vi "reg_visu OPC1.vi"(7 "object_name":string="GM1", 9 "Останов\nпрограммы":bool) -> ()   [LabVIEW 2019]
uses:
  projects/Additivs/Regulators/PROG/GM1_201007/enums/AI.ctl
  Heating/ctl/general_init_client.ctl
  OPC/OPC UA Client.ctl
  <vilib>/OPCUA/controls/OPC UA Client Refnum.ctl
  <vilib>/OPCUA/controls/NodeId.ctl
  <vilib>/OPCUA/controls/NodeIds.ctl
  <vilib>/OPCUA/controls/Subscription ID.ctl
  <vilib>/OPCUA/controls/Write Variant Request.ctl
  <vilib>/OPCUA/controls/Write Status.ctl
  <vilib>/OPCUA/controls/Subscription Data Change.ctl
  <vilib>/OPCUA/controls/Data Type.ctl
  <vilib>/OPCUA/controls/OPC UA StatusCode.ctl
  Database/ctl/Coninfo.ctl
  Inputs/Ctl/AI short.ctl
  Inputs/Ctl/Parameter State.ctl
  Inputs/Ctl/DI short.ctl
  Alarms/Ctl/ALRs_State.ctl
  projects/Additivs/Regulators/PROG/GM1_201007/enums/KFM.ctl
  projects/Additivs/Regulators/PROG/GM1_201007/enums/PAR.ctl
  projects/Additivs/Regulators/PROG/GM1_201007/enums/DI.ctl
  projects/Additivs/Regulators/PROG/GM1_201007/enums/DI_FAST.ctl
  projects/Additivs/Regulators/PROG/GM1_201007/enums/AO.ctl
  projects/Additivs/Regulators/PROG/GM1_201007/enums/DO.ctl
  projects/Additivs/Regulators/PROG/GM1_201007/enums/ALR.ctl
  projects/Additivs/Regulators/PROG/GM1_201007/enums/System.ctl
  ctl/Y_short.ctl
  Inputs/Ctl/Parameter State short.ctl
  ctl/Ys_short.ctl
  <vilib>/picture/picture.llb/imagedata.ctl
  Reg visu/Reg visu.lvclass
  Reg visu/Reg visu.lvclass/Reg visu.ctl
  Inputs/Ctl/ParamColumns.ctl
  531d0f69-163a-4f16-9a14-c53a50917fc8.vi
  cf2ac22c-c8a5-4ec0-ba3c-9dae82546773.vi
  <vilib>/NI/AMC/Create Single Message.vi
  <vilib>/NI/AMC/Update Message Routing Info.vi
  <vilib>/NI/AMC/Read Termination Message.vi
  <vilib>/JDP Science/JSONtext/Find Multiple Items.vi
  <vilib>/JDP Science/JSONtext/String Subset.vi
  <vilib>/JDP Science/JSONtext/support/Strip Quotes and Unescape.vi
  <vilib>/JDP Science/JSONtext/support/Unescape JSON string.vi
  <vilib>/Utility/config.llb/Read Key (String).vi
  <vilib>/OPCUA/client/Multiple Read String Array.vi
  <vilib>/OPCUA/client/Multiple Read ByteString Array.vi
  Reg visu/Run.vi
  Heating/Global stop.vi
  <vilib>/NI/AMC/Send Message.vi
  <vilib>/NI/AMC/Globals.vi
  <vilib>/OPCUA/client/Multiple Read String.vi
  <vilib>/JDP Science/JSONtext/JSON text to Variant.vi
  <vilib>/OPCUA/client/Multiple Write Variant.vi
  <vilib>/JDP Science/JSONtext/Parsing/Parse Full Path or Item Name.vi
  <vilib>/JDP Science/JSONtext/Offset/Find Item Locations by Path.vi
  <vilib>/JDP Science/JSONtext/Get Array Elements.vi
  <vilib>/JDP Science/JSONtext/LVClass Serializer/JSONtext LVClass Serializer.lvclass
  Heating/ctl/Z_State.ctl
  Heating/Heating.lvlib
  Heating/ctl/Y_state.ctl
  Heating/ctl/Y_source.ctl
  Heating/ctl/ZM_State.ctl
  <vilib>/NI/AMC/AMC.lvlib
  <vilib>/OPCUA/NI OPC UA Client.lvlib
  Database/PostgreSQL.lvlib
  <vilib>/Utility/config.llb/NI_LVConfig.lvlib
  projects/Additivs/Regulators/PROG/GM1_201007/enums/Param_h0gm1.lvlib
  Inputs/Inputs.lvlib
  control.lvlib
  OPC/OPC addons.lvlib
  Alarms/Alarms.lvlib
  Heating/ctl/ZY_control.ctl
  Alarms/Ctl/ALR_Status_short.ctl
  Heating/ctl/Y_short.ctl
  Heating/ctl/Z.ctl
  Heating/ctl/ZY_state_short.ctl
  projects/Additivs/Regulators/PROG/GM1_201007/enums/scada_prog_state.ctl
  Heating/ctl/YQ2/YQ2.xctl
  Heating/ctl/Z_OnSwitch/Z_OnSwitch.xctl
  Heating/ctl/ZY_state_OPC.ctl
  7b03969a-a950-4454-9689-61267dd49491.vi
  fdeea6ee-2705-42e7-9783-53477a0f0781.vi
  00ce5b65-c19c-4f2f-b5a6-2d8b920d64b8.vi
  d49def32-a249-4c88-86f5-dd42ff10ee1e.vi
  847353ff-c4dc-4a0d-82d8-8a8c8b1dd027.vi
  96cb8638-67ee-45ab-9e65-4cb433c703bb.vi
  5d0f38f1-9d99-409f-81fc-f0eb7cf3d60e.vi
  fe7cfdb3-b4e0-46ae-bded-47b821cc5e2e.vi
  96416696-a13a-4191-9eaf-5b72f20cf204.vi
  <vilib>/OPCUA/client/Multiple Read Int32 Array.vi
  <vilib>/OPCUA/client/Multiple Read Double Array.vi
  <vilib>/OPCUA/client/Multiple Read UInt32 Array.vi
  <vilib>/OPCUA/client/Multiple Read Bool Array.vi
  Userlib.lvlib
  Heating/ctl/Z_source.ctl
panel:
  in  "HT1 emergency stop":bool caption="Аварийный сброс"
  in  "Reset":bool
  in  "Start":bool
  out "PV 2":dbl(slide) scale=0.0..50.0 scale format="%#_4g"
  in  "tick":u32=100 caption="Время цикла основной программы" min=5 max=1000 step=1
  out "EB3BP1_XQ01":dbl caption="kPa" format="%#.1f"
  in  "AI_enum":T1
  out "CPU %":dbl(slide) scale=0.0..100.0
  in  "password system DB":string
  in  "message name":string="AI redefine"
  in  "process":bool
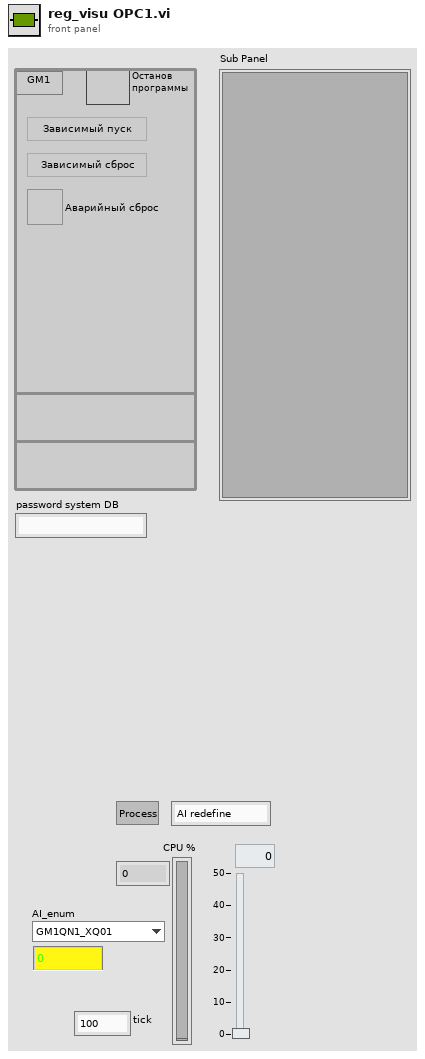
[diagram p1: front panel]
types:
  T1 = typedef "Param_h0gm1.lvlib/AI.ctl" = enum16{"GM1QN1_XQ01", "GM1QN2_XQ01", "GM1QN3_XQ01", "GM1QN4_XQ01", "GM1QN5_XQ01", "GM1QN6_XQ01", "GM1QN7_XQ01", "GM1QN8_XQ01", "GM1QN9_XQ01", "GM1QN10_XQ01", "GM1QN11_XQ01", "GM1QN12_XQ01", "GM1QN13_XQ01", "GM1QN14_XQ01", "GM1QN15_XQ01", "GM1QN16_XQ01", "GM1QN17_XQ01", "GM1QN18_XQ01", "GM1QN19_XQ01", "GM1QN20_XQ01", "GM1QN21_XQ01", "GM1QN22_XQ01", "GM1QN23_XQ01", "GM1QN1_XQ02", "GM1QN2_XQ02", "GM1QN3_XQ02", "GM1QN4_XQ02", "GM1QN5_XQ02", "GM1QN6_XQ02", "GM1QN7_XQ02", "GM1QN8_XQ02", "GM1QN9_XQ02", "GM1QN10_XQ02", "GM1QN11_XQ02", "GM1QN12_XQ02", "GM1QN13_XQ02", "GM1QN14_XQ02", "GM1QN15_XQ02", "GM1QN16_XQ02", "GM1QN17_XQ02", "GM1QN18_XQ02", "GM1QN19_XQ02", "GM1QN20_XQ02", "GM1QN21_XQ02", "GM1QN22_XQ02", "GM1QN23_XQ02"}
  T2 = typedef "Heating.lvlib/general_init_client.ctl" = enum16{"Init Data", "Init TMPs", "Read system DB param", "Read data DB param", "Read OPC param", "Read Enums", "Read Reg param", "Connect to OPC", "Read Param", "Read AI param", "AI references", "AI reorder", "AI reorder1", "AI Descriptions", "AI Descriptions1", "Read DI param", "Read AO param", "Read DO param", "Read ALR param", "Read control param", "Read state param", "Init save progs", "Init ALR Listbox symbols", "Init Y defs", "Init Shared Variables", "Exit"}
  T3 = typedef "AMC.lvlib/Message Queue.ctl" = refnum<queue>
  T4 = typedef "Inputs.lvlib/AI short.ctl" = cluster{"AI":dbl[], "AIState":T5[], "AIALRState":errorcluster[]}
  T5 = typedef "Inputs.lvlib/Parameter State.ctl" = cluster{"code":i32, "visible":bool, "color":u32, "source":string}
  T6 = typedef "NodeIds.ctl" = T7[]
  T7 = typedef "NodeId.ctl" = string
  T8 = typedef "Inputs.lvlib/DI short.ctl" = cluster{"DI":bool[], "DI_State":T5[], "DI_ALRState":errorcluster[]}
  T9 = typedef "Alarms.lvlib/ALRs_State.ctl" = cluster{"ALR not block":bool[], "ALR":bool[], "ALR blocked":bool[], "ALR ON":bool[], "code":i32[], "level":i32[][], "t ms":u32[], "ack state":enum32{"not", "tripped", "reset", "ack"}[], "color":u32[]}
  T10 = typedef "control.lvlib/Y_short.ctl" = cluster{"Y_Source":u8, "Y_SetState":u8, "SP_Set":dbl, "SP":dbl, "PV":dbl, "PV_State":T11, "Y_preSet":dbl, "Y_Set":dbl, "Y":dbl, "Y_State":T11, "YB":bool}
  T11 = typedef "Inputs.lvlib/Parameter State short.ctl" = cluster{"code":i32, "visible":bool, "color":u32}
  T12 = cluster{"connect":bool, "gas":string, "Y_State":T10}
  T13 = cluster{"name":string, "OPC port":string, "security policy":cluster{"message mode":enum16{"None", "Sign", "Sign and Encrypt"}, "security":enum16{"Basic256", "Basic128Rsa15"}}}
  T14 = cluster{"KFM":string[], "PAR":string[], "AI":string[], "DI":string[], "DI_fast":string[], "AO":string[], "DO":string[], "ALR":string[], "System":string[]}
  T15 = typedef "PostgreSQL.lvlib/Coninfo.ctl" = cluster{"host":string, "port":string, "client_encoding":string, "dbname":string, "user":string, "password":string}
  T16 = typedef "OPC addons.lvlib/OPC UA Client.ctl" = cluster{"Client refnum":T17, "Folders":T7[], "node IDs":T6, "subscription IDs":T18[], "requests":T19[], "data change event":refnum<user-event>, "Event Reg":refnum<event-registration>}
  T17 = typedef "OPC UA Client Refnum.ctl" = refnum<k21>
  T18 = typedef "Subscription ID.ctl" = u32
  T19 = typedef "Write Variant Request.ctl" = cluster{"node ID":T7, "value":variant, "timestamp (current time)":timestamp, "node status":T20}
  T20 = typedef "Write Status.ctl" = u32
  T21 = cluster{"object_name":string, "Server":cluster{"name":string, "OPC port":string, "security policy":cluster{"message mode":enum16{"None", "Sign", "Sign and Encrypt"}, "security":enum16{"Basic256", "Basic128Rsa15"}}}, "Enums":cluster{"KFM":string[], "PAR":string[], "AI":string[], "DI":string[], "DI_fast":string[], "AO":string[], "DO":string[], "ALR":string[], "System":string[]}, "OPC UA":T16, "system DB":T15, "AI_SHVR":refnum<k21>, "AI_Names_SHVR":refnum<k21>, "DI_SHVR":refnum<k21>, "DI_Names_SHVR":refnum<k21>, "ALR_state_SHRV":refnum<k21>, "ALR_Descriptions_SHRV":refnum<k21>, "CPU_utilization":refnum<k21>, "AI_refs":refnum<vi>[], "AI_Descriptions":string[], "DI_Descriptions":string[], "ALR_Descriptions":string[]}
  T22 = cluster{"AI_reorder_table":i32[], "AI":dbl[], "AIState":T5[], "AIALRState":errorcluster[], "DI_reorder_table":i32[], "DI":bool[], "DI_State":T5[], "ALR_State":T9, "ALR_Names":string[], "RegsParam":dbl[][], "Regs_Descriptions":string[][], "system msg":string}
  T23 = typedef "NI_LVConfig.lvlib/Config Data RefNum.ctl" = refnum<k1>
  T24 = typedef "Param_h0gm1.lvlib/System.ctl" = enum16{"GM3HT1", "GM3HT2", "EB2TB1", "EB2TB2", "EB2TB3", "EB3TB1", "EB3TB2", "EB3TB3"}
  T25 = typedef "Param_h0gm1.lvlib/ALR.ctl" = enum16{"GM1JBA1JA1_CONN", "GM1JBA1JA2_CONN", "GM1JBA2JA1_CONN", "GM1JBA2JA2_CONN", "GM1JBA3JA1_CONN", "GM1QN1XQ01_SERR", "GM1QN2XQ01_SERR", "GM1QN3XQ01_SERR", "GM1QN4XQ01_SERR", "GM1QN5XQ01_SERR", "GM1QN6XQ01_SERR", "GM1QN7XQ01_SERR", "GM1QN8XQ01_SERR", "GM1QN9XQ01_SERR", "GM1QN10XQ01_SERR", "GM1QN11XQ01_SERR", "GM1QN12XQ01_SERR", "GM1QN13XQ01_SERR", "GM1QN14XQ01_SERR", "GM1QN15XQ01_SERR", "GM1QN16XQ01_SERR", "GM1QN17XQ01_SERR", "GM1QN18XQ01_SERR", "GM1QN19XQ01_SERR", "GM1QN20XQ01_SERR", "GM1QN21XQ01_SERR", "GM1QN22XQ01_SERR", "GM1QN23XQ01_SERR"}
  T26 = typedef "Param_h0gm1.lvlib/DO.ctl" = enum16{"GM1FZ1_YB47"}
  T27 = typedef "Param_h0gm1.lvlib/AO.ctl" = enum16{"GM1QN1_YQ01", "GM1QN2_YQ01", "GM1QN3_YQ01", "GM1QN4_YQ01", "GM1QN5_YQ01", "GM1QN6_YQ01", "GM1QN7_YQ01", "GM1QN8_YQ01", "GM1QN9_YQ01", "GM1QN10_YQ01", "GM1QN11_YQ01", "GM1QN12_YQ01", "GM1QN13_YQ01", "GM1QN14_YQ01", "GM1QN15_YQ01", "GM1QN16_YQ01", "GM1QN17_YQ01", "GM1QN18_YQ01", "GM1QN19_YQ01", "GM1QN20_YQ01", "GM1QN21_YQ01", "GM1QN22_YQ01", "GM1QN23_YQ01"}
  T28 = typedef "Param_h0gm1.lvlib/DI_FAST.ctl" = enum16{"W1.KF_XB01", "W1.KF_XB02", "W1.KF_XB03", "W1.KF_XB04", "W1.KF_XB05", "W1.KF_XB06", "W1.KF_XB07", "W1.KF_XB08", "W1.KF_XB09", "W1.KF_XB10", "W1.KF_XB11", "W1.KF_XB12", "W1.KF_XB13", "W1.KF_XB14", "W1.KF_XB15", "W1.KF_XB16"}
  T29 = typedef "Param_h0gm1.lvlib/DI.ctl" = enum16{"GM1FZ1_XB19"}
  T30 = typedef "Param_h0gm1.lvlib/PAR.ctl" = enum16{"GM1QN1_alr_value", "GM1QN1_auto_value", "GM1QN1_output_set_time", "GM1QN1_group", "GM1QN1_process_gas", "GM1QN2_alr_value", "GM1QN2_auto_value", "GM1QN2_output_set_time", "GM1QN2_group", "GM1QN2_process_gas", "GM1QN3_alr_value", "GM1QN3_auto_value", "GM1QN3_output_set_time", "GM1QN3_group", "GM1QN3_process_gas", "GM1QN4_alr_value", "GM1QN4_auto_value", "GM1QN4_output_set_time", "GM1QN4_group", "GM1QN4_process_gas", "GM1QN5_alr_value", "GM1QN5_auto_value", "GM1QN5_output_set_time", "GM1QN5_group", "GM1QN5_process_gas", "GM1QN6_alr_value", "GM1QN6_auto_value", "GM1QN6_output_set_time", "GM1QN6_group", "GM1QN6_process_gas", "GM1QN7_alr_value", "GM1QN7_auto_value", "GM1QN7_output_set_time", "GM1QN7_group", "GM1QN7_process_gas", "GM1QN8_alr_value", "GM1QN8_auto_value", "GM1QN8_output_set_time", "GM1QN8_group", "GM1QN8_process_gas", "GM1QN9_alr_value", "GM1QN9_auto_value", "GM1QN9_output_set_time", "GM1QN9_group", "GM1QN9_process_gas", "GM1QN10_alr_value", "GM1QN10_auto_value", "GM1QN10_output_set_time", "GM1QN10_group", "GM1QN10_process_gas", "GM1QN11_alr_value", "GM1QN11_auto_value", "GM1QN11_output_set_time", "GM1QN11_group", "GM1QN11_process_gas", "GM1QN12_alr_value", "GM1QN12_auto_value", "GM1QN12_output_set_time", "GM1QN12_group", "GM1QN12_process_gas", "GM1QN13_alr_value", "GM1QN13_auto_value", "GM1QN13_output_set_time", "GM1QN13_group", "GM1QN13_process_gas", "GM1QN14_alr_value", "GM1QN14_auto_value", "GM1QN14_output_set_time", "GM1QN14_group", "GM1QN14_process_gas", "GM1QN15_alr_value", "GM1QN15_auto_value", "GM1QN15_output_set_time", "GM1QN15_group", "GM1QN15_process_gas", "GM1QN16_alr_value", "GM1QN16_auto_value", "GM1QN16_output_set_time", "GM1QN16_group", "GM1QN16_process_gas", "GM1QN17_alr_value", "GM1QN17_auto_value", "GM1QN17_output_set_time", "GM1QN17_group", "GM1QN17_process_gas", "GM1QN18_alr_value", "GM1QN18_auto_value", "GM1QN18_output_set_time", "GM1QN18_group", "GM1QN18_process_gas", "GM1QN19_alr_value", "GM1QN19_auto_value", "GM1QN19_output_set_time", "GM1QN19_group", "GM1QN19_process_gas", "GM1QN20_alr_value", "GM1QN20_auto_value", "GM1QN20_output_set_time", "GM1QN20_group", "GM1QN20_process_gas", "GM1QN21_alr_value", "GM1QN21_auto_value", "GM1QN21_output_set_time", "GM1QN21_group", "GM1QN21_process_gas", "GM1QN22_alr_value", "GM1QN22_auto_value", "GM1QN22_output_set_time", "GM1QN22_group", "GM1QN22_process_gas", "GM1QN23_alr_value", "GM1QN23_auto_value", "GM1QN23_output_set_time", "GM1QN23_group", "GM1QN23_process_gas"}
  T31 = typedef "Param_h0gm1.lvlib/KFM.ctl" = enum16{"GM1KF1_A1", "GM1JBA1_JA1", "GM1JBA1_JA2", "GM1JBA2_JA1", "GM1JBA2_JA2", "GM1JBA3_JA1"}
  T32 = cluster{"message mode":enum16{"None", "Sign", "Sign and Encrypt"}, "security":enum16{"Basic256", "Basic128Rsa15"}}
  T33 = typedef "OPC addons.lvlib/OPC tag.ctl" = cluster{"name":string, "data type":T34, "access level":T35, "description":string, "period":T36}
  T34 = typedef "Data Type.ctl" = u16
  T35 = typedef "OPC addons.lvlib/Access level.ctl" = enum16{"none", "read-only", "write-only", "read/write"}
  T36 = typedef "OPC addons.lvlib/Period.ctl" = enum16{"on_load", "100 ms", "500 ms", "1 s"}
  T37 = cluster{"sampling interval":dbl, "queue size":u32, "discard oldest":bool, "data change filter":cluster{"trigger":enum32{"Status", "StatusValue", "StatusValueTimestamp"}, "deadband type":enum32{"None", "Absolute", "Percent"}, "deadband value":dbl}}[]
  T38 = cluster{"Read Access":enum8{"Allowed", "Required", "None"}, "Write Access":enum8{"Allowed", "Required", "None"}}
  T39 = typedef "OPC UA StatusCode.ctl" = u32
  T40 = cluster{"node ID":T7, "values ":string[], "timestamp":timestamp, "status":T39}[]
  T41 = cluster{"node ID":T7, "values ":string[], "timestamp":timestamp, "status":T39}
  T42 = cluster{"node ID":T7, "values ":u8[][], "timestamp":timestamp, "status":T39}[]
  T43 = cluster{"node ID":T7, "values ":u8[][], "timestamp":timestamp, "status":T39}
  T44 = typedef "Heating.lvlib/ZY_control.ctl" = cluster{"Z_HSw":u8, "Z_HSetState":T45, "Y_HSw":u8, "Y_HSetState":T46, "SP":dbl, "Y_H":dbl, "Reset_ALR":bool}
  T45 = typedef "Heating.lvlib/Z_State.ctl" = enum8{"initialization", "alarm", "disabled", "not ready", "stop ready", "reserv", "switched off", "reserv2", "switched on", "check", "on min", "decrease out", "on", "increase out", "on max"}
  T46 = typedef "Heating.lvlib/Y_state.ctl" = enum8{"initialize", "alarm", "min", "stop", "hand", "auto", "max"}
  T47 = typedef "Heating.lvlib/ZY_state_short.ctl" = cluster{"Z":T48, "Y":T51, "ALR_Status":T53[]}
  T48 = typedef "Heating.lvlib/Z.ctl" = cluster{"Z_Source":T49, "Z_SetState":T45, "Z_State":T45, "Z_State_T":u32, "ZM_State":T50, "ZM_State_T":u32, "ALR  L1":bool, "ALR  L2":bool, "HH_run":u64}
  T49 = typedef "Heating.lvlib/Z_source.ctl" = enum8{"initialize", "local disabled", "local hand", "hand", "auto", "dist"}
  T50 = typedef "Heating.lvlib/ZM_State.ctl" = enum8{"initialization", "stop", "start_cmd", "contactor_on_cmd", "heating", "on", "stop_cmd", "power_down", "contactor_off_cmd", "cooling", "restart_delay"}
  T51 = typedef "Heating.lvlib/Y_short.ctl" = cluster{"Y_Source":T52, "Y_SetState":T46, "SP_Set":dbl, "SP":dbl, "PV":dbl, "Y_Set":dbl, "Y":dbl, "Y_State":T11, "YB":bool}
  T52 = typedef "Heating.lvlib/Y_source.ctl" = enum8{"initialize", "local disabled", "local hand", "hand", "auto", "dist"}
  T53 = typedef "Alarms.lvlib/ALR_Status_short.ctl" = cluster{"status":bool, "code":i32, "level":i32}
  T54 = cluster{"connect":bool, "gas":string, "Y_State":T10}[]
  T55 = typedef "imagedata.ctl" = cluster{"image type":i32, "image depth":i32, "image":u8[], "mask":u8[], "colors":u32[], "Rectangle":cluster{"left":i16, "top":i16, "right":i16, "bottom":i16}}
  T56 = typedef "AMC.lvlib/Message.ctl" = cluster{"name":string, "value":string, "attributes":T57, "receiver host":string, "receiver process":string, "source host":string, "source process":string, "priority message":bool, "acknowledge message":bool}
  T57 = typedef "Tools_KeyedArray.lvlib/KeyedArray.ctl" = cluster{"keys":string[], "values":string[]}
  T58 = cluster{"node ID":T7, "value ":string, "timestamp":timestamp, "status":T39}[]
  T59 = typedef "Inputs.lvlib/ParamColumns.ctl" = enum16{"value", "value_range_min", "value_range_max", "d", "fname", "value_units", "fcode", "fcodef", "fcode_full"}
  T60 = typedef "Param_h0gm1.lvlib/scada_prog_state.ctl" = enum16{"ReadAIParam", "ReadAIParam1", "ReadDIParam", "AI", "AI1", "AIValues", "AIValues1", "DI", "DiValues", "Alarms", "Messages", "TB1", "TB2", "TB3", "Control EB3", "Outputs", "Exit"}
  T61 = cluster{"connect":bool, "Z_Source":T52, "Z_State_heating":T45}
  T62 = typedef "Heating.lvlib/ZY_state_OPC.ctl" = cluster{"Z":cluster{"Z_Source":u8, "Z_SetState":u8, "Z_State":u8, "Z_State_T":u32, "ZM_State":u8, "ZM_State_T":u32, "ALR  L1":bool, "ALR  L2":bool, "HH_run":i32}, "Y":cluster{"Y_Source":u8, "Y_SetState":u8, "SP_Set":dbl, "SP":dbl, "PV":dbl, "Y_Set":dbl, "Y":dbl, "Y_State":cluster{"code":i32, "visible":bool, "color":u32}, "YB":bool}, "ALR_Status":cluster{"status":bool, "code":i32, "level":i32}[]}
  T63 = typedef "Heating.lvlib/ZY_state_short.ctl" = cluster{"Z":T64, "Y":T51, "ALR_Status":T53[]}
  T64 = typedef "Heating.lvlib/Z.ctl" = cluster{"Z_Source":T52, "Z_SetState":T45, "Z_State":T45, "Z_State_T":u32, "ZM_State":T50, "ZM_State_T":u32, "ALR  L1":bool, "ALR  L2":bool, "HH_run":i32}
  T65 = cluster{"node ID":T7, "values ":dbl[], "timestamp":timestamp, "status":T39}[]
  T66 = cluster{"node ID":T7, "values ":i32[], "timestamp":timestamp, "status":T39}[]
  T67 = cluster{"node ID":T7, "values ":dbl[], "timestamp":timestamp, "status":T39}
  T68 = cluster{"node ID":T7, "values ":i32[], "timestamp":timestamp, "status":T39}
  T69 = cluster{"node ID":T7, "values ":bool[], "timestamp":timestamp, "status":T39}[]
  T70 = cluster{"node ID":T7, "values ":bool[], "timestamp":timestamp, "status":T39}
  T71 = cluster{"node ID":T7, "values ":u32[], "timestamp":timestamp, "status":T39}[]
  T72 = cluster{"node ID":T7, "values ":u32[], "timestamp":timestamp, "status":T39}
  T73 = cluster{"node ID":T7, "value ":string, "timestamp":timestamp, "status":T39}
  T74 = typedef "Heating.lvlib/ZY_state_short.ctl" = cluster{"Z":T64, "Y":T75, "ALR_Status":T53[]}
  T75 = typedef "Heating.lvlib/Y_short.ctl" = cluster{"Y_Source":T52, "Y_SetState":T46, "SP_Set":dbl, "SP":dbl, "PV":dbl, "Y":dbl, "Y_State":T11, "YB":bool}
  T76 = enum32{"invalid app kind", "Development System", "Run Time System", "Student Edition", "Embedded LabVIEW", "Evaluation", "Custom"}
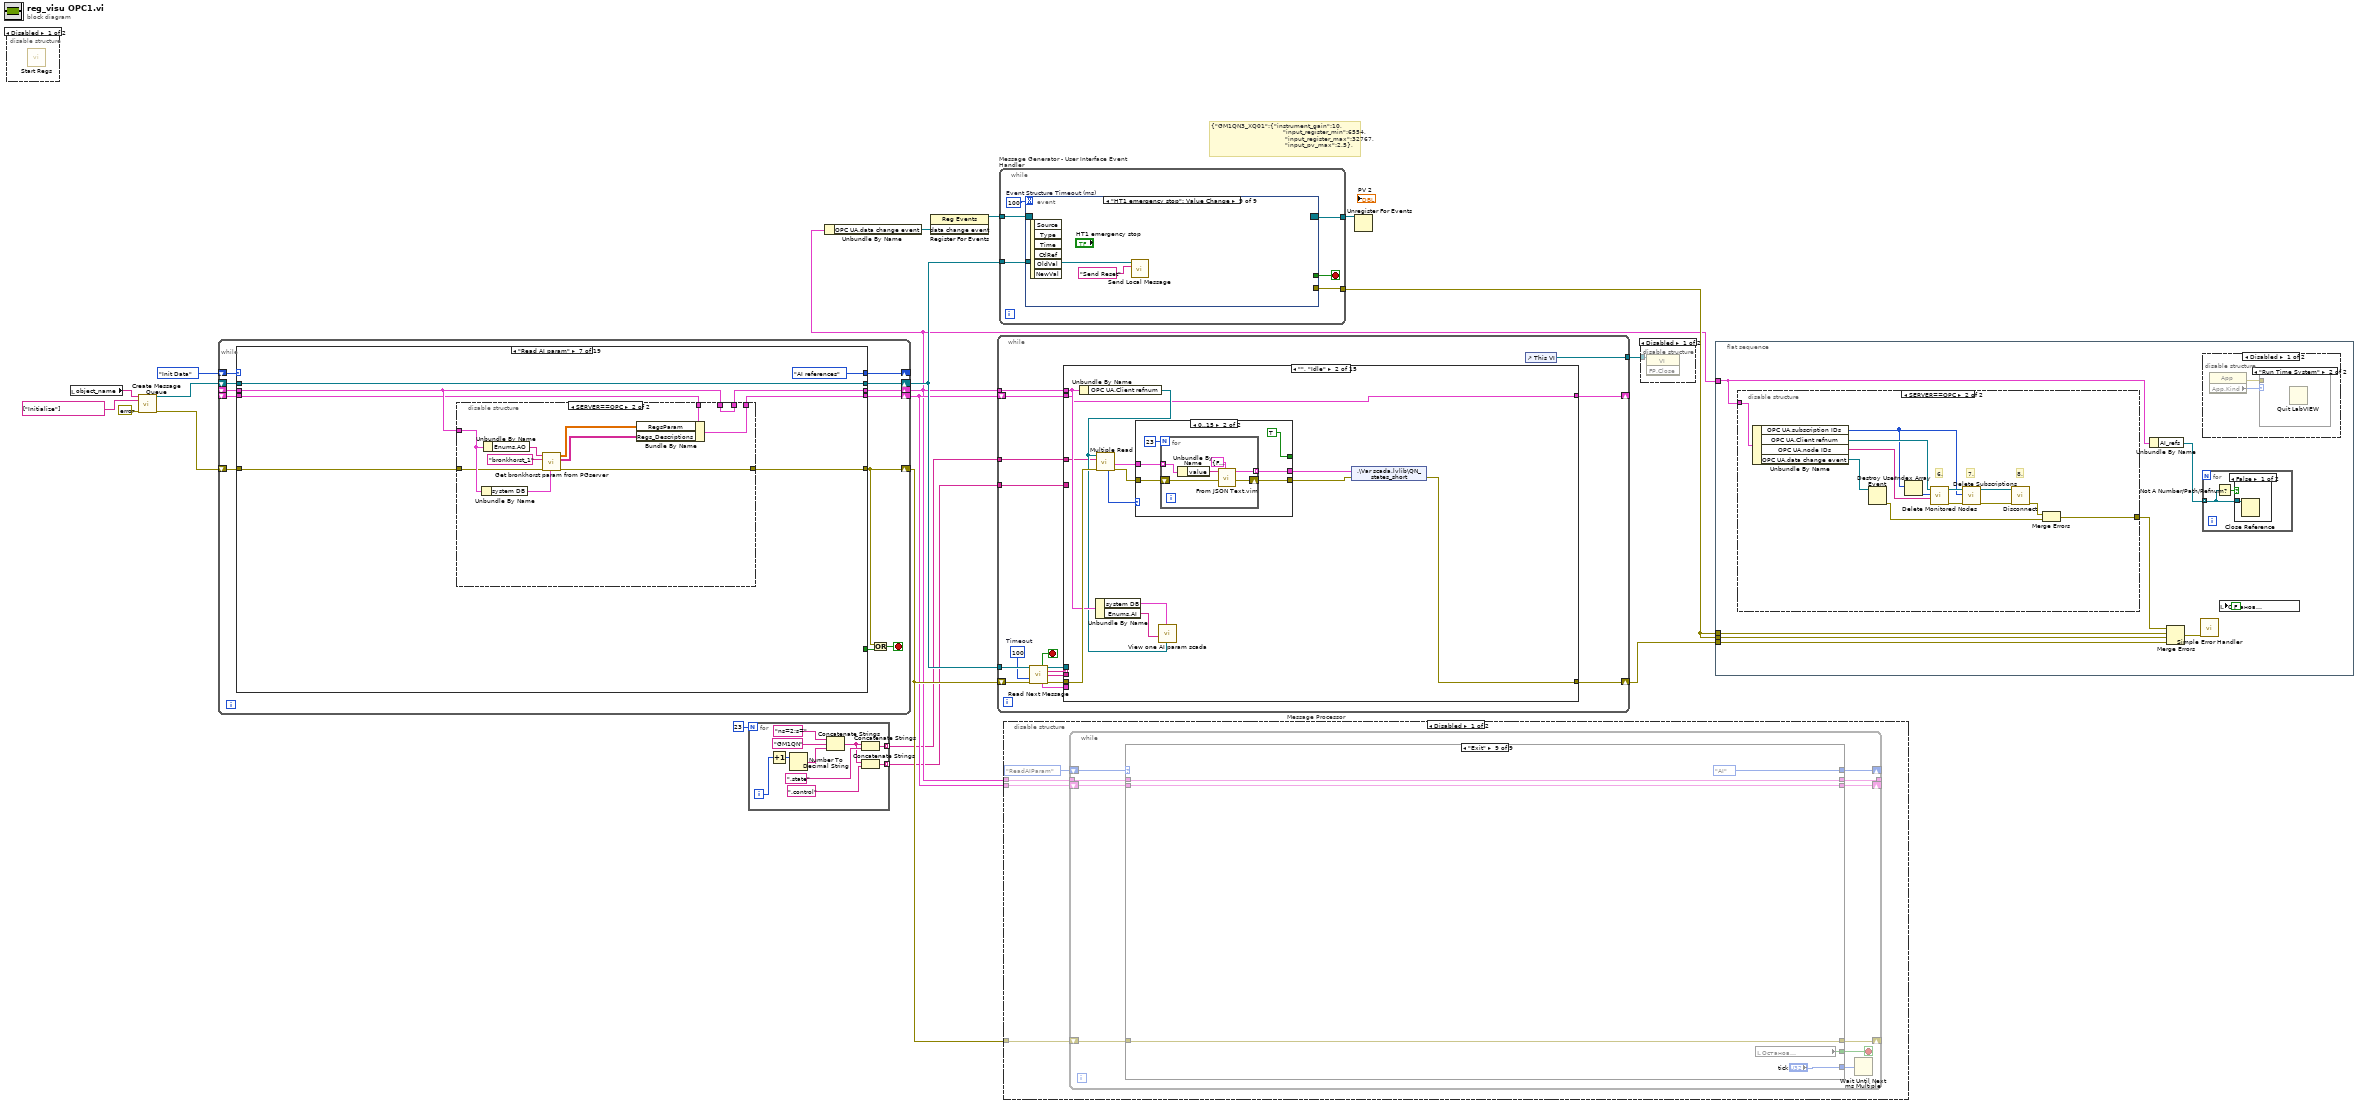
[diagram p0: block diagram]
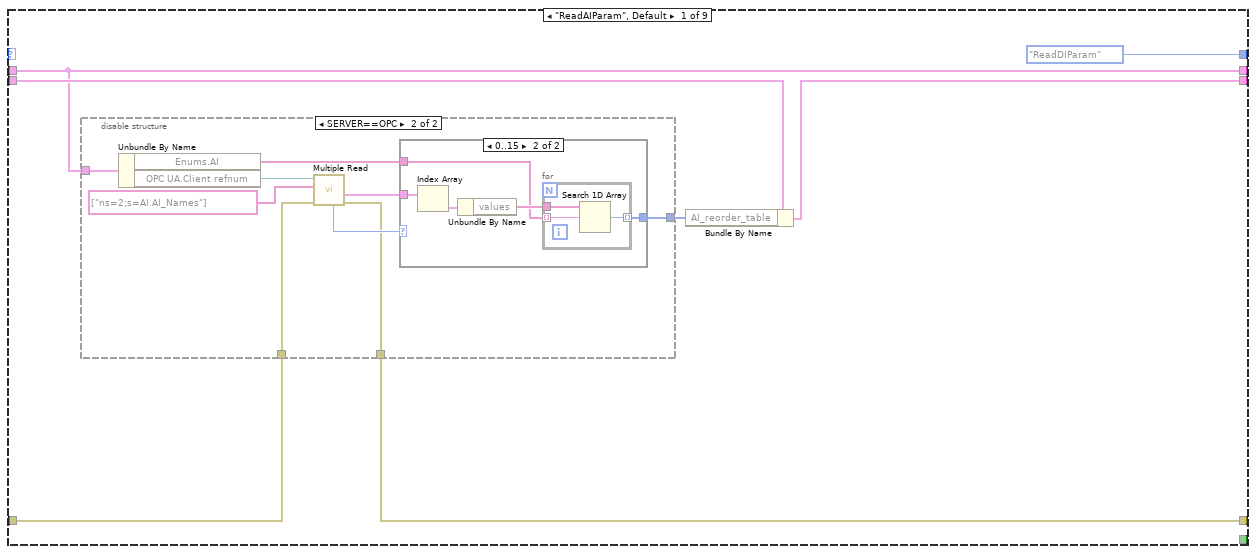
[diagram p3: hidden frame]
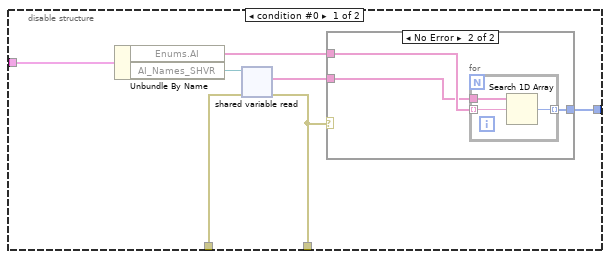
[diagram p4: hidden frame]
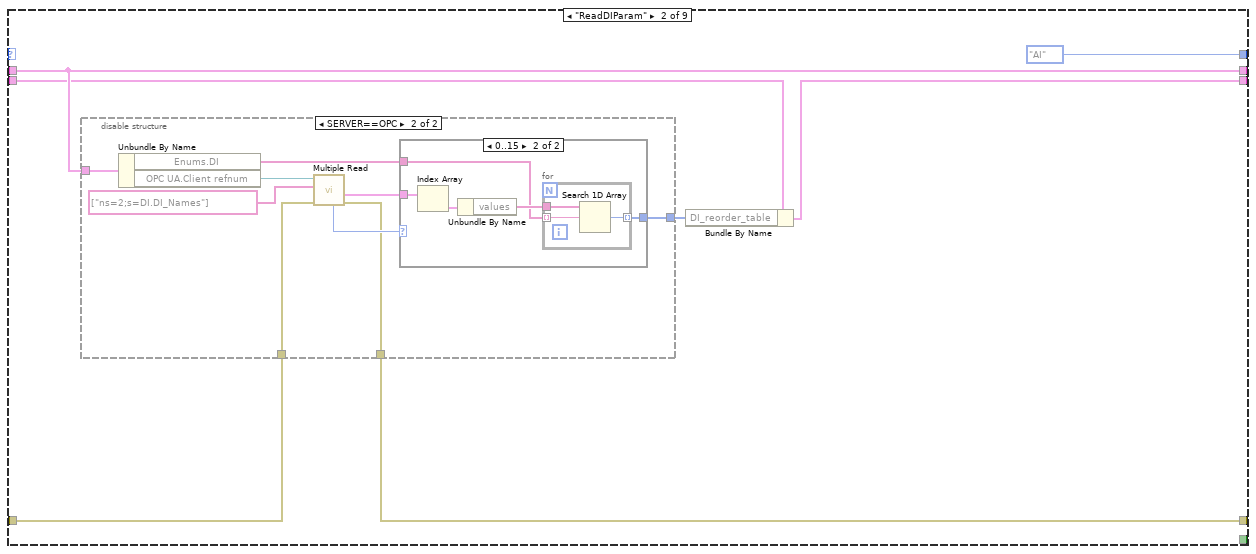
[diagram p7: hidden frame]
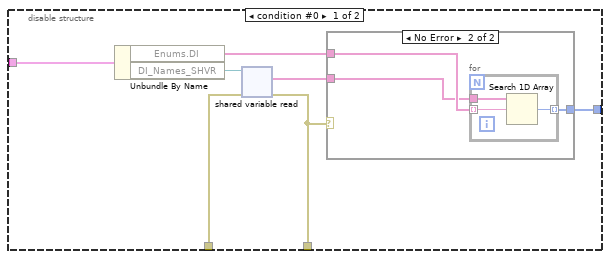
[diagram p8: hidden frame]
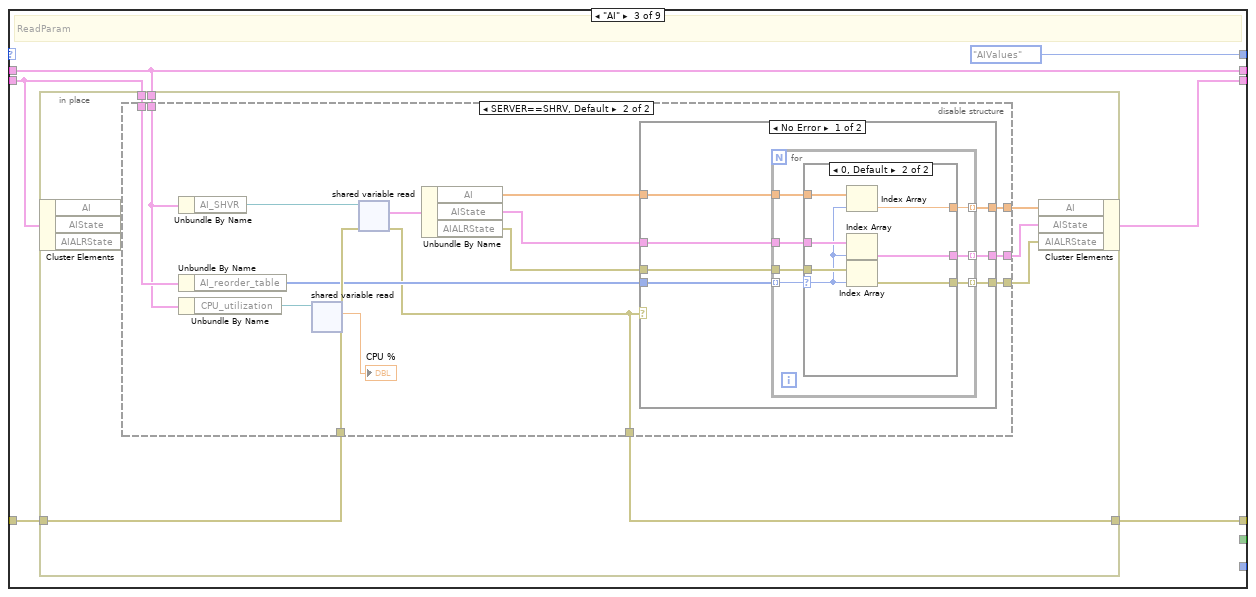
[diagram p11: hidden frame]
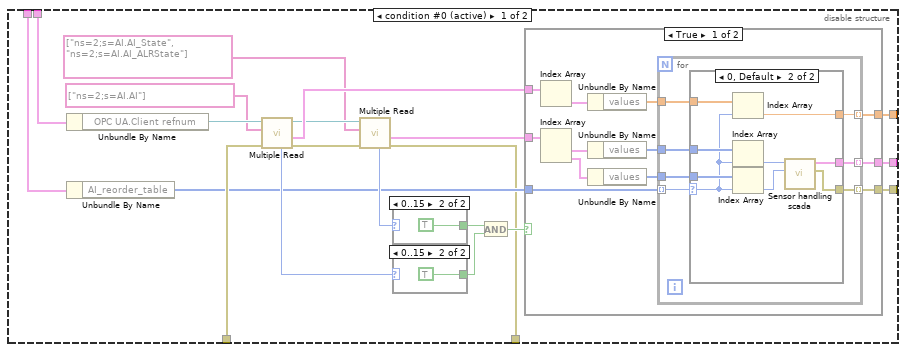
[diagram p12: hidden frame]
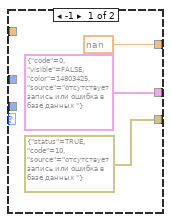
[diagram p15: hidden frame]
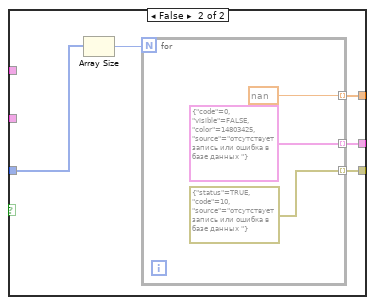
[diagram p16: hidden frame]
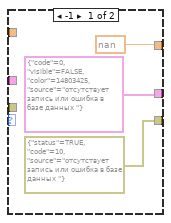
[diagram p17: hidden frame]
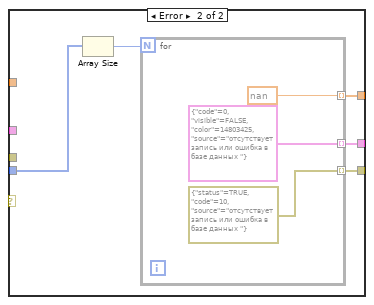
[diagram p18: hidden frame]
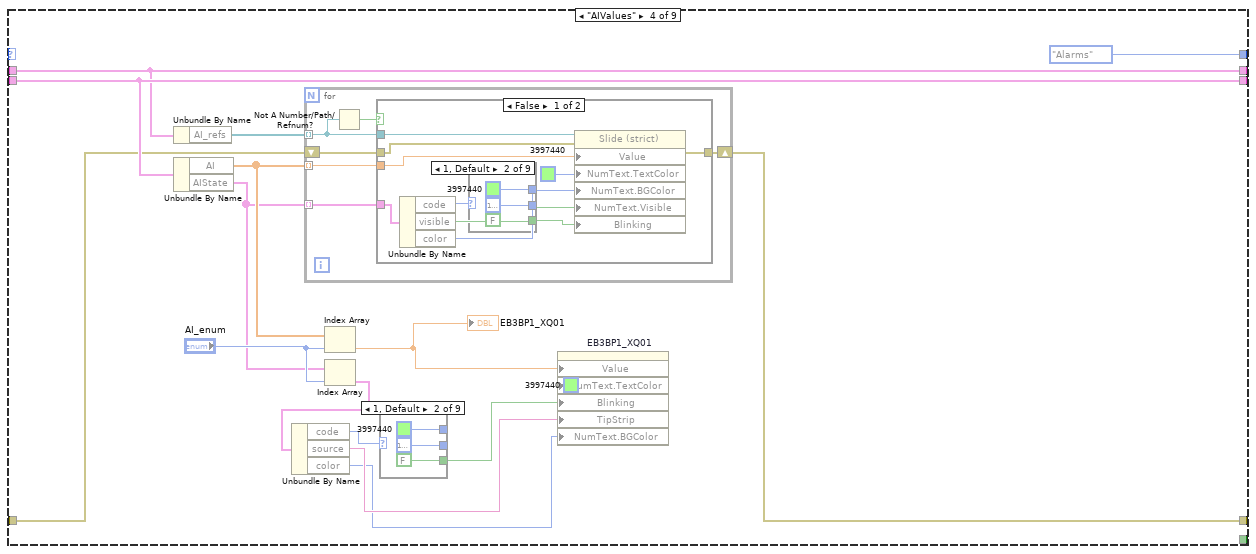
[diagram p19: hidden frame]
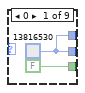
[diagram p20: hidden frame]
diagram:
  # "{\"GM1QN3_XQ01\":{\"instrument_gain\":10,\n                                    \"input_register_min\":6554,\n                                     \"input_register_max\":32767,\n                                     \"input_pv_max\":2.5},"
  n1 = disable-structure shown="Disabled" {
    frame Disabled {
      n2 = call "Start Regs.vi"() -> ()  [unwired: 11 in, 1 out]
    }
    frame Enabled {
    }
  }
  n3 = local read "object_name"() -> (w17:string)
  n4 = call <vilib>:"Create Message Queue.vi"("message queue name"=w17, "initial message names"=string[] ["Initialize"], "error in"=errorcluster {"status"=FALSE, "code"=0, "source"=""}) -> ("message queue out"=w10:T3, "error out"=w12:errorcluster)  [unwired: 11 in]
  n5 = while {
    shift-right: [w20] -> w6
    shift-left: w12 -> [w28]
    shift-right: [w31] -> w4
    shift-left: _ -> [w29]
    shift-right: [w27] -> _
    shift-left: general_init_client."Init Data" -> [w30]
    shift-right: [w24] -> w5
    shift-left: _ -> [w23]
    shift-right: [w21] -> w9
    shift-left: w10 -> [w22]
    stop <- w25 stop-if-true
    n6 = case shown="\"Read AI param\"" w30 {
      tunnel: [w50 w68 w70 w113 w176 w202 w239 w279 w291 w336 w356 w392 w435 w463 w493 w499 w516 w577 w580] -> w20
      selector: w30 -> [_ _ _ _ _ _ _ _ _ _ _ _ _ _ _ _ _ _ w583]
      tunnel: [w51 w66 w105 w114 w196 w203 w240 w276 w290 w330 w358 w393 w437 w465 w495 w512 w528 w578 w581] -> w31
      tunnel: w29 -> [_ w66 w104 w112 w198 w201 w238 w275 w290 w329 w355 w386 w434 w462 w495 w512 w528 w578 w581]
      tunnel: w28 -> [w50 w68 w106 w115 w186 w205 w241 w279 w292 w337 w359 w387 w438 w466 w492 w499 w518 w577 w580]
      tunnel: [general_init_client."Init TMPs" general_init_client."Read system DB param" general_init_client."Read data DB param" general_init_client."Read Enums" general_init_client."Read OPC param" general_init_client."Read Param" general_init_client."AI references" general_init_client."AI reorder" general_init_client."AI Descriptions" general_init_client."Read DI param" general_init_client."Read ALR param" general_init_client."Read control param" general_init_client."Read state param" general_init_client."Init Shared Variables" general_init_client."Init ALR Listbox symbols" general_init_client."Init Y defs" general_init_client."Exit" general_init_client."Init Data" w582] -> w27
      tunnel: [_ _ _ _ _ _ _ _ _ _ _ _ _ _ _ _ _ TRUE _] -> w26
      tunnel: [w48 w61 w108 w117 w200 w206 w237 w280 w289 w333 w357 w385 w436 w464 w498 w515 w527 w575 w585] -> w24
      tunnel: w23 -> [w48 _ w108 w117 w200 w206 w236 w280 w288 w333 w357 w384 w436 w464 w498 w515 w527 w575 w585]
      tunnel: w22 -> [w49 w67 w107 w116 w175 w204 w243 w282 w295 w342 w361 w395 w440 w468 w497 w514 w521 w574 w584]
      tunnel: [w49 w67 w107 w116 w175 w204 w243 w282 w295 w342 w361 w395 w440 w468 w497 w514 w521 w574 w584] -> w21
      frame "Init Data" {
        w33 = string[] []  # DI_Descriptions
        w34 = string[] []  # AI_Descriptions
        w32 = string[] []  # ALR_Descriptions
        w35 = refnum<vi>[] []  # AI_refs
        w36 = refnum<k21> refnum  # CPU_utilization
        w38 = refnum<k21> refnum  # ALR_Descriptions_SHRV
        w39 = refnum<k21> refnum  # ALR_state_SHRV
        w40 = refnum<k21> refnum  # DI_Names_SHVR
        w41 = refnum<k21> refnum  # DI_SHVR
        w42 = T13 {"name"="H1GM2", "OPC port"="49580", "security policy"={"message mode"=enum."None", "security"=enum."Basic256"}}  # Server
        w43 = refnum<k21> refnum  # AI_Names_SHVR
        w44 = refnum<k21> refnum  # AI_SHVR
        w46 = T14 {"KFM"=[], "PAR"=[], "AI"=[], "DI"=[], "DI_fast"=[], "AO"=[], "DO"=[], "ALR"=[], "System"=[]}  # Enums
        w47 = T15 {"host"="localhosh", "port"="5432", "client_encoding"="LATIN1", "dbname"="system", "user"="postgres", "password"=""}  # system DB
        w45 = T16 {"Client refnum"="", "Folders"=[], "node IDs"=[], "subscription IDs"=[], "requests"=[], "data change event"=refnum, "Event Reg"=refnum}  # OPC UA
        n7 = Bundle("object_name"="object_name", "Server"=w42, "Enums"=w46, "OPC UA"=w45, "system DB"=w47, "AI_SHVR"=w44, "AI_Names_SHVR"=w43, "DI_SHVR"=w41, "DI_Names_SHVR"=w40, "ALR_state_SHRV"=w39, "ALR_Descriptions_SHRV"=w38, "CPU_utilization"=w36, "AI_refs"=w35, "AI_Descriptions"=w34, "DI_Descriptions"=w33, "ALR_Descriptions"=w32) -> (w51:T21)  [unwired: 1 in]
      }
      frame "Init TMPs" {
        w53 = string[][] []  # Regs_Descriptions
        w55 = dbl[][] []  # RegsParam
        w56 = string[] []  # ALR_Names
        w57 = T9 {"ALR not block"=[], "ALR"=[], "ALR blocked"=[], "ALR ON"=[], "code"=[], "level"=[], "t ms"=[], "ack state"=[], "color"=[]}  # ALR_State
        w54 = ""  # system msg
        w58 = i32[] []  # DI_reorder_table
        w60 = i32[] []  # AI_reorder_table
        (unwired) dbl[] []  # AO
        (unwired) dbl[][] []  # AOP
        (unwired) bool[] []  # DO
        (unwired) i32[][] []  # DOP
        (unwired) i32[] []  # PAR_I
        (unwired) dbl[] []  # PAR
        (unwired) bool[] []  # connect
        w65 = T5[] []  # AIState
        w64 = errorcluster[] []  # AIALRState
        w63 = bool[] []  # DI
        (unwired) dbl[][] []  # DIP
        w62 = T5[] []  # DI_State
        (unwired) dbl[][] []  # AIP
        w59 = dbl[] []  # AI
        n8 = Bundle("AI_reorder_table"=w60, "AI"=w59, "AIState"=w65, "AIALRState"=w64, "DI_reorder_table"=w58, "DI"=w63, "DI_State"=w62, "ALR_State"=w57, "ALR_Names"=w56, "RegsParam"=w55, "Regs_Descriptions"=w53, "system msg"=w54) -> (w61:T22)  [unwired: 1 in]
      }
      frame "Read system DB param" {
        w81 = "System_DB" ("key")
        n9 = disable-structure shown="Default" {
          disable-tunnel: [w110 w111] -> w71
          frame condition #0 (active) {
            n10 = call <vilib>:"Application Directory.vi"() -> ("Application Directory"=w110:path)
          }
          frame condition #1 {
            n11 = call <vilib>:"Dflt Data Dir.vi"() -> ("App:Default Data Directory"=w111:path)
          }
        }
        n12 = Unbundle By Name(w104) -> ("system DB"=w95:T15)
        n13 = Unbundle By Name(w95) -> ("host"=w94:string, "port"=w93:string, "client_encoding"=w90:string, "dbname"=w85:string, "user"=w80:string)
        n14 = Build Path(base path=w71, name or relative path=path "DBp.ini" ("configuration file path")) -> (appended path=w103:path)
        n15 = call <vilib>:"Open Config Data.vi"("error in (no error)"=w106, "configuration file path"=w103) -> ("error out"=w101:errorcluster, "refnum"=w100:T23)  [unwired: 7 in, 1 out]
        n16 = call-poly <vilib>:"Read Key.vi"("section"=w81, "error in (no error)"=w101, "default value"=w94, "key"="host", "refnum"=w100) -> ("error out"=w96:errorcluster, "value"=w73:string, "refnum out"=w97:T23)  [unwired: 3 in, 1 out]
        n17 = call-poly <vilib>:"Read Key.vi"("section"=w81, "error in (no error)"=w96, "default value"=w93, "key"="port", "refnum"=w97) -> ("error out"=w89:errorcluster, "value"=w74:string, "refnum out"=w91:T23)  [unwired: 3 in, 1 out]
        n18 = call-poly <vilib>:"Read Key.vi"("section"=w81, "error in (no error)"=w89, "default value"=w90, "key"="clint_encoding", "refnum"=w91) -> ("error out"=w86:errorcluster, "value"=w75:string, "refnum out"=w87:T23)  [unwired: 3 in, 1 out]
        n19 = call-poly <vilib>:"Read Key.vi"("section"=w81, "error in (no error)"=w86, "default value"=w85, "key"="dbname", "refnum"=w87) -> ("error out"=w82:errorcluster, "value"=w76:string, "refnum out"=w83:T23)  [unwired: 3 in, 1 out]
        n20 = call-poly <vilib>:"Read Key.vi"("section"=w81, "error in (no error)"=w82, "default value"=w80, "key"="user", "refnum"=w83) -> ("error out"=w78:errorcluster, "value"=w77:string, "refnum out"=w79:T23)  [unwired: 3 in, 1 out]
        n21 = call <vilib>:"Close Config Data.vi"("error in (no error)"=w78, "refnum"=w79) -> ("error out"=w70:errorcluster)  [unwired: 8 in, 1 out]
        n22 = Bundle By Name(cluster=w104, "system DB.user"=w77, "system DB.dbname"=w76, "system DB.client_encoding"=w75, "system DB.port"=w74, "system DB.host"=w73, "system DB.password"="password system DB") -> (w105:T21)
      }
      frame "Read data DB param" {
        n23 = disable-structure shown="SERVER==OPC" {
          disable-tunnel: w115 -> [w158 w164]
          disable-tunnel: w112 -> [w156 w163]
          disable-tunnel: [w154 w163] -> w114
          disable-tunnel: [w123 w164] -> w113
          disable-tunnel: w112 -> [w150 _]
          frame condition #0 (active) {
            w135 = "Server" ("key")
            n24 = disable-structure shown="Default" {
              disable-tunnel: [w161 w162] -> w153
              frame condition #0 (active) {
                n25 = call <vilib>:"Application Directory.vi"() -> ("Application Directory"=w161:path)
              }
              frame condition #1 {
                n26 = call <vilib>:"Dflt Data Dir.vi"() -> ("App:Default Data Directory"=w162:path)
              }
            }
            n27 = Unbundle By Name(w150) -> ("Server.name"=w152:string, "Server.OPC port"=w149:string, "Server.security policy.message mode"=w138:enum16{"None", "Sign", "Sign and Encrypt"}, "Server.security policy.security"=w133:enum16{"Basic256", "Basic128Rsa15"})
            n28 = Build Path(base path=w153, name or relative path=path "DBp.ini" ("configuration file path")) -> (appended path=w160:path)
            n29 = call <vilib>:"Open Config Data.vi"("error in (no error)"=w158, "configuration file path"=w160) -> ("error out"=w137:errorcluster, "refnum"=w157:T23)  [unwired: 7 in, 1 out]
            n30 = call <userlib>:"Get Strings from Enum__ogtk.vi"("error in (no error)"=w137, "Enum"=w138) -> ("error out"=w127:errorcluster, "String Value"=w136:string)  [unwired: 6 in, 2 out]
            n31 = call <userlib>:"Get Strings from Enum__ogtk.vi"("error in (no error)"=w137, "Enum"=w133) -> ("error out"=w128:errorcluster, "String Value"=w134:string)  [unwired: 6 in, 2 out]
            n32 = call-poly <vilib>:"Read Key.vi"("section"=w135, "error in (no error)"=w137, "default value"=w152, "key"="name", "refnum"=w157) -> ("error out"=w146:errorcluster, "value"=w151:string, "refnum out"=w147:T23)  [unwired: 3 in, 1 out]
            n33 = call-poly <vilib>:"Read Key.vi"("section"=w135, "error in (no error)"=w146, "default value"=w149, "key"="OPC port", "refnum"=w147) -> ("error out"=w145:errorcluster, "value"=w144:string, "refnum out"=w143:T23)  [unwired: 3 in, 1 out]
            n34 = call-poly <vilib>:"Read Key.vi"("section"=w135, "error in (no error)"=w145, "default value"=w136, "key"="message mode", "refnum"=w143) -> ("error out"=w140:errorcluster, "value"=w130:string, "refnum out"=w142:T23)  [unwired: 3 in, 1 out]
            n35 = call-poly <vilib>:"Read Key.vi"("section"=w135, "error in (no error)"=w140, "default value"=w134, "key"="security ", "refnum"=w142) -> ("error out"=w139:errorcluster, "value"=w129:string, "refnum out"=w141:T23)  [unwired: 3 in, 1 out]
            n36 = call <vilib>:"Close Config Data.vi"("error in (no error)"=w139, "refnum"=w141) -> ("error out"=w124:errorcluster)  [unwired: 8 in, 1 out]
            n37 = Scan From String(input string=w129, error in=w128, default 1=enum16{"Basic256", "Basic128Rsa15"}."Basic256" ("Server.security policy.security")) -> (error out=w122:errorcluster, output 1=w126:enum16{"Basic256", "Basic128Rsa15"})  [unwired: 2 in, 2 out]
            n38 = Scan From String(input string=w130, error in=w127, default 1=enum16{"None", "Sign", "Sign and Encrypt"}."None" ("Server.security policy.message mode")) -> (error out=w121:errorcluster, output 1=w125:enum16{"None", "Sign", "Sign and Encrypt"})  [unwired: 2 in, 2 out]
            n39 = Bundle By Name(cluster=w156, "Server.security policy.security"=w126, "Server.security policy.message mode"=w125, "Server.OPC port"=w144, "Server.name"=w151) -> (w154:T21)
            n40 = Merge Errors(w124, w122, w121) -> (w123:errorcluster)
          }
          frame condition #1 {
          }
        }
      }
      frame "Read Enums" {
        w166 = System."GM3HT1"  # System_enum
        w167 = ALR."GM1JBA1JA1_CONN"  # ALR_enum
        w168 = DO."GM1FZ1_YB47"  # DO_enum
        w169 = AO."GM1QN1_YQ01"  # AO_enum
        w170 = DI_FAST."W1.KF_XB01"  # DI_enum fast
        w171 = DI."GM1FZ1_XB19"  # DI_enum
        w172 = AI."GM1QN1_XQ01"  # AI_enum
        w173 = PAR."GM1QN1_output_set_time"  # PAR_enum
        w174 = KFM."GM1JBA1_JA1"  # KFM_enum
        w195 = T14 {"KFM"=[], "PAR"=[], "AI"=[], "DI"=[], "DI_fast"=[], "AO"=[], "DO"=[], "ALR"=[], "System"=[]}  # Enums
        n41 = call <userlib>:"Get Strings from Enum__ogtk.vi"("error in (no error)"=w186, "Enum"=w174) -> ("error out"=w185:errorcluster, "Enum Strings"=w194:string[])  [unwired: 6 in, 2 out]
        n42 = call <userlib>:"Get Strings from Enum__ogtk.vi"("error in (no error)"=w186, "Enum"=w173) -> ("error out"=w184:errorcluster, "Enum Strings"=w193:string[])  [unwired: 6 in, 2 out]
        n43 = call <userlib>:"Get Strings from Enum__ogtk.vi"("error in (no error)"=w186, "Enum"=w172) -> ("error out"=w183:errorcluster, "Enum Strings"=w192:string[])  [unwired: 6 in, 2 out]
        n44 = call <userlib>:"Get Strings from Enum__ogtk.vi"("error in (no error)"=w186, "Enum"=w171) -> ("error out"=w182:errorcluster, "Enum Strings"=w191:string[])  [unwired: 6 in, 2 out]
        n45 = call <userlib>:"Get Strings from Enum__ogtk.vi"("error in (no error)"=w186, "Enum"=w170) -> ("error out"=w181:errorcluster, "Enum Strings"=w190:string[])  [unwired: 6 in, 2 out]
        n46 = call <userlib>:"Get Strings from Enum__ogtk.vi"("error in (no error)"=w186, "Enum"=w169) -> ("error out"=w180:errorcluster, "Enum Strings"=w189:string[])  [unwired: 6 in, 2 out]
        n47 = call <userlib>:"Get Strings from Enum__ogtk.vi"("error in (no error)"=w186, "Enum"=w168) -> ("error out"=w179:errorcluster, "Enum Strings"=w188:string[])  [unwired: 6 in, 2 out]
        n48 = call <userlib>:"Get Strings from Enum__ogtk.vi"("error in (no error)"=w186, "Enum"=w167) -> ("error out"=w178:errorcluster, "Enum Strings"=w187:string[])  [unwired: 6 in, 2 out]
        n49 = call <userlib>:"Get Strings from Enum__ogtk.vi"("error in (no error)"=w186, "Enum"=w166) -> ("error out"=w177:errorcluster)  [unwired: 6 in, 3 out]
        n50 = Bundle By Name(cluster=w195, "KFM"=w194, "PAR"=w193, "AI"=w192, "DI"=w191, "DI_fast"=w190, "AO"=w189, "DO"=w188, "ALR"=w187, "System"=string[] []) -> (w197:T14)
        n51 = Merge Errors(w185, w184, w183, w182, w181, w180, w179, w178, w177) -> (w176:errorcluster)
        n52 = Bundle By Name(cluster=w198, "Enums"=w197) -> (w196:T21)
      }
      frame "Read OPC param" {
        n53 = disable-structure shown="SERVER==OPC" {
          disable-tunnel: w205 -> [w228 w234]
          disable-tunnel: [w227 w235] -> w203
          disable-tunnel: [w209 w234] -> w202
          disable-tunnel: w201 -> [w221 w235]
          disable-tunnel: w201 -> [w213 _]
          frame condition #0 (active) {
            w229 = TRUE  # trust any server
            # "1."
            n54 = Unbundle By Name(w213) -> ("Server.name"=w223:string, "Server.OPC port"=w219:string, "Server.security policy"=w208:T32)
            n55 = Concatenate Strings("opc.tcp://" ("server endpoint URL 2"), w223, ":" ("server endpoint URL 2"), w219) -> (w218:string)
            n56 = call <vilib>:"Connect.vi"("trust any server (F)"=w229, "error in (no error)"=w228, "security policy"=w208, "server endpoint URL"=w218) -> ("error out"=w231:errorcluster, "OPC UA client refnum out"=w232:T17)  [unwired: 5 in, 1 out]
            n57 = call <vilib>:"Create Subscription.vi"("error in (no error)"=w231, "publishing interval (1000 ms)"=100.0 ("update rate (1000 ms)"), "OPC UA client refnum in"=w232) -> ("error out"=w210:errorcluster, "OPC UA data change event"=w212:refnum<user-event>, "subscription ID out"=w225:T18, "OPC UA client refnum out"=w233:T17)  [unwired: 4 in, 1 out]
            n58 = register-events(w212) -> (reference out=w211:refnum<event-registration>)  [unwired: 2 in, 1 out]
            n59 = call "OPC_server_param.vi"() -> ("Parameters"=w217:T33[])  [unwired: 11 in]
            n60 = call "Select OPC node IDs.vi"("OPC Params"=w217) -> ("parameters"=w214:T37, "requests"=w215:T19[], "node IDs"=w216:string[])  [unwired: 8 in]
            n61 = call <vilib>:"Add Monitored Data Nodes.vi"("monitoring parameters"=w214, "error in (no error)"=w210, "node IDs"=w216, "subscription ID in"=w225, "OPC UA client refnum in"=w233) -> ("error out"=w209:errorcluster, "OPC UA client refnum out"=w224:T17)  [unwired: 3 in, 2 out]
            n62 = Build Array(w225) -> (w226:T18[])
            n63 = Bundle By Name(cluster=w221, "OPC UA.data change event"=w212, "OPC UA.Event Reg"=w211, "OPC UA.node IDs"=w216, "OPC UA.subscription IDs"=w226, "OPC UA.requests"=w215, "OPC UA.Client refnum"=w224) -> (w227:T21)
          }
          frame condition #1 {
          }
        }
      }
      frame "Read AI param" {
        n64 = disable-structure shown="SERVER==OPC" {
          disable-tunnel: w241 -> [w258 w267]
          disable-tunnel: [w256 w272] -> w240
          disable-tunnel: w238 -> [w251 w272]
          disable-tunnel: [w246 w268] -> w239
          disable-tunnel: w238 -> [w249 w271]
          disable-tunnel: w236 -> [w244 w265]
          disable-tunnel: [w244 w263] -> w237
          frame condition #0 {
            w245 = T38 {"Read Access"=enum."Allowed", "Write Access"=enum."None"} ("access")
            w248 = "ni.var.psp://" ("server endpoint URL 2")
            n65 = Unbundle By Name(w249) -> ("Server.name"=w247:string)
            n66 = Concatenate Strings(w248, w247, "/InputsVar/AI" ("server endpoint URL 2")) -> (w259:string)
            n67 = shared-variable-open ("AI_ref")(w259, w258, T4 {"AI"=[], "AIState"=[], "AIALRState"=[]} ("AI"), w245) -> (w257:refnum<k21>, w255:errorcluster)
            n68 = Concatenate Strings(w248, w247, "/InputsVar/AI_fcode_full" ("server endpoint URL 2")) -> (w254:string)
            n69 = shared-variable-open ("AI_ref")(w254, w255, string[] [] ("AI"), w245) -> (w250:refnum<k21>, w246:errorcluster)
            n70 = Bundle By Name(cluster=w251, "AI_SHVR"=w257, "AI_Names_SHVR"=w250) -> (w256:T21)
          }
          frame condition #1 (active) {
            n71 = Unbundle By Name(w271) -> ("system DB"=w266:T15)
            n72 = Unbundle By Name(w271) -> ("Enums.AO"=w270:string[])
            n73 = call "Get bronkhorst param from PGserver.vi"("conninfo"=w266, "error in (no error)"=w267, "AIParamTable"="bronkhorst_1", "AIParameters"=w270) -> ("error out"=w268:errorcluster, "Names table"=w262:string[][], "Parameters table"=w264:dbl[][])  [unwired: 5 in]
            n74 = Bundle By Name(cluster=w265, "RegsParam"=w264, "Regs_Descriptions"=w262) -> (w263:T22)
          }
        }
      }
      frame "AI references" {
        w274 = AI."GM1QN1_XQ01"  # AI_enum
        n75 = Unbundle By Name(w275) -> ("Enums.AI"=w277:string[])
        n76 = Array Size(array=w277) -> (size(s)=w278:i32)
        n77 = for {
          N: w278 -> [_]
          tunnel: w274 -> [w286]
          tunnel: [w283] -> w273 mode=indexing
          i -> [w284]
          n78 = Coerce To Type(0:w284, 1:w286) -> (2:w285:T1)
          n79 = case shown="\"GM1QN1_XQ01\"" w285 {
            tunnel: [_ w287] -> w283
            frame Default {
            }
            frame "GM1QN1_XQ01" {
              n80 = control-ref of="PV 2"() -> (w287:refnum<vi>)
            }
          }
        }
        n81 = Bundle By Name(cluster=w275, "AI_refs"=w273) -> (w276:T21)
      }
      frame "AI reorder" {
        n82 = disable-structure shown="SERVER==OPC" {
          disable-tunnel: [w300 w311] -> w293
          disable-tunnel: w290 -> [w302 w317]
          disable-tunnel: w292 -> [w297 w310]
          disable-tunnel: [w296 w309] -> w291
          frame condition #0 {
            n83 = Unbundle By Name(w302) -> ("Enums.AI"=w299:string[], "AI_Names_SHVR"=w301:refnum<k21>)
            n84 = shared-variable-read(w301, w297) -> (w296:errorcluster, w298:string[])  [unwired: 2 out]
            n85 = case shown="No Error" w296 {
              tunnel: w298 -> [_ w303]
              tunnel: w299 -> [_ w305]
              tunnel: [_ w304] -> w300
              frame Error {
              }
              frame No Error {
                n86 = for {
                  tunnel: w305 -> [w308] mode=indexing
                  tunnel: w303 -> [w307]
                  tunnel: [w306] -> w304 mode=indexing
                  n87 = Search 1D Array(1D array=w307, element=w308) -> (index of element=w306:i32)  [unwired: 1 in]
                }
              }
            }
          }
          frame condition #1 (active) {
            n88 = Unbundle By Name(w317) -> ("Enums.AI"=w312:string[], "OPC UA.Client refnum"=w314:T17)
            n89 = call-poly <vilib>:"Multiple Read.vi"("error in (no error)"=w310, "node IDs"=T6 ["ns=2;s=AI.AI_Names"] ("OPC UA.node IDs"), "OPC UA client refnum in"=w314) -> ("error out"=w309:errorcluster, "results"=w316:T40, "service status"=w315:T39)  [unwired: 5 in, 1 out]
            n90 = case shown="0..15" w315 {
              tunnel: w316 -> [_ w321]
              tunnel: w312 -> [_ w319]
              tunnel: [_ w318] -> w311
              frame 16.., Default {
              }
              frame 0..15 {
                n91 = Index Array(array=w321) -> (element=w322:T41)  [unwired: 1 in]
                n92 = Unbundle By Name(w322) -> ("values"=w320:string[])
                n93 = for {
                  tunnel: w319 -> [w325] mode=indexing
                  tunnel: w320 -> [w324]
                  tunnel: [w323] -> w318 mode=indexing
                  n94 = Search 1D Array(1D array=w324, element=w325) -> (index of element=w323:i32)  [unwired: 1 in]
                }
              }
            }
          }
        }
        n95 = Bundle By Name(cluster=w288, "AI_reorder_table"=w293) -> (w289:T22)
      }
      frame "AI Descriptions" {
        n96 = Unbundle By Name(w329) -> ("OPC UA.Client refnum"=w339:T17)
        n97 = Unbundle By Name(w329) -> ("AI_refs"=w328:refnum<vi>[])
        n98 = Unbundle By Name(w333) -> ("AI_reorder_table"=w332:i32[])
        n99 = call-poly <vilib>:"Multiple Read.vi"("error in (no error)"=w337, "node IDs"=T6 ["ns=2;s=AI.AI_Descriptions"] ("OPC UA.node IDs"), "OPC UA client refnum in"=w339) -> ("error out"=w336:errorcluster, "results"=w335:T42)  [unwired: 5 in, 2 out]
        n100 = Index Array(array=w335) -> (element=w334:T43)  [unwired: 1 in]
        n101 = Unbundle By Name(w334) -> ("values"=w338:u8[][])
        n102 = for {
          tunnel: w338 -> [w354] mode=indexing
          tunnel: [w352] -> w326 mode=indexing
          tunnel: u8[] [0] ("unsigned byte array") -> [w350]
          n103 = Byte Array To String(unsigned byte array=w354) -> (string=w353:string)
          n104 = Byte Array To String(unsigned byte array=w350) -> (string=w351:string)
          n105 = Match Pattern(string=w353, regular expression=w351) -> (before substring=w352:string)  [unwired: 1 in, 3 out]
        }
        n106 = for {
          tunnel: w332 -> [w347] mode=indexing
          tunnel: w326 -> [w346]
          tunnel: [w345] -> w331 mode=indexing
          tunnel: w328 -> [w343] mode=indexing
          n107 = Not A Number/Path/Refnum?(number/path/refnum=w343) -> (NaN/Path/Refnum?=w344:bool)
          n108 = Index Array(array=w346, index=w347) -> (element=w345:string)
          n109 = case shown="False" w344 {
            tunnel: w345 -> [w349 _]
            tunnel: w343 -> [w348 _]
            frame False {
              n110 = property on="Property Node" class="Slide (strict)"(reference=w348, "TipStrip"=w349) -> ()  [unwired: 1 in, 2 out]
            }
            frame True {
            }
          }
        }
        n111 = Bundle By Name(cluster=w329, "AI_Descriptions"=w331) -> (w330:T21)
      }
      frame "Read DI param" {
        n112 = disable-structure shown="SERVER==SHRV, Default" {
          disable-tunnel: w359 -> [w363 w378]
          disable-tunnel: [w362 w376] -> w358
          disable-tunnel: w355 -> [w362 w369]
          disable-tunnel: [w363 w367] -> w356
          disable-tunnel: w355 -> [_ w365]
          frame condition #0 (active) {
          }
          frame condition #1 {
            w364 = T38 {"Read Access"=enum."Allowed", "Write Access"=enum."None"} ("access")
            w373 = "ni.var.psp://" ("server endpoint URL 2")
            n113 = Unbundle By Name(w365) -> ("Server.name"=w372:string)
            n114 = Concatenate Strings(w373, w372, "/InputsVar/DI" ("server endpoint URL 2")) -> (w379:string)
            n115 = shared-variable-open ("AI_ref")(w379, w378, T8 {"DI"=[], "DI_State"=[], "DI_ALRState"=[]} ("DI"), w364) -> (w377:refnum<k21>, w375:errorcluster)
            n116 = Concatenate Strings(w373, w372, "/InputsVar/DI_fcode_full" ("server endpoint URL 2")) -> (w374:string)
            n117 = shared-variable-open ("AI_ref")(w374, w375, string[] [] ("AI"), w364) -> (w368:refnum<k21>, w367:errorcluster)
            n118 = Bundle By Name(cluster=w369, "DI_SHVR"=w377, "DI_Names_SHVR"=w368) -> (w376:T21)
          }
        }
      }
      frame "Read ALR param" {
        n119 = Unbundle By Name(w384) -> ("ALR_State"=w390:T9)
        n120 = Unbundle By Name(w386) -> ("Enums.ALR"=w391:string[])
        n121 = Array Size(array=w391) -> (size(s)=w382:i32)
        n122 = call "ALR scada init.vi"("error in (no error)"=w387, "N_param"=w382, "ALR_State in"=w390) -> ("error out"=w388:errorcluster, "ALR_State out"=w389:T9)  [unwired: 7 in]
        n123 = disable-structure shown="SERVER==SHRV, Default" {
          disable-tunnel: w388 -> [w416 w420]
          disable-tunnel: [w415 w428] -> w393
          disable-tunnel: w386 -> [w414 w427]
          disable-tunnel: [w413 w417] -> w392
          disable-tunnel: w386 -> [_ w419]
          frame condition #0 {
            w401 = T38 {"Read Access"=enum."Allowed", "Write Access"=enum."None"} ("access")
            w400 = "ni.var.psp://" ("server endpoint URL 2")
            n124 = Unbundle By Name(w414) -> ("Server.name"=w399:string)
            n125 = Concatenate Strings(w400, w399, "/ALRVar/ALR_State" ("server endpoint URL 2")) -> (w411:string)
            n126 = shared-variable-open ("AI_ref")(w411, w416, T9 {"ALR not block"=[], "ALR"=[], "ALR blocked"=[], "ALR ON"=[], "code"=[], "level"=[], "t ms"=[], "ack state"=[], "color"=[]} ("ALR_State"), w401) -> (w410:refnum<k21>, w409:errorcluster)
            n127 = Concatenate Strings(w400, w399, "/ALRVar/ALR_Descriptions" ("server endpoint URL 2")) -> (w408:string)
            n128 = shared-variable-open ("AI_ref")(w408, w409, string[] [] ("ALR_Names"), w401) -> (w396:refnum<k21>, w402:errorcluster)
            n129 = Concatenate Strings(w400, w399, "/Var/Total" ("server endpoint URL 2")) -> (w404:string)
            n130 = shared-variable-open ("AI_ref")(w404, w402, 0.0 ("CPU_utilization"), w401) -> (w397:refnum<k21>, w413:errorcluster)
            n131 = Bundle By Name(cluster=w414, "ALR_state_SHRV"=w410, "ALR_Descriptions_SHRV"=w396, "CPU_utilization"=w397) -> (w415:T21)
          }
          frame condition #1 (active) {
            n132 = Unbundle By Name(w419) -> ("OPC UA.Client refnum"=w423:T17)
            n133 = call-poly <vilib>:"Multiple Read.vi"("error in (no error)"=w420, "node IDs"=T6 ["ns=2;s=ALR.ALR_Descriptions"] ("OPC UA.node IDs"), "OPC UA client refnum in"=w423) -> ("error out"=w417:errorcluster, "results"=w425:T42)  [unwired: 5 in, 2 out]
            n134 = Index Array(array=w425) -> (element=w426:T43)  [unwired: 1 in]
            n135 = Unbundle By Name(w426) -> ("values"=w424:u8[][])
            n136 = for {
              tunnel: w424 -> [w433] mode=indexing
              tunnel: [w431] -> w418 mode=indexing
              tunnel: u8[] [0] ("unsigned byte array") -> [w429]
              n137 = Byte Array To String(unsigned byte array=w433) -> (string=w432:string)
              n138 = Byte Array To String(unsigned byte array=w429) -> (string=w430:string)
              n139 = Match Pattern(string=w432, regular expression=w430) -> (before substring=w431:string)  [unwired: 1 in, 3 out]
            }
            n140 = Bundle By Name(cluster=w427, "ALR_Descriptions"=w418) -> (w428:T21)
          }
        }
        n141 = Initialize Array("", w382) -> (w381:string[])
        n142 = Bundle By Name(cluster=w384, "ALR_State"=w389, "ALR_Names"=w381) -> (w385:T22)
      }
      frame "Read control param" {
        n143 = disable-structure shown="SERVER==SHRV, Default" {
          disable-tunnel: w438 -> [w442 w459]
          disable-tunnel: [w441 w458] -> w437
          disable-tunnel: w434 -> [w441 w455]
          disable-tunnel: [w442 _] -> w435
          disable-tunnel: w434 -> [_ w454]
          frame condition #0 (active) {
          }
          frame condition #1 {
            w443 = T44 {"Z_HSw"=0, "Z_HSetState"=enum."stop ready", "Y_HSw"=0, "Y_HSetState"=enum."hand", "SP"=0.0, "Y_H"=0.0, "Reset_ALR"=FALSE} ("ZY_control")
            w451 = T38 {"Read Access"=enum."Allowed", "Write Access"=enum."Allowed"} ("access")
            w450 = "ni.var.psp://" ("server endpoint URL 2")
            n144 = Unbundle By Name(w454) -> ("Server.name"=w449:string)
            n145 = Concatenate Strings(w450, w449, "/Var/EB2TB1_control" ("server endpoint URL 2")) -> (w460:string)
            n146 = shared-variable-open ("AI_ref")(w460, w459, w443, w451) -> (w446:refnum<k21>, w457:errorcluster)
            n147 = Concatenate Strings(w450, w449, "/Var/EB2TB2_control" ("server endpoint URL 2")) -> (w456:string)
            n148 = shared-variable-open ("AI_ref")(w456, w457, w443, w451) -> (w445:refnum<k21>, w452:errorcluster)
            n149 = Concatenate Strings(w450, w449, "/Var/EB2TB3_control" ("server endpoint URL 2")) -> (w453:string)
            n150 = shared-variable-open ("AI_ref")(w453, w452, w443, w451) -> (w444:refnum<k21>)  [unwired: 1 out]
            n151 = Bundle By Name(cluster=w455, "CPU_utilization"=w446, "AI_Descriptions"=w445, "ALR_Descriptions"=w444) -> (w458:T21)
          }
        }
      }
      frame "Read state param" {
        n152 = disable-structure shown="SERVER==SHRV, Default" {
          disable-tunnel: w466 -> [w470 w487]
          disable-tunnel: [w469 w486] -> w465
          disable-tunnel: w462 -> [w469 w483]
          disable-tunnel: [w470 _] -> w463
          disable-tunnel: w462 -> [_ w482]
          frame condition #0 (active) {
          }
          frame condition #1 {
            w471 = T47 {"Z"={"Z_Source"=enum."hand", "Z_SetState"=enum."stop ready", "Z_State"=enum."initialization", "Z_State_T"=0, "ZM_State"=enum."initialization", "ZM_State_T"=0, "ALR  L1"=FALSE, "ALR  L2"=FALSE, "HH_run"=0}, "Y"={"Y_Source"=enum."hand", "Y_SetState"=enum."hand", "SP_Set"=0.0, "SP"=0.0, "PV"=0.0, "Y_Set"=0.0, "Y"=0.0, "Y_State"={"code"=0, "visible"=FALSE, "color"=0}, "YB"=FALSE}, "ALR_Status"=[]} ("AI")
            w479 = T38 {"Read Access"=enum."Allowed", "Write Access"=enum."Allowed"} ("access")
            w478 = "ni.var.psp://" ("server endpoint URL 2")
            n153 = Unbundle By Name(w482) -> ("Server.name"=w477:string)
            n154 = Concatenate Strings(w478, w477, "/Var/EB2TB1_state" ("server endpoint URL 2")) -> (w488:string)
            n155 = shared-variable-open ("AI_ref")(w488, w487, w471, w479) -> (w474:refnum<k21>, w485:errorcluster)
            n156 = Concatenate Strings(w478, w477, "/Var/EB2TB2_state" ("server endpoint URL 2")) -> (w484:string)
            n157 = shared-variable-open ("AI_ref")(w484, w485, w471, w479) -> (w473:refnum<k21>, w480:errorcluster)
            n158 = Concatenate Strings(w478, w477, "/Var/EB2TB3_state" ("server endpoint URL 2")) -> (w481:string)
            n159 = shared-variable-open ("AI_ref")(w481, w480, w471, w479) -> (w472:refnum<k21>)  [unwired: 1 out]
            n160 = Bundle By Name(cluster=w483, "AI_refs"=w474, "DI_Descriptions"=w473, "EB2TB3_state"=w472) -> (w486:T21)
          }
        }
      }
      frame "Init Shared Variables" {
        n161 = Initialize Array(T12 {"connect"=FALSE, "gas"="H2", "Y_State"={"Y_Source"=3, "Y_SetState"=0, "SP_Set"=0.0, "SP"=0.0, "PV"=0.0, "PV_State"={"code"=0, "visible"=FALSE, "color"=0}, "Y_preSet"=0.0, "Y_Set"=0.0, "Y"=0.0, "Y_State"={"code"=0, "visible"=FALSE, "color"=0}, "YB"=FALSE}} ("Y_short_conn"), 24 ("dimension size")) -> (w490:T54)
        n162 = shared-variable ".\\Var scada.lvlib\\QN_states_short"(w490, error in=w492) -> (error out=w493:errorcluster)
      }
      frame "Init ALR Listbox symbols" {
        w508 = T55 {"image type"=0, "image depth"=24, "image"=[153, 204, 51, 153, 204, 51, 153, 204, 51, 153, 204, 51, 153, 204, 51, 153, 204, 51, 153, 204, 51, 153, 204, 51, 153, 204, 51, 153, 204, 51, 153, 204, 51, 153, 204, 51, 153, 204, 51, 153, 204, 51, 153, 204, 51, 153, 204, 51, 153, 204, 51, 153, 204, 51, 153, 204, 51, 153, 204, 51, 153, 204, 51, 153, 204, 51, 153, 204, 51, 153, 204, 51, 153, 204, 51, 153, 204, 51, 153, 204, 51, 153, 204, 51, 153, 204, 51, 153, 204, 51, 153, 204, 51, 153, 204, 51, 153, 204, 51, 153, 204, 51, 153, 204, 51, 153, 204, 51, 255, 255, 255, 255, 255, 255, 153, 204, 51, 153, 204, 51, 153, 204, 51, 153, 204, 51, 153, 204, 51, 153, 204, 51, 153, 204, 51, 153, 204, 51, 153, 204, 51, 153, 204, 51, 153, 204, 51, 153, 204, 51, 153, 204, 51, 153, 204, 51, 153, 204, 51, 255, 255, 255, 255, 255, 255, 255, 255, 255, 153, 204, 51, 153, 204, 51, 153, 204, 51, 153, 204, 51, 153, 204, 51, 153, 204, 51, 153, 204, 51, 153, 204, 51, 153, 204, 51, 153, 204, 51, 153, 204, 51, 153, 204, 51, 153, 204, 51, 153, 204, 51, 153, 204, 51, 255, 255, 255, 255, 255, 255, 255, 255, 255, 153, 204, 51, 153, 204, 51, 153, 204, 51, 153, 204, 51, 153, 204, 51, 153, 204, 51, 153, 204, 51, 153, 204, 51, 153, 204, 51, 153, 204, 51, 153, 204, 51, 153, 204, 51, 153, 204, 51, 153, 204, 51, 153, 204, 51, 255, 255, 255, 255, 255, 255, 255, 255, 255, 153, 204, 51, 153, 204, 51, 153, 204, 51, 153, 204, 51, 153, 204, 51, 153, 204, 51, 153, 204, 51, 153, 204, 51, 153, 204, 51, 153, 204, 51, 153, 204, 51, 153, 204, 51, 153, 204, 51, 153, 204, 51, 153, 204, 51, 255, 255, 255, 255, 255, 255, 255, 255, 255, 153, 204, 51, 153, 204, 51, 153, 204, 51, 255, 255, 255, 153, 204, 51, 153, 204, 51, 153, 204, 51, 153, 204, 51, 153, 204, 51, 153, 204, 51, 153, 204, 51, 153, 204, 51, 153, 204, 51, 153, 204, 51, 153, 204, 51, 255, 255, 255, 255, 255, 255, 255, 255, 255, 153, 204, 51, 255, 255, 255, 255, 255, 255, 153, 204, 51, 153, 204, 51, 153, 204, 51, 153, 204, 51, 153, 204, 51, 153, 204, 51, 153, 204, 51, 153, 204, 51, 153, 204, 51, 153, 204, 51, 153, 204, 51, 153, 204, 51, 255, 255, 255, 255, 255, 255, 255, 255, 255, 255, 255, 255, 255, 255, 255, 255, 255, 255, 153, 204, 51, 153, 204, 51, 153, 204, 51, 153, 204, 51, 153, 204, 51, 153, 204, 51, 153, 204, 51, 153, 204, 51, 153, 204, 51, 153, 204, 51, 153, 204, 51, 153, 204, 51, 255, 255, 255, 255, 255, 255, 255, 255, 255, 255, 255, 255, 255, 255, 255, 153, 204, 51, 153, 204, 51, 153, 204, 51, 153, 204, 51, 153, 204, 51, 153, 204, 51, 153, 204, 51, 153, 204, 51, 153, 204, 51, 153, 204, 51, 153, 204, 51, 255, 255, 255, 255, 255, 255, 255, 255, 255, 255, 255, 255, 255, 255, 255, 255, 255, 255, 153, 204, 51, 153, 204, 51, 153, 204, 51, 153, 204, 51, 153, 204, 51, 153, 204, 51, 153, 204, 51, 153, 204, 51, 153, 204, 51, 153, 204, 51, 255, 255, 255, 255, 255, 255, 255, 255, 255, 255, 255, 255, 255, 255, 255, 255, 255, 255, 255, 255, 255, 255, 255, 255, 153, 204, 51, 153, 204, 51, 153, 204, 51, 153, 204, 51, 153, 204, 51, 153, 204, 51, 153, 204, 51, 153, 204, 51, 153, 204, 51, 153, 204, 51, 153, 204, 51, 255, 255, 255, 255, 255, 255, 255, 255, 255, 255, 255, 255, 255, 255, 255, 255, 255, 255, 153, 204, 51, 153, 204, 51, 153, 204, 51, 153, 204, 51, 153, 204, 51, 153, 204, 51, 153, 204, 51, 153, 204, 51, 153, 204, 51, 153, 204, 51, 153, 204, 51, 153, 204, 51, 153, 204, 51, 153, 204, 51, 255, 255, 255, 255, 255, 255, 255, 255, 255, 153, 204, 51, 153, 204, 51, 153, 204, 51, 153, 204, 51, 153, 204, 51, 153, 204, 51, 153, 204, 51, 153, 204, 51, 153, 204, 51, 153, 204, 51, 153, 204, 51, 153, 204, 51, 153, 204, 51, 153, 204, 51, 153, 204, 51, 153, 204, 51, 153, 204, 51, 153, 204, 51, 153, 204, 51, 153, 204, 51, 153, 204, 51, 153, 204, 51, 153, 204, 51, 153, 204, 51, 153, 204, 51, 153, 204, 51, 153, 204, 51, 153, 204, 51, 153, 204, 51, 153, 204, 51, 153, 204, 51, 153, 204, 51, 153, 204, 51, 153, 204, 51, 153, 204, 51, 153, 204, 51, 153, 204, 51, 153, 204, 51, 153, 204, 51, 153, 204, 51, 153, 204, 51, 153, 204, 51, 153, 204, 51, 153, 204, 51, 153, 204, 51, 153, 204, 51, 153, 204, 51, 153, 204, 51, 153, 204, 51, 153, 204, 51, 153, 204, 51, 153, 204, 51, 153, 204, 51, 153, 204, 51], "mask"=[], "colors"=[], "Rectangle"={"left"=0, "top"=0, "right"=17, "bottom"=17}}  # green down arrow
        w500 = T55 {"image type"=0, "image depth"=24, "image"=array[867 elements], "mask"=[], "colors"=[], "Rectangle"={"left"=0, "top"=0, "right"=17, "bottom"=17}}  # gray
        w510 = T55 {"image type"=0, "image depth"=24, "image"=[77, 77, 77, 77, 77, 77, 77, 77, 77, 77, 77, 77, 77, 77, 77, 77, 77, 77, 77, 77, 77, 77, 77, 77, 77, 77, 77, 77, 77, 77, 77, 77, 77, 77, 77, 77, 77, 77, 77, 77, 77, 77, 77, 77, 77, 77, 77, 77, 77, 77, 77, 77, 77, 77, 77, 77, 77, 77, 77, 77, 77, 77, 77, 77, 77, 77, 77, 77, 77, 77, 77, 77, 77, 77, 77, 77, 77, 77, 77, 77, 77, 77, 77, 77, 77, 77, 77, 77, 77, 77, 77, 77, 77, 77, 77, 77, 77, 77, 77, 77, 77, 77, 77, 77, 77, 77, 77, 77, 77, 77, 77, 77, 77, 77, 77, 77, 77, 77, 77, 77, 77, 77, 77, 77, 77, 77, 77, 77, 77, 77, 77, 77, 77, 77, 77, 77, 77, 77, 77, 77, 77, 77, 77, 77, 77, 77, 77, 77, 77, 77, 77, 77, 77, 77, 77, 77, 77, 77, 77, 77, 77, 77, 77, 77, 77, 77, 77, 77, 77, 77, 77, 77, 77, 77, 77, 77, 77, 77, 77, 77, 77, 77, 77, 77, 77, 77, 77, 77, 77, 77, 77, 77, 77, 77, 77, 77, 77, 77, 77, 77, 77, 77, 77, 77, 77, 77, 77, 77, 77, 77, 77, 77, 77, 77, 77, 77, 77, 77, 77, 77, 77, 77, 77, 77, 77, 77, 77, 77, 77, 77, 77, 77, 77, 77, 77, 77, 77, 77, 77, 77, 77, 77, 77, 77, 77, 77, 77, 77, 77, 77, 77, 77, 77, 77, 77, 77, 77, 77, 77, 77, 77, 77, 77, 77, 77, 77, 77, 77, 77, 77, 77, 77, 77, 77, 77, 77, 77, 77, 77, 77, 77, 77, 77, 77, 77, 77, 77, 77, 77, 77, 77, 77, 77, 77, 77, 77, 77, 77, 77, 77, 77, 77, 77, 77, 77, 77, 77, 77, 77, 77, 77, 77, 77, 77, 77, 77, 77, 77, 77, 77, 77, 77, 77, 77, 77, 77, 77, 77, 77, 77, 77, 77, 77, 77, 77, 77, 77, 77, 77, 77, 77, 77, 77, 77, 77, 77, 77, 77, 77, 77, 77, 77, 77, 77, 77, 77, 77, 77, 77, 77, 77, 77, 77, 77, 77, 77, 77, 77, 77, 77, 77, 77, 77, 77, 77, 77, 77, 77, 77, 77, 77, 77, 77, 77, 77, 77, 77, 77, 77, 77, 77, 77, 77, 77, 77, 77, 77, 77, 77, 77, 77, 77, 77, 77, 77, 77, 77, 77, 77, 77, 77, 77, 77, 77, 77, 77, 77, 77, 77, 77, 77, 77, 77, 77, 77, 77, 77, 77, 77, 77, 77, 77, 77, 77, 77, 77, 77, 77, 77, 77, 77, 77, 77, 77, 77, 77, 77, 77, 77, 77, 77, 77, 77, 77, 77, 77, 77, 77, 77, 77, 77, 77, 77, 77, 77, 77, 77, 77, 77, 77, 77, 77, 77, 77, 77, 77, 77, 77, 77, 77, 77, 77, 77, 77, 77, 77, 77, 77, 77, 77, 77, 77, 77, 77, 77, 77, 77, 77, 77, 77, 77, 77, 77, 77, 77, 77, 77, 77, 77, 77, 77, 77, 77, 77, 77, 77, 77, 77, 77, 77, 77, 77, 77, 77, 77, 77, 77, 77, 77, 77, 77, 77, 77, 77, 77, 77, 77, 77, 77, 77, 77, 77, 77, 77, 77, 77, 77, 77, 77, 77, 77, 77, 77, 77, 77, 77, 77, 77, 77, 77, 77, 77, 77, 77, 77, 77, 77, 77, 77, 77, 77, 77, 77, 77, 77, 77, 77, 77, 77, 77, 77, 77, 77, 77, 77, 77, 77, 77, 77, 77, 77, 77, 77, 77, 77, 77, 77, 77, 77, 77, 77, 77, 77, 77, 77, 77, 77, 77, 77, 77, 77, 77, 77, 77, 77, 77, 77, 77, 77, 77, 77, 77, 77, 77, 77, 77, 77, 77, 77, 77, 77, 77, 77, 77, 77, 77, 77, 77, 77, 77, 77, 77, 77, 77, 77, 77, 77, 77, 77, 77, 77, 77, 77, 77, 77, 77, 77, 77, 77, 77, 77, 77, 77, 77, 77, 77, 77, 77, 77, 77, 77, 77, 77, 77, 77, 77, 77, 77, 77, 77, 77, 77, 77, 77, 77, 77, 77, 77, 77, 77, 77, 77, 77, 77, 77, 77, 77, 77, 77, 77, 77, 77, 77, 77, 77, 77, 77, 77, 77, 77, 77, 77, 77, 77, 77, 77, 77, 77, 77, 77, 77, 77, 77, 77, 77, 77, 77, 77, 77, 77, 77, 77, 77, 77, 77, 77, 77, 77, 77, 77, 77, 77, 77, 77, 77, 77, 77, 77, 77, 77, 77, 77, 77, 77, 77, 77, 77, 77, 77, 77, 77, 77, 77, 77, 77, 77, 77, 77, 77, 77, 77, 77, 77, 77, 77, 77, 77, 77, 77, 77, 77, 77, 77, 77, 77, 77, 77, 77, 77, 77, 77, 77, 77, 77, 77, 77, 77, 77, 77, 77, 77, 77, 77, 77, 77, 77, 77, 77, 77, 77, 77, 77, 77, 77, 77, 77, 77, 77, 77, 77, 77, 77, 77, 77, 77, 77, 77, 77, 77, 77, 77, 77, 77, 77, 77, 77, 77, 77, 77, 77, 77, 77, 77, 77, 77, 77, 77, 77, 77, 77, 77, 77, 77, 77, 77, 77, 77, 77, 77, 77, 77, 77, 77, 77, 77, 77, 77], "mask"=[], "colors"=[], "Rectangle"={"left"=0, "top"=0, "right"=17, "bottom"=17}}  # brown
        w509 = T55 {"image type"=0, "image depth"=24, "image"=[77, 77, 77, 77, 77, 77, 77, 77, 77, 77, 77, 77, 77, 77, 77, 77, 77, 77, 77, 77, 77, 77, 77, 77, 77, 77, 77, 77, 77, 77, 77, 77, 77, 77, 77, 77, 77, 77, 77, 77, 77, 77, 77, 77, 77, 77, 77, 77, 77, 77, 77, 77, 77, 77, 77, 77, 77, 77, 77, 77, 77, 77, 77, 77, 77, 77, 77, 77, 77, 77, 77, 77, 77, 77, 77, 77, 77, 77, 77, 77, 77, 77, 77, 77, 77, 77, 77, 77, 77, 77, 77, 77, 77, 77, 77, 77, 77, 77, 77, 77, 77, 77, 77, 77, 77, 77, 77, 77, 77, 77, 77, 77, 77, 77, 77, 77, 77, 77, 77, 77, 77, 77, 77, 77, 77, 77, 77, 77, 77, 77, 77, 77, 77, 77, 77, 77, 77, 77, 77, 77, 77, 77, 77, 77, 77, 77, 77, 77, 77, 77, 77, 77, 77, 77, 77, 77, 77, 77, 77, 77, 77, 77, 77, 77, 77, 77, 77, 77, 77, 77, 77, 77, 77, 77, 77, 77, 77, 77, 77, 77, 195, 195, 195, 195, 195, 195, 255, 255, 255, 255, 255, 255, 255, 255, 255, 77, 77, 77, 77, 77, 77, 77, 77, 77, 77, 77, 77, 77, 77, 77, 77, 77, 77, 77, 77, 77, 77, 77, 77, 77, 77, 77, 77, 77, 77, 255, 255, 255, 255, 255, 255, 255, 255, 255, 255, 255, 255, 255, 255, 255, 255, 255, 255, 255, 255, 255, 77, 77, 77, 77, 77, 77, 77, 77, 77, 77, 77, 77, 77, 77, 77, 77, 77, 77, 77, 77, 77, 77, 77, 77, 77, 77, 77, 77, 77, 77, 77, 77, 77, 255, 255, 255, 255, 255, 255, 255, 255, 255, 255, 255, 255, 255, 255, 255, 221, 221, 221, 77, 77, 77, 77, 77, 77, 77, 77, 77, 77, 77, 77, 77, 77, 77, 77, 77, 77, 77, 77, 77, 77, 77, 77, 77, 77, 77, 77, 77, 77, 77, 77, 77, 77, 77, 77, 255, 255, 255, 255, 255, 255, 255, 255, 255, 255, 255, 255, 195, 195, 195, 77, 77, 77, 77, 77, 77, 77, 77, 77, 77, 77, 77, 77, 77, 77, 77, 77, 77, 77, 77, 77, 77, 77, 77, 77, 77, 77, 77, 77, 77, 77, 77, 77, 255, 255, 255, 255, 255, 255, 255, 255, 255, 255, 255, 255, 255, 255, 255, 127, 127, 127, 77, 77, 77, 77, 77, 77, 77, 77, 77, 77, 77, 77, 77, 77, 77, 77, 77, 77, 77, 77, 77, 77, 77, 77, 77, 77, 77, 77, 77, 77, 255, 255, 255, 255, 255, 255, 255, 255, 255, 77, 77, 77, 255, 255, 255, 255, 255, 255, 77, 77, 77, 77, 77, 77, 77, 77, 77, 77, 77, 77, 77, 77, 77, 77, 77, 77, 77, 77, 77, 77, 77, 77, 77, 77, 77, 77, 77, 77, 255, 255, 255, 255, 255, 255, 255, 255, 255, 77, 77, 77, 77, 77, 77, 77, 77, 77, 255, 255, 255, 77, 77, 77, 77, 77, 77, 77, 77, 77, 77, 77, 77, 77, 77, 77, 77, 77, 77, 77, 77, 77, 77, 77, 77, 77, 77, 77, 255, 255, 255, 255, 255, 255, 255, 255, 255, 77, 77, 77, 77, 77, 77, 77, 77, 77, 77, 77, 77, 77, 77, 77, 77, 77, 77, 77, 77, 77, 77, 77, 77, 77, 77, 77, 77, 77, 77, 77, 77, 77, 77, 77, 77, 77, 77, 77, 255, 255, 255, 255, 255, 255, 255, 255, 255, 77, 77, 77, 77, 77, 77, 77, 77, 77, 77, 77, 77, 77, 77, 77, 77, 77, 77, 77, 77, 77, 77, 77, 77, 77, 77, 77, 77, 77, 77, 77, 77, 77, 77, 77, 77, 77, 77, 77, 255, 255, 255, 255, 255, 255, 255, 255, 255, 77, 77, 77, 77, 77, 77, 77, 77, 77, 77, 77, 77, 77, 77, 77, 77, 77, 77, 77, 77, 77, 77, 77, 77, 77, 77, 77, 77, 77, 77, 77, 77, 77, 77, 77, 77, 77, 77, 77, 255, 255, 255, 255, 255, 255, 255, 255, 255, 77, 77, 77, 77, 77, 77, 77, 77, 77, 77, 77, 77, 77, 77, 77, 77, 77, 77, 77, 77, 77, 77, 77, 77, 77, 77, 77, 77, 77, 77, 77, 77, 77, 77, 77, 77, 77, 77, 77, 77, 77, 77, 255, 255, 255, 255, 255, 255, 77, 77, 77, 77, 77, 77, 77, 77, 77, 77, 77, 77, 77, 77, 77, 77, 77, 77, 77, 77, 77, 77, 77, 77, 77, 77, 77, 77, 77, 77, 77, 77, 77, 77, 77, 77, 77, 77, 77, 77, 77, 77, 77, 77, 77, 77, 77, 77, 77, 77, 77, 77, 77, 77, 77, 77, 77, 77, 77, 77, 77, 77, 77, 77, 77, 77, 77, 77, 77, 77, 77, 77, 77, 77, 77, 77, 77, 77, 77, 77, 77, 77, 77, 77, 77, 77, 77, 77, 77, 77, 77, 77, 77, 77, 77, 77, 77, 77, 77, 77, 77, 77, 77, 77, 77, 77, 77, 77, 77, 77, 77, 77, 77, 77, 77, 77, 77, 77, 77, 77, 77, 77, 77, 77, 77, 77, 77, 77, 77, 77, 77, 77, 77, 77, 77, 77, 77, 77, 77, 77, 77], "mask"=[], "colors"=[], "Rectangle"={"left"=0, "top"=0, "right"=17, "bottom"=17}}  # brown up arrow
        w507 = T55 {"image type"=0, "image depth"=24, "image"=[77, 77, 77, 77, 77, 77, 77, 77, 77, 77, 77, 77, 77, 77, 77, 77, 77, 77, 77, 77, 77, 77, 77, 77, 77, 77, 77, 77, 77, 77, 77, 77, 77, 77, 77, 77, 77, 77, 77, 77, 77, 77, 77, 77, 77, 77, 77, 77, 77, 77, 77, 77, 77, 77, 77, 77, 77, 77, 77, 77, 77, 77, 77, 77, 77, 77, 77, 77, 77, 77, 77, 77, 77, 77, 77, 77, 77, 77, 77, 77, 77, 77, 77, 77, 77, 77, 77, 249, 248, 249, 249, 244, 249, 77, 77, 77, 77, 77, 77, 77, 77, 77, 77, 77, 77, 77, 77, 77, 77, 77, 77, 77, 77, 77, 77, 77, 77, 77, 77, 77, 77, 77, 77, 77, 77, 77, 77, 77, 77, 77, 77, 77, 77, 77, 77, 255, 255, 255, 251, 250, 250, 255, 251, 255, 77, 77, 77, 77, 77, 77, 77, 77, 77, 77, 77, 77, 77, 77, 77, 77, 77, 77, 77, 77, 77, 77, 77, 77, 77, 77, 77, 77, 77, 77, 77, 77, 77, 77, 77, 77, 77, 77, 77, 77, 77, 77, 245, 244, 244, 243, 240, 241, 77, 77, 77, 77, 77, 77, 77, 77, 77, 77, 77, 77, 77, 77, 77, 77, 77, 77, 77, 77, 77, 77, 77, 77, 77, 77, 77, 77, 77, 77, 77, 77, 77, 77, 77, 77, 77, 77, 77, 77, 77, 77, 255, 251, 255, 245, 244, 244, 243, 240, 241, 77, 77, 77, 77, 77, 77, 77, 77, 77, 77, 77, 77, 77, 77, 77, 77, 77, 77, 77, 77, 77, 77, 77, 77, 77, 77, 77, 77, 77, 77, 77, 77, 77, 77, 77, 77, 77, 77, 77, 77, 77, 77, 244, 243, 243, 247, 241, 247, 170, 170, 170, 77, 77, 77, 77, 77, 77, 77, 77, 77, 77, 77, 77, 77, 77, 77, 77, 77, 77, 77, 77, 77, 77, 77, 77, 77, 77, 77, 77, 77, 77, 77, 77, 77, 77, 77, 77, 77, 77, 77, 250, 247, 250, 240, 235, 239, 247, 241, 247, 77, 77, 77, 77, 77, 77, 77, 77, 77, 77, 77, 77, 77, 77, 77, 77, 77, 77, 77, 77, 77, 77, 77, 77, 77, 77, 77, 77, 77, 77, 77, 77, 77, 77, 77, 77, 77, 77, 77, 77, 77, 77, 251, 245, 252, 245, 238, 245, 170, 170, 170, 77, 77, 77, 77, 77, 77, 77, 77, 77, 77, 77, 77, 77, 77, 77, 77, 77, 77, 77, 77, 77, 77, 77, 77, 77, 77, 77, 77, 77, 77, 77, 77, 77, 77, 77, 77, 77, 77, 77, 246, 243, 245, 239, 237, 238, 221, 222, 220, 77, 77, 77, 77, 77, 77, 77, 77, 77, 77, 77, 77, 77, 77, 77, 77, 77, 77, 77, 77, 77, 77, 77, 77, 255, 255, 255, 255, 255, 255, 255, 255, 255, 77, 77, 77, 77, 77, 77, 77, 77, 77, 239, 236, 238, 232, 230, 230, 77, 77, 77, 77, 77, 77, 77, 77, 77, 77, 77, 77, 77, 77, 77, 77, 77, 77, 77, 77, 77, 77, 77, 77, 77, 77, 77, 170, 170, 170, 255, 255, 255, 255, 255, 255, 77, 77, 77, 77, 77, 77, 249, 241, 249, 233, 231, 231, 237, 231, 236, 77, 77, 77, 77, 77, 77, 77, 77, 77, 77, 77, 77, 77, 77, 77, 77, 77, 77, 77, 77, 77, 77, 77, 77, 77, 77, 77, 77, 77, 77, 255, 255, 255, 255, 255, 255, 237, 243, 234, 221, 231, 218, 237, 234, 236, 230, 228, 228, 170, 170, 170, 77, 77, 77, 77, 77, 77, 77, 77, 77, 77, 77, 77, 77, 77, 77, 77, 77, 77, 77, 77, 77, 77, 77, 77, 77, 77, 77, 77, 77, 77, 77, 77, 77, 170, 170, 170, 234, 232, 232, 230, 229, 229, 229, 226, 227, 217, 216, 215, 77, 77, 77, 77, 77, 77, 77, 77, 77, 77, 77, 77, 77, 77, 77, 77, 77, 77, 77, 77, 77, 77, 77, 77, 77, 77, 77, 77, 77, 77, 77, 77, 77, 77, 77, 77, 170, 170, 170, 234, 232, 232, 230, 229, 229, 229, 226, 227, 77, 77, 77, 77, 77, 77, 77, 77, 77, 77, 77, 77, 77, 77, 77, 77, 77, 77, 77, 77, 77, 77, 77, 77, 77, 77, 77, 77, 77, 77, 77, 77, 77, 77, 77, 77, 77, 77, 77, 77, 77, 77, 237, 232, 236, 234, 229, 233, 170, 170, 170, 77, 77, 77, 77, 77, 77, 77, 77, 77, 77, 77, 77, 77, 77, 77, 77, 77, 77, 77, 77, 77, 77, 77, 77, 77, 77, 77, 77, 77, 77, 77, 77, 77, 77, 77, 77, 77, 77, 77, 77, 77, 77, 77, 77, 77, 77, 77, 77, 77, 77, 77, 77, 77, 77, 77, 77, 77, 77, 77, 77, 77, 77, 77, 77, 77, 77, 77, 77, 77, 77, 77, 77, 77, 77, 77, 77, 77, 77, 77, 77, 77, 77, 77, 77, 77, 77, 77, 77, 77, 77, 77, 77, 77, 77, 77, 77, 77, 77, 77, 77, 77, 77, 77, 77, 77, 77, 77, 77, 77, 77, 77, 77, 77, 77, 77, 77, 77, 77, 77, 77, 77, 77, 77, 77, 77, 77, 77, 77, 77], "mask"=[], "colors"=[], "Rectangle"={"left"=0, "top"=0, "right"=17, "bottom"=17}}  # brown ok
        w501 = T55 {"image type"=0, "image depth"=24, "image"=[77, 77, 77, 77, 77, 77, 77, 77, 77, 77, 77, 77, 77, 77, 77, 77, 77, 77, 77, 77, 77, 77, 77, 77, 77, 77, 77, 77, 77, 77, 77, 77, 77, 77, 77, 77, 77, 77, 77, 77, 77, 77, 77, 77, 77, 77, 77, 77, 77, 77, 77, 77, 77, 77, 77, 77, 77, 77, 77, 77, 77, 77, 77, 77, 77, 77, 77, 77, 77, 77, 77, 77, 77, 77, 77, 77, 77, 77, 77, 77, 77, 77, 77, 77, 77, 77, 77, 77, 77, 77, 77, 77, 77, 77, 77, 77, 77, 77, 77, 77, 77, 77, 77, 77, 77, 77, 77, 77, 77, 77, 77, 77, 77, 77, 77, 77, 77, 77, 77, 77, 77, 77, 77, 77, 77, 77, 77, 77, 77, 77, 77, 77, 77, 77, 77, 77, 77, 77, 77, 77, 77, 153, 204, 51, 153, 204, 51, 77, 77, 77, 77, 77, 77, 77, 77, 77, 77, 77, 77, 77, 77, 77, 77, 77, 77, 77, 77, 77, 77, 77, 77, 77, 77, 77, 77, 77, 77, 77, 77, 77, 77, 77, 77, 77, 77, 77, 77, 77, 77, 153, 204, 51, 153, 204, 51, 153, 204, 51, 77, 77, 77, 77, 77, 77, 77, 77, 77, 77, 77, 77, 77, 77, 77, 77, 77, 77, 77, 77, 77, 77, 77, 77, 77, 77, 77, 77, 77, 77, 77, 77, 77, 77, 77, 77, 77, 77, 77, 77, 77, 77, 153, 204, 51, 153, 204, 51, 99, 156, 0, 77, 77, 77, 77, 77, 77, 77, 77, 77, 77, 77, 77, 77, 77, 77, 77, 77, 77, 77, 77, 77, 77, 77, 77, 77, 77, 77, 77, 77, 77, 77, 77, 77, 77, 77, 77, 77, 77, 77, 153, 204, 51, 153, 204, 51, 153, 204, 51, 77, 77, 77, 77, 77, 77, 77, 77, 77, 77, 77, 77, 77, 77, 77, 77, 77, 77, 77, 77, 77, 77, 77, 77, 77, 77, 77, 77, 77, 77, 77, 77, 77, 77, 77, 77, 77, 77, 77, 77, 77, 77, 153, 204, 51, 153, 204, 51, 99, 156, 0, 77, 77, 77, 77, 77, 77, 77, 77, 77, 77, 77, 77, 77, 77, 77, 77, 77, 77, 77, 77, 77, 77, 77, 77, 77, 77, 77, 77, 77, 77, 77, 77, 77, 77, 77, 77, 77, 77, 77, 153, 204, 51, 153, 204, 51, 153, 204, 51, 77, 77, 77, 77, 77, 77, 77, 77, 77, 77, 77, 77, 77, 77, 77, 77, 77, 77, 77, 77, 77, 77, 77, 77, 77, 77, 77, 77, 77, 77, 77, 77, 77, 77, 77, 77, 77, 77, 77, 77, 77, 77, 153, 204, 51, 153, 204, 51, 99, 156, 0, 77, 77, 77, 77, 77, 77, 77, 77, 77, 77, 77, 77, 77, 77, 77, 77, 77, 77, 77, 77, 77, 77, 77, 77, 77, 77, 77, 77, 77, 77, 77, 77, 77, 77, 77, 77, 77, 77, 77, 153, 204, 51, 153, 204, 51, 153, 204, 51, 77, 77, 77, 77, 77, 77, 77, 77, 77, 77, 77, 77, 77, 77, 77, 77, 77, 77, 77, 77, 77, 77, 77, 77, 153, 204, 51, 153, 204, 51, 153, 204, 51, 77, 77, 77, 77, 77, 77, 77, 77, 77, 153, 204, 51, 153, 204, 51, 99, 156, 0, 77, 77, 77, 77, 77, 77, 77, 77, 77, 77, 77, 77, 77, 77, 77, 77, 77, 77, 77, 77, 77, 77, 77, 77, 99, 156, 0, 153, 204, 51, 153, 204, 51, 77, 77, 77, 77, 77, 77, 153, 204, 51, 153, 204, 51, 153, 204, 51, 77, 77, 77, 77, 77, 77, 77, 77, 77, 77, 77, 77, 77, 77, 77, 77, 77, 77, 77, 77, 77, 77, 77, 77, 77, 77, 77, 77, 77, 77, 153, 204, 51, 153, 204, 51, 153, 204, 51, 153, 204, 51, 153, 204, 51, 153, 204, 51, 99, 156, 0, 77, 77, 77, 77, 77, 77, 77, 77, 77, 77, 77, 77, 77, 77, 77, 77, 77, 77, 77, 77, 77, 77, 77, 77, 77, 77, 77, 77, 77, 77, 77, 77, 77, 99, 156, 0, 153, 204, 51, 153, 204, 51, 153, 204, 51, 99, 156, 0, 77, 77, 77, 77, 77, 77, 77, 77, 77, 77, 77, 77, 77, 77, 77, 77, 77, 77, 77, 77, 77, 77, 77, 77, 77, 77, 77, 77, 77, 77, 77, 77, 77, 77, 77, 77, 99, 156, 0, 153, 204, 51, 153, 204, 51, 153, 204, 51, 77, 77, 77, 77, 77, 77, 77, 77, 77, 77, 77, 77, 77, 77, 77, 77, 77, 77, 77, 77, 77, 77, 77, 77, 77, 77, 77, 77, 77, 77, 77, 77, 77, 77, 77, 77, 77, 77, 77, 77, 77, 77, 153, 204, 51, 153, 204, 51, 99, 156, 0, 77, 77, 77, 77, 77, 77, 77, 77, 77, 77, 77, 77, 77, 77, 77, 77, 77, 77, 77, 77, 77, 77, 77, 77, 77, 77, 77, 77, 77, 77, 77, 77, 77, 77, 77, 77, 77, 77, 77, 77, 77, 77, 77, 77, 77, 77, 77, 77, 77, 77, 77, 77, 77, 77, 77, 77, 77, 77, 77, 77, 77, 77, 77, 77, 77, 77, 77, 77, 77, 77, 77, 77, 77, 77, 77], "mask"=[], "colors"=[], "Rectangle"={"left"=0, "top"=0, "right"=17, "bottom"=17}}  # brown ok green down
        w502 = T55 {"image type"=0, "image depth"=24, "image"=[77, 77, 77, 77, 77, 77, 77, 77, 77, 77, 77, 77, 77, 77, 77, 77, 77, 77, 77, 77, 77, 77, 77, 77, 77, 77, 77, 77, 77, 77, 77, 77, 77, 77, 77, 77, 77, 77, 77, 77, 77, 77, 77, 77, 77, 77, 77, 77, 77, 77, 77, 77, 77, 77, 77, 77, 77, 77, 77, 77, 77, 77, 77, 77, 77, 77, 77, 77, 77, 77, 77, 77, 77, 77, 77, 77, 77, 77, 77, 77, 77, 77, 77, 77, 77, 77, 77, 77, 77, 77, 77, 77, 77, 77, 77, 77, 77, 77, 77, 77, 77, 77, 77, 77, 77, 77, 77, 77, 77, 77, 77, 77, 77, 77, 77, 77, 77, 77, 77, 77, 77, 77, 77, 77, 77, 77, 77, 77, 77, 77, 77, 77, 77, 77, 77, 77, 77, 77, 77, 77, 77, 249, 248, 249, 249, 244, 249, 77, 77, 77, 77, 77, 77, 77, 77, 77, 77, 77, 77, 77, 77, 77, 77, 77, 77, 77, 77, 77, 77, 77, 77, 77, 77, 77, 77, 77, 77, 77, 77, 77, 77, 77, 77, 77, 77, 77, 77, 77, 77, 255, 255, 255, 251, 250, 250, 255, 251, 255, 77, 77, 77, 77, 77, 77, 77, 77, 77, 77, 77, 77, 77, 77, 77, 77, 77, 77, 77, 77, 77, 77, 77, 77, 77, 77, 77, 77, 77, 77, 77, 77, 77, 77, 77, 77, 77, 77, 77, 77, 77, 77, 245, 244, 244, 243, 240, 241, 77, 77, 77, 77, 77, 77, 77, 77, 77, 77, 77, 77, 77, 77, 77, 77, 77, 77, 77, 77, 77, 77, 77, 77, 77, 77, 77, 77, 77, 77, 77, 77, 77, 77, 77, 77, 77, 77, 77, 77, 77, 77, 255, 251, 255, 245, 244, 244, 243, 240, 241, 77, 77, 77, 77, 77, 77, 77, 77, 77, 77, 77, 77, 77, 77, 77, 77, 77, 77, 77, 77, 77, 77, 77, 77, 77, 77, 77, 77, 77, 77, 77, 77, 77, 77, 77, 77, 77, 77, 77, 77, 77, 77, 244, 243, 243, 247, 241, 247, 170, 170, 170, 77, 77, 77, 77, 77, 77, 77, 77, 77, 77, 77, 77, 77, 77, 77, 77, 77, 77, 77, 77, 77, 77, 77, 77, 77, 77, 77, 77, 77, 77, 77, 77, 77, 77, 77, 77, 77, 77, 77, 250, 247, 250, 240, 235, 239, 247, 241, 247, 77, 77, 77, 77, 77, 77, 77, 77, 77, 77, 77, 77, 77, 77, 77, 77, 77, 77, 77, 77, 77, 77, 77, 77, 77, 77, 77, 77, 77, 77, 77, 77, 77, 77, 77, 77, 77, 77, 77, 77, 77, 77, 251, 245, 252, 245, 238, 245, 170, 170, 170, 77, 77, 77, 77, 77, 77, 77, 77, 77, 77, 77, 77, 77, 77, 77, 77, 77, 77, 77, 77, 77, 77, 77, 77, 77, 77, 77, 77, 77, 77, 77, 77, 77, 77, 77, 77, 77, 77, 77, 246, 243, 245, 239, 237, 238, 221, 222, 220, 77, 77, 77, 77, 77, 77, 77, 77, 77, 77, 77, 77, 77, 77, 77, 77, 77, 77, 77, 77, 77, 77, 77, 77, 255, 255, 255, 255, 255, 255, 255, 255, 255, 77, 77, 77, 77, 77, 77, 77, 77, 77, 239, 236, 238, 232, 230, 230, 77, 77, 77, 77, 77, 77, 77, 77, 77, 77, 77, 77, 77, 77, 77, 77, 77, 77, 77, 77, 77, 77, 77, 77, 77, 77, 77, 170, 170, 170, 255, 255, 255, 255, 255, 255, 77, 77, 77, 77, 77, 77, 249, 241, 249, 233, 231, 231, 237, 231, 236, 77, 77, 77, 77, 77, 77, 77, 77, 77, 77, 77, 77, 77, 77, 77, 77, 77, 77, 77, 77, 77, 77, 77, 77, 77, 77, 77, 77, 77, 77, 255, 255, 255, 255, 255, 255, 237, 243, 234, 221, 231, 218, 237, 234, 236, 230, 228, 228, 170, 170, 170, 77, 77, 77, 77, 77, 77, 77, 77, 77, 77, 77, 77, 77, 77, 77, 77, 77, 77, 77, 77, 77, 77, 77, 77, 77, 77, 77, 77, 77, 77, 77, 77, 77, 170, 170, 170, 234, 232, 232, 230, 229, 229, 229, 226, 227, 217, 216, 215, 77, 77, 77, 77, 77, 77, 77, 77, 77, 77, 77, 77, 77, 77, 77, 77, 77, 77, 77, 77, 77, 77, 77, 77, 77, 77, 77, 77, 77, 77, 77, 77, 77, 77, 77, 77, 170, 170, 170, 234, 232, 232, 230, 229, 229, 229, 226, 227, 77, 77, 77, 77, 77, 77, 77, 77, 77, 77, 77, 77, 77, 77, 77, 77, 77, 77, 77, 77, 77, 77, 77, 77, 77, 77, 77, 77, 77, 77, 77, 77, 77, 77, 77, 77, 77, 77, 77, 77, 77, 77, 237, 232, 236, 234, 229, 233, 170, 170, 170, 77, 77, 77, 77, 77, 77, 77, 77, 77, 77, 77, 77, 77, 77, 77, 77, 77, 77, 77, 77, 77, 77, 77, 77, 77, 77, 77, 77, 77, 77, 77, 77, 77, 77, 77, 77, 77, 77, 77, 77, 77, 77, 77, 77, 77, 77, 77, 77, 77, 77, 77, 77, 77, 77, 77, 77, 77, 77, 77, 77, 77, 77, 77, 77, 77, 77, 77, 77, 77, 77, 77, 77, 77, 77, 77], "mask"=[], "colors"=[], "Rectangle"={"left"=0, "top"=0, "right"=17, "bottom"=17}}  # brown ok down
        w506 = T55 {"image type"=0, "image depth"=24, "image"=[18, 179, 255, 18, 179, 255, 18, 179, 255, 18, 179, 255, 18, 179, 255, 18, 179, 255, 18, 179, 255, 18, 179, 255, 18, 179, 255, 18, 179, 255, 18, 179, 255, 18, 179, 255, 18, 179, 255, 18, 179, 255, 18, 179, 255, 18, 179, 255, 18, 179, 255, 18, 179, 255, 18, 179, 255, 18, 179, 255, 18, 179, 255, 18, 179, 255, 18, 179, 255, 18, 179, 255, 18, 179, 255, 18, 179, 255, 18, 179, 255, 18, 179, 255, 18, 179, 255, 18, 179, 255, 18, 179, 255, 18, 179, 255, 18, 179, 255, 18, 179, 255, 18, 179, 255, 18, 179, 255, 18, 179, 255, 18, 179, 255, 18, 179, 255, 18, 179, 255, 18, 179, 255, 18, 179, 255, 18, 179, 255, 18, 179, 255, 18, 179, 255, 18, 179, 255, 18, 179, 255, 18, 179, 255, 18, 179, 255, 18, 179, 255, 18, 179, 255, 18, 179, 255, 18, 179, 255, 18, 179, 255, 18, 179, 255, 18, 179, 255, 18, 179, 255, 18, 179, 255, 18, 179, 255, 18, 179, 255, 18, 179, 255, 18, 179, 255, 18, 179, 255, 18, 179, 255, 18, 179, 255, 18, 179, 255, 18, 179, 255, 18, 179, 255, 18, 179, 255, 18, 179, 255, 18, 179, 255, 18, 179, 255, 18, 179, 255, 18, 179, 255, 18, 179, 255, 18, 179, 255, 18, 179, 255, 18, 179, 255, 18, 179, 255, 18, 179, 255, 18, 179, 255, 18, 179, 255, 18, 179, 255, 18, 179, 255, 18, 179, 255, 18, 179, 255, 18, 179, 255, 18, 179, 255, 18, 179, 255, 18, 179, 255, 18, 179, 255, 18, 179, 255, 18, 179, 255, 18, 179, 255, 18, 179, 255, 18, 179, 255, 18, 179, 255, 18, 179, 255, 18, 179, 255, 18, 179, 255, 18, 179, 255, 18, 179, 255, 18, 179, 255, 18, 179, 255, 18, 179, 255, 18, 179, 255, 18, 179, 255, 18, 179, 255, 18, 179, 255, 18, 179, 255, 18, 179, 255, 18, 179, 255, 18, 179, 255, 18, 179, 255, 18, 179, 255, 18, 179, 255, 18, 179, 255, 18, 179, 255, 18, 179, 255, 18, 179, 255, 18, 179, 255, 18, 179, 255, 18, 179, 255, 18, 179, 255, 18, 179, 255, 18, 179, 255, 18, 179, 255, 18, 179, 255, 18, 179, 255, 18, 179, 255, 18, 179, 255, 18, 179, 255, 18, 179, 255, 18, 179, 255, 18, 179, 255, 18, 179, 255, 18, 179, 255, 18, 179, 255, 18, 179, 255, 18, 179, 255, 18, 179, 255, 18, 179, 255, 18, 179, 255, 18, 179, 255, 18, 179, 255, 18, 179, 255, 18, 179, 255, 18, 179, 255, 18, 179, 255, 18, 179, 255, 18, 179, 255, 18, 179, 255, 18, 179, 255, 18, 179, 255, 18, 179, 255, 18, 179, 255, 18, 179, 255, 18, 179, 255, 18, 179, 255, 18, 179, 255, 18, 179, 255, 18, 179, 255, 18, 179, 255, 18, 179, 255, 18, 179, 255, 18, 179, 255, 18, 179, 255, 18, 179, 255, 18, 179, 255, 18, 179, 255, 18, 179, 255, 18, 179, 255, 18, 179, 255, 18, 179, 255, 18, 179, 255, 18, 179, 255, 18, 179, 255, 18, 179, 255, 18, 179, 255, 18, 179, 255, 18, 179, 255, 18, 179, 255, 18, 179, 255, 18, 179, 255, 18, 179, 255, 18, 179, 255, 18, 179, 255, 18, 179, 255, 18, 179, 255, 18, 179, 255, 18, 179, 255, 18, 179, 255, 18, 179, 255, 18, 179, 255, 18, 179, 255, 18, 179, 255, 18, 179, 255, 18, 179, 255, 18, 179, 255, 18, 179, 255, 18, 179, 255, 18, 179, 255, 18, 179, 255, 18, 179, 255, 18, 179, 255, 18, 179, 255, 18, 179, 255, 18, 179, 255, 18, 179, 255, 18, 179, 255, 18, 179, 255, 18, 179, 255, 18, 179, 255, 18, 179, 255, 18, 179, 255, 18, 179, 255, 18, 179, 255, 18, 179, 255, 18, 179, 255, 18, 179, 255, 18, 179, 255, 18, 179, 255, 18, 179, 255, 18, 179, 255, 18, 179, 255, 18, 179, 255, 18, 179, 255, 18, 179, 255, 18, 179, 255, 18, 179, 255, 18, 179, 255, 18, 179, 255, 18, 179, 255, 18, 179, 255, 18, 179, 255, 18, 179, 255, 18, 179, 255, 18, 179, 255, 18, 179, 255, 18, 179, 255, 18, 179, 255, 18, 179, 255, 18, 179, 255, 18, 179, 255, 18, 179, 255, 18, 179, 255, 18, 179, 255, 18, 179, 255, 18, 179, 255, 18, 179, 255, 18, 179, 255, 18, 179, 255, 18, 179, 255, 18, 179, 255, 18, 179, 255, 18, 179, 255, 18, 179, 255, 18, 179, 255, 18, 179, 255, 18, 179, 255, 18, 179, 255, 18, 179, 255, 18, 179, 255, 18, 179, 255, 18, 179, 255, 18, 179, 255, 18, 179, 255, 18, 179, 255, 18, 179, 255, 18, 179, 255, 18, 179, 255, 18, 179, 255, 18, 179, 255, 18, 179, 255, 18, 179, 255, 18, 179, 255, 18, 179, 255, 18, 179, 255, 18, 179, 255, 18, 179, 255, 18, 179, 255, 18, 179, 255, 18, 179, 255, 18, 179, 255, 18, 179, 255, 18, 179, 255, 18, 179, 255, 18, 179, 255, 18, 179, 255], "mask"=[], "colors"=[], "Rectangle"={"left"=0, "top"=0, "right"=17, "bottom"=17}}  # blue
        w511 = T55 {"image type"=0, "image depth"=0, "image"=[], "mask"=[], "colors"=[], "Rectangle"={"left"=0, "top"=0, "right"=0, "bottom"=0}}  # element
        w505 = T55 {"image type"=0, "image depth"=24, "image"=[18, 179, 255, 18, 179, 255, 18, 179, 255, 18, 179, 255, 18, 179, 255, 18, 179, 255, 18, 179, 255, 18, 179, 255, 18, 179, 255, 18, 179, 255, 18, 179, 255, 18, 179, 255, 18, 179, 255, 18, 179, 255, 18, 179, 255, 18, 179, 255, 18, 179, 255, 18, 179, 255, 18, 179, 255, 18, 179, 255, 18, 179, 255, 18, 179, 255, 18, 179, 255, 18, 179, 255, 18, 179, 255, 18, 179, 255, 18, 179, 255, 18, 179, 255, 18, 179, 255, 18, 179, 255, 18, 179, 255, 18, 179, 255, 18, 179, 255, 18, 179, 255, 18, 179, 255, 18, 179, 255, 18, 179, 255, 18, 179, 255, 18, 179, 255, 18, 179, 255, 18, 179, 255, 18, 179, 255, 18, 179, 255, 18, 179, 255, 18, 179, 255, 18, 179, 255, 18, 179, 255, 18, 179, 255, 18, 179, 255, 18, 179, 255, 18, 179, 255, 18, 179, 255, 18, 179, 255, 18, 179, 255, 18, 179, 255, 18, 179, 255, 18, 179, 255, 18, 179, 255, 18, 179, 255, 18, 179, 255, 53, 189, 255, 98, 204, 255, 255, 255, 255, 255, 255, 255, 255, 255, 255, 18, 179, 255, 18, 179, 255, 18, 179, 255, 18, 179, 255, 18, 179, 255, 18, 179, 255, 18, 179, 255, 18, 179, 255, 18, 179, 255, 18, 179, 255, 255, 255, 255, 255, 255, 255, 255, 255, 255, 255, 255, 255, 255, 255, 255, 255, 255, 255, 255, 255, 255, 18, 179, 255, 18, 179, 255, 18, 179, 255, 18, 179, 255, 18, 179, 255, 18, 179, 255, 18, 179, 255, 18, 179, 255, 18, 179, 255, 18, 179, 255, 18, 179, 255, 255, 255, 255, 255, 255, 255, 255, 255, 255, 255, 255, 255, 255, 255, 255, 255, 255, 255, 18, 179, 255, 18, 179, 255, 18, 179, 255, 18, 179, 255, 18, 179, 255, 18, 179, 255, 18, 179, 255, 18, 179, 255, 18, 179, 255, 18, 179, 255, 18, 179, 255, 18, 179, 255, 255, 255, 255, 255, 255, 255, 255, 255, 255, 255, 255, 255, 98, 204, 255, 18, 179, 255, 18, 179, 255, 18, 179, 255, 18, 179, 255, 18, 179, 255, 18, 179, 255, 18, 179, 255, 18, 179, 255, 18, 179, 255, 18, 179, 255, 18, 179, 255, 255, 255, 255, 255, 255, 255, 255, 255, 255, 255, 255, 255, 255, 255, 255, 53, 189, 255, 18, 179, 255, 18, 179, 255, 18, 179, 255, 18, 179, 255, 18, 179, 255, 18, 179, 255, 18, 179, 255, 18, 179, 255, 18, 179, 255, 18, 179, 255, 255, 255, 255, 255, 255, 255, 255, 255, 255, 18, 179, 255, 255, 255, 255, 255, 255, 255, 18, 179, 255, 18, 179, 255, 18, 179, 255, 18, 179, 255, 18, 179, 255, 18, 179, 255, 18, 179, 255, 18, 179, 255, 18, 179, 255, 18, 179, 255, 255, 255, 255, 255, 255, 255, 255, 255, 255, 18, 179, 255, 18, 179, 255, 18, 179, 255, 255, 255, 255, 18, 179, 255, 18, 179, 255, 18, 179, 255, 18, 179, 255, 18, 179, 255, 18, 179, 255, 18, 179, 255, 18, 179, 255, 18, 179, 255, 255, 255, 255, 255, 255, 255, 255, 255, 255, 18, 179, 255, 18, 179, 255, 18, 179, 255, 18, 179, 255, 18, 179, 255, 18, 179, 255, 18, 179, 255, 18, 179, 255, 18, 179, 255, 18, 179, 255, 18, 179, 255, 18, 179, 255, 18, 179, 255, 255, 255, 255, 255, 255, 255, 255, 255, 255, 18, 179, 255, 18, 179, 255, 18, 179, 255, 18, 179, 255, 18, 179, 255, 18, 179, 255, 18, 179, 255, 18, 179, 255, 18, 179, 255, 18, 179, 255, 18, 179, 255, 18, 179, 255, 18, 179, 255, 255, 255, 255, 255, 255, 255, 255, 255, 255, 18, 179, 255, 18, 179, 255, 18, 179, 255, 18, 179, 255, 18, 179, 255, 18, 179, 255, 18, 179, 255, 18, 179, 255, 18, 179, 255, 18, 179, 255, 18, 179, 255, 18, 179, 255, 18, 179, 255, 255, 255, 255, 255, 255, 255, 255, 255, 255, 18, 179, 255, 18, 179, 255, 18, 179, 255, 18, 179, 255, 18, 179, 255, 18, 179, 255, 18, 179, 255, 18, 179, 255, 18, 179, 255, 18, 179, 255, 18, 179, 255, 18, 179, 255, 18, 179, 255, 18, 179, 255, 255, 255, 255, 255, 255, 255, 18, 179, 255, 18, 179, 255, 18, 179, 255, 18, 179, 255, 18, 179, 255, 18, 179, 255, 18, 179, 255, 18, 179, 255, 18, 179, 255, 18, 179, 255, 18, 179, 255, 18, 179, 255, 18, 179, 255, 18, 179, 255, 18, 179, 255, 18, 179, 255, 18, 179, 255, 18, 179, 255, 18, 179, 255, 18, 179, 255, 18, 179, 255, 18, 179, 255, 18, 179, 255, 18, 179, 255, 18, 179, 255, 18, 179, 255, 18, 179, 255, 18, 179, 255, 18, 179, 255, 18, 179, 255, 18, 179, 255, 18, 179, 255, 18, 179, 255, 18, 179, 255, 18, 179, 255, 18, 179, 255, 18, 179, 255, 18, 179, 255, 18, 179, 255, 18, 179, 255, 18, 179, 255, 18, 179, 255, 18, 179, 255, 18, 179, 255, 18, 179, 255, 18, 179, 255, 18, 179, 255], "mask"=[], "colors"=[], "Rectangle"={"left"=0, "top"=0, "right"=17, "bottom"=17}}  # blue up arrow
        w503 = T55 {"image type"=0, "image depth"=24, "image"=[18, 179, 255, 18, 179, 255, 18, 179, 255, 18, 179, 255, 18, 179, 255, 18, 179, 255, 18, 179, 255, 18, 179, 255, 18, 179, 255, 18, 179, 255, 18, 179, 255, 18, 179, 255, 18, 179, 255, 18, 179, 255, 18, 179, 255, 18, 179, 255, 18, 179, 255, 18, 179, 255, 18, 179, 255, 18, 179, 255, 18, 179, 255, 18, 179, 255, 18, 179, 255, 18, 179, 255, 18, 179, 255, 18, 179, 255, 18, 179, 255, 18, 179, 255, 18, 179, 255, 18, 179, 255, 18, 179, 255, 18, 179, 255, 18, 179, 255, 18, 179, 255, 18, 179, 255, 18, 179, 255, 18, 179, 255, 18, 179, 255, 18, 179, 255, 18, 179, 255, 18, 179, 255, 18, 179, 255, 18, 179, 255, 18, 179, 255, 18, 179, 255, 18, 179, 255, 18, 179, 255, 249, 248, 249, 249, 244, 249, 18, 179, 255, 18, 179, 255, 18, 179, 255, 18, 179, 255, 18, 179, 255, 18, 179, 255, 18, 179, 255, 18, 179, 255, 18, 179, 255, 18, 179, 255, 18, 179, 255, 18, 179, 255, 18, 179, 255, 18, 179, 255, 255, 255, 255, 251, 250, 250, 255, 251, 255, 18, 179, 255, 18, 179, 255, 18, 179, 255, 18, 179, 255, 18, 179, 255, 18, 179, 255, 18, 179, 255, 18, 179, 255, 18, 179, 255, 18, 179, 255, 18, 179, 255, 18, 179, 255, 18, 179, 255, 18, 179, 255, 245, 244, 244, 243, 240, 241, 18, 179, 255, 18, 179, 255, 18, 179, 255, 18, 179, 255, 18, 179, 255, 18, 179, 255, 18, 179, 255, 18, 179, 255, 18, 179, 255, 18, 179, 255, 18, 179, 255, 18, 179, 255, 18, 179, 255, 18, 179, 255, 255, 251, 255, 245, 244, 244, 243, 240, 241, 18, 179, 255, 18, 179, 255, 18, 179, 255, 18, 179, 255, 18, 179, 255, 18, 179, 255, 18, 179, 255, 18, 179, 255, 18, 179, 255, 18, 179, 255, 18, 179, 255, 18, 179, 255, 18, 179, 255, 18, 179, 255, 244, 243, 243, 247, 241, 247, 98, 204, 255, 18, 179, 255, 18, 179, 255, 18, 179, 255, 18, 179, 255, 18, 179, 255, 18, 179, 255, 18, 179, 255, 18, 179, 255, 18, 179, 255, 18, 179, 255, 18, 179, 255, 18, 179, 255, 18, 179, 255, 250, 247, 250, 240, 235, 239, 247, 241, 247, 18, 179, 255, 18, 179, 255, 18, 179, 255, 18, 179, 255, 18, 179, 255, 18, 179, 255, 18, 179, 255, 18, 179, 255, 18, 179, 255, 18, 179, 255, 18, 179, 255, 18, 179, 255, 18, 179, 255, 18, 179, 255, 251, 245, 252, 245, 238, 245, 98, 204, 255, 18, 179, 255, 18, 179, 255, 18, 179, 255, 18, 179, 255, 18, 179, 255, 18, 179, 255, 18, 179, 255, 18, 179, 255, 18, 179, 255, 18, 179, 255, 18, 179, 255, 18, 179, 255, 18, 179, 255, 246, 243, 245, 239, 237, 238, 221, 222, 220, 18, 179, 255, 18, 179, 255, 18, 179, 255, 18, 179, 255, 18, 179, 255, 18, 179, 255, 18, 179, 255, 18, 179, 255, 255, 255, 255, 255, 255, 255, 255, 255, 255, 18, 179, 255, 18, 179, 255, 18, 179, 255, 239, 236, 238, 232, 230, 230, 18, 179, 255, 18, 179, 255, 18, 179, 255, 18, 179, 255, 18, 179, 255, 18, 179, 255, 18, 179, 255, 18, 179, 255, 18, 179, 255, 98, 204, 255, 255, 255, 255, 255, 255, 255, 18, 179, 255, 18, 179, 255, 249, 241, 249, 233, 231, 231, 237, 231, 236, 18, 179, 255, 18, 179, 255, 18, 179, 255, 18, 179, 255, 18, 179, 255, 18, 179, 255, 18, 179, 255, 18, 179, 255, 18, 179, 255, 18, 179, 255, 255, 255, 255, 255, 255, 255, 237, 243, 234, 221, 231, 218, 237, 234, 236, 230, 228, 228, 98, 204, 255, 18, 179, 255, 18, 179, 255, 18, 179, 255, 18, 179, 255, 18, 179, 255, 18, 179, 255, 18, 179, 255, 18, 179, 255, 18, 179, 255, 18, 179, 255, 18, 179, 255, 98, 204, 255, 234, 232, 232, 230, 229, 229, 229, 226, 227, 98, 204, 255, 18, 179, 255, 18, 179, 255, 18, 179, 255, 18, 179, 255, 18, 179, 255, 18, 179, 255, 18, 179, 255, 18, 179, 255, 18, 179, 255, 18, 179, 255, 18, 179, 255, 18, 179, 255, 98, 204, 255, 234, 232, 232, 230, 229, 229, 229, 226, 227, 18, 179, 255, 18, 179, 255, 18, 179, 255, 18, 179, 255, 18, 179, 255, 18, 179, 255, 18, 179, 255, 18, 179, 255, 18, 179, 255, 18, 179, 255, 18, 179, 255, 18, 179, 255, 18, 179, 255, 18, 179, 255, 237, 232, 236, 234, 229, 233, 98, 204, 255, 18, 179, 255, 18, 179, 255, 18, 179, 255, 18, 179, 255, 18, 179, 255, 18, 179, 255, 18, 179, 255, 18, 179, 255, 18, 179, 255, 18, 179, 255, 18, 179, 255, 18, 179, 255, 18, 179, 255, 18, 179, 255, 18, 179, 255, 18, 179, 255, 18, 179, 255, 18, 179, 255, 18, 179, 255, 18, 179, 255, 18, 179, 255, 18, 179, 255, 18, 179, 255, 18, 179, 255, 18, 179, 255], "mask"=[], "colors"=[], "Rectangle"={"left"=0, "top"=0, "right"=17, "bottom"=17}}  # blue ok down
        w504 = T55 {"image type"=0, "image depth"=24, "image"=[18, 179, 255, 18, 179, 255, 18, 179, 255, 18, 179, 255, 18, 179, 255, 18, 179, 255, 18, 179, 255, 18, 179, 255, 18, 179, 255, 18, 179, 255, 18, 179, 255, 18, 179, 255, 18, 179, 255, 18, 179, 255, 18, 179, 255, 18, 179, 255, 18, 179, 255, 18, 179, 255, 18, 179, 255, 18, 179, 255, 18, 179, 255, 18, 179, 255, 18, 179, 255, 18, 179, 255, 18, 179, 255, 18, 179, 255, 18, 179, 255, 18, 179, 255, 18, 179, 255, 18, 179, 255, 18, 179, 255, 18, 179, 255, 18, 179, 255, 18, 179, 255, 18, 179, 255, 18, 179, 255, 255, 255, 255, 255, 255, 255, 18, 179, 255, 18, 179, 255, 18, 179, 255, 18, 179, 255, 18, 179, 255, 18, 179, 255, 18, 179, 255, 18, 179, 255, 18, 179, 255, 18, 179, 255, 18, 179, 255, 18, 179, 255, 18, 179, 255, 18, 179, 255, 18, 179, 255, 255, 255, 255, 255, 255, 255, 255, 255, 255, 18, 179, 255, 18, 179, 255, 18, 179, 255, 18, 179, 255, 18, 179, 255, 18, 179, 255, 18, 179, 255, 18, 179, 255, 18, 179, 255, 18, 179, 255, 18, 179, 255, 18, 179, 255, 18, 179, 255, 18, 179, 255, 18, 179, 255, 255, 255, 255, 255, 255, 255, 255, 255, 255, 18, 179, 255, 18, 179, 255, 18, 179, 255, 18, 179, 255, 18, 179, 255, 18, 179, 255, 18, 179, 255, 18, 179, 255, 18, 179, 255, 18, 179, 255, 18, 179, 255, 18, 179, 255, 18, 179, 255, 18, 179, 255, 18, 179, 255, 255, 255, 255, 255, 255, 255, 255, 255, 255, 18, 179, 255, 18, 179, 255, 18, 179, 255, 18, 179, 255, 18, 179, 255, 18, 179, 255, 18, 179, 255, 18, 179, 255, 18, 179, 255, 18, 179, 255, 18, 179, 255, 18, 179, 255, 18, 179, 255, 18, 179, 255, 18, 179, 255, 255, 255, 255, 255, 255, 255, 255, 255, 255, 18, 179, 255, 18, 179, 255, 18, 179, 255, 255, 255, 255, 18, 179, 255, 18, 179, 255, 18, 179, 255, 18, 179, 255, 18, 179, 255, 18, 179, 255, 18, 179, 255, 18, 179, 255, 18, 179, 255, 18, 179, 255, 18, 179, 255, 255, 255, 255, 255, 255, 255, 255, 255, 255, 18, 179, 255, 255, 255, 255, 255, 255, 255, 18, 179, 255, 18, 179, 255, 18, 179, 255, 18, 179, 255, 18, 179, 255, 18, 179, 255, 18, 179, 255, 18, 179, 255, 18, 179, 255, 18, 179, 255, 18, 179, 255, 18, 179, 255, 255, 255, 255, 255, 255, 255, 255, 255, 255, 255, 255, 255, 255, 255, 255, 255, 255, 255, 18, 179, 255, 18, 179, 255, 18, 179, 255, 18, 179, 255, 18, 179, 255, 18, 179, 255, 18, 179, 255, 18, 179, 255, 18, 179, 255, 18, 179, 255, 18, 179, 255, 18, 179, 255, 255, 255, 255, 255, 255, 255, 255, 255, 255, 255, 255, 255, 255, 255, 255, 18, 179, 255, 18, 179, 255, 18, 179, 255, 18, 179, 255, 18, 179, 255, 18, 179, 255, 18, 179, 255, 18, 179, 255, 18, 179, 255, 18, 179, 255, 18, 179, 255, 255, 255, 255, 255, 255, 255, 255, 255, 255, 255, 255, 255, 255, 255, 255, 255, 255, 255, 18, 179, 255, 18, 179, 255, 18, 179, 255, 18, 179, 255, 18, 179, 255, 18, 179, 255, 18, 179, 255, 18, 179, 255, 18, 179, 255, 18, 179, 255, 255, 255, 255, 255, 255, 255, 255, 255, 255, 255, 255, 255, 255, 255, 255, 255, 255, 255, 255, 255, 255, 255, 255, 255, 18, 179, 255, 18, 179, 255, 18, 179, 255, 18, 179, 255, 18, 179, 255, 18, 179, 255, 18, 179, 255, 18, 179, 255, 18, 179, 255, 18, 179, 255, 18, 179, 255, 255, 255, 255, 255, 255, 255, 255, 255, 255, 255, 255, 255, 255, 255, 255, 255, 255, 255, 18, 179, 255, 18, 179, 255, 18, 179, 255, 18, 179, 255, 18, 179, 255, 18, 179, 255, 18, 179, 255, 18, 179, 255, 18, 179, 255, 18, 179, 255, 18, 179, 255, 18, 179, 255, 18, 179, 255, 18, 179, 255, 255, 255, 255, 255, 255, 255, 255, 255, 255, 18, 179, 255, 18, 179, 255, 18, 179, 255, 18, 179, 255, 18, 179, 255, 18, 179, 255, 18, 179, 255, 18, 179, 255, 18, 179, 255, 18, 179, 255, 18, 179, 255, 18, 179, 255, 18, 179, 255, 18, 179, 255, 18, 179, 255, 18, 179, 255, 18, 179, 255, 18, 179, 255, 18, 179, 255, 18, 179, 255, 18, 179, 255, 18, 179, 255, 18, 179, 255, 18, 179, 255, 18, 179, 255, 18, 179, 255, 18, 179, 255, 18, 179, 255, 18, 179, 255, 18, 179, 255, 18, 179, 255, 18, 179, 255, 18, 179, 255, 18, 179, 255, 18, 179, 255, 18, 179, 255, 18, 179, 255, 18, 179, 255, 18, 179, 255, 18, 179, 255, 18, 179, 255, 18, 179, 255, 18, 179, 255, 18, 179, 255, 18, 179, 255, 18, 179, 255, 18, 179, 255, 18, 179, 255, 18, 179, 255, 18, 179, 255, 18, 179, 255, 18, 179, 255, 18, 179, 255, 18, 179, 255], "mask"=[], "colors"=[], "Rectangle"={"left"=0, "top"=0, "right"=17, "bottom"=17}}  # blue down arrow
        n163 = Build Array(w511, w510, w509, w508, w507, w506, w505, w504, w503, w502, w501, w500) -> ()  [unwired: 1 out]
      }
      frame "Init Y defs" {
        n164 = Unbundle By Name(w527) -> ("RegsParam"=w520:dbl[][], "Regs_Descriptions"=w519:string[][])
        n165 = vi-ref "Reg visu.lvclass:Run.vi"() -> (w524:refnum<vi>)
        n166 = property class="VI"(reference=w524) -> (reference out=w525:refnum<vi>, "Name"=w526:string)  [unwired: 1 in, 1 out]
        n167 = Close Reference(reference=w525) -> ()  [unwired: 1 in, 1 out]
        n168 = for {
          N: 1 -> [_]
          tunnel: refnum<class "Reg visu.lvclass"> refnum ("Reg visu.lvclass") -> [w537]
          tunnel: w521 -> [w566]
          tunnel: w518 -> [w555]
          tunnel: w526 -> [w564]
          tunnel: w520 -> [w557] mode=indexing
          tunnel: w519 -> [w546] mode=indexing
          tunnel: [w530] -> w517 mode=indexing
          i -> [w567]
          w533 = 128  # Enable simultaneous calls on reentrant VIs
          n169 = Index Array(array=w557) -> (element #1=w556:dbl, element #2=w554:dbl, element #3=w552:dbl, element #4=w550:dbl, element #5=w548:dbl)  [unwired: 5 in]
          n170 = call "Write Scale max.vi"("error in (no error)"=w555, "Scale max"=w556, "Reg visu in"=w537) -> ("error out"=w553:errorcluster, "Reg visu out"=w561:refnum<class "Reg visu.lvclass">)  [unwired: 7 in]
          n171 = call "Write auto.vi"("error in (no error)"=w553, "auto"=w554, "Reg visu in"=w561) -> ("error out"=w551:errorcluster, "Reg visu out"=w560:refnum<class "Reg visu.lvclass">)  [unwired: 7 in]
          n172 = call "Write alarm value.vi"("error in (no error)"=w551, "alarm value"=w552, "Reg visu in"=w560) -> ("error out"=w549:errorcluster, "Reg visu out"=w559:refnum<class "Reg visu.lvclass">)  [unwired: 7 in]
          n173 = call "Write k.vi"("error in (no error)"=w549, "k"=w550, "Reg visu in"=w559) -> ("error out"=w547:errorcluster, "Reg visu out"=w558:refnum<class "Reg visu.lvclass">)  [unwired: 7 in]
          n174 = call "Write t.vi"("error in (no error)"=w547, "t"=w548, "Reg visu in"=w558) -> ("error out"=w542:errorcluster, "Reg visu out"=w543:refnum<class "Reg visu.lvclass">)  [unwired: 7 in]
          n175 = Increment(x=w567) -> (x+1=w569:i32)
          n176 = Index Array(array=w546) -> (element #1=w545:string, element #3=w544:string)  [unwired: 3 in, 1 out]
          n177 = Number To Decimal String(number=w569) -> (decimal integer string=w568:string)  [unwired: 1 in]
          n178 = call "Write group.vi"("error in (no error)"=w542, "group"=w545, "Reg visu in"=w543) -> ("error out"=w541:errorcluster, "Reg visu out"=w540:refnum<class "Reg visu.lvclass">)  [unwired: 7 in]
          n179 = Concatenate Strings("GM1QN" ("string"), w568) -> (w563:string)
          n180 = call "Write gas.vi"("error in (no error)"=w541, "gas"=w544, "Reg visu in"=w540) -> ("error out"=w538:errorcluster, "Reg visu out"=w539:refnum<class "Reg visu.lvclass">)  [unwired: 7 in]
          n181 = call "Write object_name.vi"("error in (no error)"=w538, "object_name"=w563, "Reg visu in"=w539) -> ("error out"=w571:errorcluster, "Reg visu out"=w572:refnum<class "Reg visu.lvclass">)  [unwired: 7 in]
          n182 = call "Write N.vi"("error in (no error)"=w571, "N"=w567, "Reg visu in"=w572) -> ("error out"=w562:errorcluster, "Reg visu out"=w573:refnum<class "Reg visu.lvclass">)  [unwired: 7 in]
          n183 = Open VI Reference(type specifier VI Refnum (for type only)=refnum<vi> refnum, vi path=w564, options=w533, error in (no error)=w562) -> (vi reference=w535:refnum<vi>, error out=w536:errorcluster)  [unwired: 2 in]
          n184 = call-by-ref "Start Asynchronous Call"(reference=w535, error in=w536, "message queue in"=w566, "Reg visu in"=w573) -> (reference out=w534:refnum<vi>, error out=w532:errorcluster)  [unwired: 9 in, 1 out]
          n185 = invoke on="Sub Panel" class="SubPnl" method="Insert VI"(error in=w532, "VI Ref"=w534) -> (error out=w531:errorcluster)  [unwired: 2 in, 3 out]
          n186 = Close Reference(reference=w534, error in (no error)=w531) -> (error out=w530:errorcluster)
        }
        n187 = Merge Errors(w517) -> (w516:errorcluster)
      }
      frame "Exit".. {
      }
      frame Default {
        n188 = Increment(x=w583) -> (x+1=w582:T2)
      }
    }
    n189 = Or(x=w20, y=w26) -> (x .or. y?=w25:bool)
  }
  n190 = for {
    N: 23 -> [_]
    tunnel: [w589] -> w3 mode=indexing
    tunnel: [w586] -> w1 mode=indexing
    i -> [w592]
    n191 = Increment(x=w592) -> (x+1=w594:i32)
    n192 = Number To Decimal String(number=w594) -> (decimal integer string=w593:string)  [unwired: 1 in]
    n193 = Concatenate Strings("ns=2;s=", "GM1QN" ("string"), w593) -> (w588:string)
    n194 = Concatenate Strings(w588, ".control") -> (w586:string)
    n195 = Concatenate Strings(w588, ".state") -> (w589:string)
  }
  n196 = Unbundle By Name(w4) -> ("OPC UA.data change event"=w14:refnum<user-event>)
  n197 = register-events(w14) -> (reference out=w15:refnum<event-registration>)  [unwired: 2 in, 1 out]
  n198 = while "Message Processor" {
    shift-left: w6 -> [w607]
    shift-right: [w611] -> w8
    tunnel: w9 -> [w608]
    tunnel: w4 -> [w602]
    tunnel: [w601] -> w16
    tunnel: w3 -> [w599]
    tunnel: w1 -> [w598]
    shift-right: [w596] -> _
    shift-left: w5 -> [w597]
    stop <- w610 stop-if-true
    w603 = 100  # Timeout
    n199 = call <vilib>:"Read Next Message.vi"("message queue in"=w608, "timeout (1 ms)"=w603, "error in"=w607) -> ("exit process?"=w610:bool, "message queue out"=w609:T3, "message name"=w605:string, "message value"=w604:string, "message"=w600:T56, "error out"=w606:errorcluster)  [unwired: 5 in, 2 out]
    n200 = case shown="\"\", \"Idle\"" w605 {
      selector: w605 -> [_ _ w643 _ _ _ _ _ _ _ _ _ _ _ _]
      tunnel: w609 -> [_ _ _ w650 _ _ w657 _ _ w682 w703 _ w750 _ _]
      tunnel: w606 -> [w613 w626 w644 w648 w652 w654 w658 w660 w666 w681 w711 w724 w734 w774 w805]
      tunnel: [w613 w617 w644 w646 w652 w654 w656 w660 w666 w686 w704 w726 w751 w776 w813] -> w611
      tunnel: w604 -> [_ _ _ _ _ _ _ _ w665 _ _ _ _ w773 w792]
      tunnel: w602 -> [_ w622 _ _ _ _ _ _ _ w675 w712 w725 w736 w775 w812]
      tunnel: w600 -> [_ _ _ _ _ _ _ _ _ _ _ _ _ w772 _]
      tunnel: w599 -> [_ w615 _ _ _ _ _ _ _ _ _ _ _ _ _]
      tunnel: w598 -> [_ _ _ _ _ _ _ _ _ _ w709 w722 _ _ _]
      tunnel: w597 -> [w612 w614 w640 w645 w651 w653 w655 w659 w661 w685 w702 w719 w733 w761 w801]
      tunnel: [w612 w614 w640 w645 w651 w653 w655 w659 w661 w685 w702 w719 w733 w761 w801] -> w596
      frame "---------- Framework Operations ----------" {
        # "Dummy case to add a seperator in the Case Structure menu"
      }
      frame "", "Idle" {
        n201 = Unbundle By Name(w622) -> ("OPC UA.Client refnum"=w619:T17)
        n202 = Unbundle By Name(w622) -> ("system DB"=w621:T15, "Enums.AI"=w620:string[])
        n203 = call-poly <vilib>:"Multiple Read.vi"("error in (no error)"=w626, "node IDs"=w615, "OPC UA client refnum in"=w619) -> ("error out"=w624:errorcluster, "results"=w623:T58, "service status"=w625:T39)  [unwired: 5 in, 1 out]
        n204 = case shown="0..15" w625 {
          tunnel: w624 -> [w627 w633]
          tunnel: [w627 w632] -> w618
          tunnel: w623 -> [_ w631]
          tunnel: [_ w630] -> w616
          tunnel: [_ TRUE] -> _
          frame 16.., Default {
          }
          frame 0..15 {
            n205 = for {
              N: 23 -> [_]
              tunnel: w631 -> [w635] mode=indexing
              tunnel: [w636] -> w630 mode=indexing
              shift-right: [w637] -> w632
              shift-left: w633 -> [w638]
              n206 = Unbundle By Name(w635) -> ("value"=w639:string)
              n207 = call "From JSON Text.vim"("Data Type and Default Value"=T12 {"connect"=FALSE, "gas"="H2", "Y_State"={"Y_Source"=3, "Y_SetState"=0, "SP_Set"=0.0, "SP"=0.0, "PV"=0.0, "PV_State"={"code"=0, "visible"=FALSE, "color"=0}, "Y_preSet"=0.0, "Y_Set"=0.0, "Y"=0.0, "Y_State"={"code"=0, "visible"=FALSE, "color"=0}, "YB"=FALSE}} ("Y_short_conn"), "error in (no error)"=w638, "JSON"=w639) -> ("error out"=w637:errorcluster, "Data out"=w636:T12)  [unwired: 7 in]
            }
          }
        }
        n208 = call "View one AI param scada.vi"("OPC UA.Client refnum"=w619, "conninfo"=w621, "AIParameters"=w620) -> ()  [unwired: 8 in, 1 out]
        n209 = shared-variable ".\\Var scada.lvlib\\QN_states_short"(w616, error in=w618) -> (error out=w617:errorcluster)
      }
      frame "Missing Message Handler", Default {
        # "Call this case if a message is received that is not handled \nby any other case. Typically this is a programming error\nas a result of a typo or unhandled message/missing message handler."
        n210 = Format Into String(format string="DevError: Missing message handler for '%s\" message." ("message"), w643) -> (resulting string=w641:string)  [unwired: 2 in, 1 out]
        n211 = One Button Dialog(message=w641) -> ()  [unwired: 2 out]
      }
      frame "Error" {
        # "Proceed to Exit - Remove this if it is\nnot appropriate for the General Error case"
        # "General Error Case - this case is called if an error is passed using the error cluster below. Typically most new errors should be handed in each individual case and not passed in the rror cluster. If necessary a custom error handler case should be added and called from other cases."
        n212 = call <vilib>:"Simple Error Handler.vi"("error in (no error)"=w648) -> ()  [unwired: 1 in, 8 out]
        n213 = call <vilib>:"Clear Errors.vi"("error in (no error)"=w648) -> ("error out"=w647:errorcluster)  [unwired: 5 in, 1 out]
        n214 = call <vilib>:"Send Local Message.vi"("message queue in"=w650, "message name"="Exit", "error in"=w647) -> ("error out"=w646:errorcluster)  [unwired: 10 in, 2 out]
      }
      frame "---------- Generic Operations ----------" {
        # "Dummy case to add a seperator in the Case Structure menu"
      }
      frame "Initialize" {
        # "Initialize the state variables and user interface"
      }
      frame "Exit" {
        # "Destroy message queue >> this will halt the UI event handler loop"
        # "Stop the VI\n>> Perform any cleanup tasks in this message case.\n>> Clear display before closing."
        n215 = call <vilib>:"Destroy Message Queue.vi"("message queue in"=w657, "error in"=w658) -> ("error out"=w656:errorcluster)  [unwired: 11 in, 2 out]
      }
      frame "---------- Application Operations ----------" {
        # "Dummy case to add a seperator in the Case Structure menu"
      }
      frame "Process Data" {
        # "Add actions to perform in response to Process button being pressed"
        n216 = Fract/Exp String To Number(string=w665) -> (number=w664:dbl)  [unwired: 4 out]
        n217 = Format Into String(format string="Process Data: %f" ("message"), w664) -> (resulting string=w662:string)  [unwired: 2 in, 1 out]
        n218 = One Button Dialog(message=w662) -> ()  [unwired: 2 out]
      }
      frame "Send auto param" {
        n219 = Unbundle By Name(w685) -> ("RegsParam"=w684:dbl[][])
        n220 = for {
          N: 23 -> [_]
          tunnel: w684 -> [w694] mode=indexing
          shift-right: [w689] -> w670
          shift-left: "UPDATE TMP_PAR SET {" ("string") -> [w690]
          i -> [w691]
          n221 = Increment(x=w691) -> (x+1=w700:i32)
          n222 = Index Array(array=w694, index=1) -> (element=w693:dbl)
          n223 = Number To Decimal String(number=w700) -> (decimal integer string=w699:string)  [unwired: 1 in]
          n224 = Number To Fractional String(use system decimal point (T)=FALSE, number=w693) -> (F-format string=w692:string)  [unwired: 2 in]
          n225 = Concatenate Strings(w690, "\"GM1QN" ("string"), w699, "_auto_value\":{\"value\":" ("string"), w692, "}," ("string")) -> (w689:string)
        }
        n226 = Unbundle By Name(w675) -> ("OPC UA.Client refnum"=w674:T17)
        n227 = String Length(string=w670) -> (length=w673:i32)
        n228 = Decrement(x=w673) -> (x-1=w671:i32)
        n229 = Replace Substring(2:1 ("length (len. of substring)"), 3:w671, 4:"}" ("string"), 5:w670) -> (1:w667:string)  [unwired: 1 out]
        n230 = Get Date/Time In Seconds() -> (seconds since 1Jan1904=w678:timestamp)
        n231 = call "Write element_1.vi"("seconds since 1Jan1904"=w678, "Variant"=w667, "node ID"=T7 "ns=2;s=CONTROL.control") -> ("request out"=w677:T19)  [unwired: 8 in]
        n232 = Build Array(w677) -> (w679:T19[])
        n233 = call-poly <vilib>:"Multiple Write.vi"("error in (no error)"=w681, "requests"=w679, "OPC UA client refnum in"=w674) -> ("error out"=w680:errorcluster)  [unwired: 5 in, 3 out]
        n234 = call <vilib>:"Send Local Message.vi"("message queue in"=w682, "message name"="Send Start On", "error in"=w680) -> ("error out"=w686:errorcluster)  [unwired: 10 in, 2 out]
        n235 = Wait (ms)(milliseconds to wait=u32 200) -> ()  [unwired: 1 out]
      }
      frame "Send Start On" {
        n236 = Get Date/Time In Seconds() -> (seconds since 1Jan1904=w714:timestamp)
        n237 = Unbundle By Name(w712) -> ("OPC UA.Client refnum"=w713:T17)
        n238 = for {
          tunnel: w714 -> [w718]
          tunnel: [w717] -> w708 mode=indexing
          tunnel: "{\"Start\":true}" -> [w716]
          tunnel: w709 -> [w715] mode=indexing
          n239 = call "Write element_1.vi"("seconds since 1Jan1904"=w718, "Variant"=w716, "node ID"=w715) -> ("request out"=w717:T19)  [unwired: 8 in]
        }
        n240 = call-poly <vilib>:"Multiple Write.vi"("error in (no error)"=w711, "requests"=w708, "OPC UA client refnum in"=w713) -> ("error out"=w705:errorcluster)  [unwired: 5 in, 3 out]
        n241 = call <vilib>:"Send Local Message.vi"("message queue in"=w703, "message name"="Send Start Off", "error in"=w705) -> ("error out"=w704:errorcluster)  [unwired: 10 in, 2 out]
        n242 = Wait (ms)(milliseconds to wait=u32 200) -> ()  [unwired: 1 out]
      }
      frame "Send Start Off" {
        n243 = Get Date/Time In Seconds() -> (seconds since 1Jan1904=w728:timestamp)
        n244 = Unbundle By Name(w725) -> ("OPC UA.Client refnum"=w727:T17)
        n245 = for {
          tunnel: w728 -> [w732]
          tunnel: [w731] -> w721 mode=indexing
          tunnel: "{\"Start\":false}" -> [w730]
          tunnel: w722 -> [w729] mode=indexing
          n246 = call "Write element_1.vi"("seconds since 1Jan1904"=w732, "Variant"=w730, "node ID"=w729) -> ("request out"=w731:T19)  [unwired: 8 in]
        }
        n247 = call-poly <vilib>:"Multiple Write.vi"("error in (no error)"=w724, "requests"=w721, "OPC UA client refnum in"=w727) -> ("error out"=w726:errorcluster)  [unwired: 5 in, 3 out]
        n248 = Wait (ms)(milliseconds to wait=u32 100) -> ()  [unwired: 1 out]
      }
      frame "Send Reset" {
        n249 = for {
          N: 23 -> [_]
          shift-right: [w755] -> w740
          shift-left: "UPDATE TMP_PAR SET {" ("string") -> [w756]
          i -> [w754]
          n250 = Increment(x=w754) -> (x+1=w759:i32)
          n251 = Number To Decimal String(number=w759) -> (decimal integer string=w758:string)  [unwired: 1 in]
          n252 = Concatenate Strings(w756, "\"GM1QN" ("string"), w758, "_auto_value\":{\"value\":0}," ("string")) -> (w755:string)
        }
        n253 = Unbundle By Name(w736) -> ("OPC UA.Client refnum"=w744:T17)
        n254 = String Length(string=w740) -> (length=w743:i32)
        n255 = Decrement(x=w743) -> (x-1=w741:i32)
        n256 = Replace Substring(2:1 ("length (len. of substring)"), 3:w741, 4:"}" ("string"), 5:w740) -> (1:w737:string)  [unwired: 1 out]
        n257 = Get Date/Time In Seconds() -> (seconds since 1Jan1904=w747:timestamp)
        n258 = call "Write element_1.vi"("seconds since 1Jan1904"=w747, "Variant"=w737, "node ID"=T7 "ns=2;s=CONTROL.control") -> ("request out"=w746:T19)  [unwired: 8 in]
        n259 = Build Array(w746) -> (w748:T19[])
        n260 = call-poly <vilib>:"Multiple Write.vi"("error in (no error)"=w734, "requests"=w748, "OPC UA client refnum in"=w744) -> ("error out"=w735:errorcluster)  [unwired: 5 in, 3 out]
        n261 = call <vilib>:"Send Local Message.vi"("message queue in"=w750, "message name"="Send Start On", "error in"=w735) -> ("error out"=w751:errorcluster)  [unwired: 10 in, 2 out]
        n262 = Wait (ms)(milliseconds to wait=u32 200) -> ()  [unwired: 1 out]
      }
      frame "Send Y Control" {
        n263 = Unbundle By Name(w772) -> ("attributes.keys"=w770:string[], "attributes.values"=w769:string[])
        n264 = for {
          shift-right: [w784] -> w768
          shift-left: "{" -> [w789]
          tunnel: w770 -> [w787] mode=indexing
          tunnel: w769 -> [w786] mode=indexing
          n265 = Concatenate Strings(w789, "\"", w787, "\":", w786, ",") -> (w784:string)
        }
        n266 = String Length(string=w768) -> (length=w767:i32)
        n267 = Decrement(x=w767) -> (x-1=w766:i32)
        n268 = Replace Substring(2:1 ("length (len. of substring)"), 3:w766, 4:"}", 5:w768) -> (1:w763:string)  [unwired: 1 out]
        n269 = Unbundle By Name(w775) -> ("OPC UA.Client refnum"=w778:T17)
        n270 = Concatenate Strings("ns=2;s=", w773, ".control") -> (w777:string)
        n271 = Get Date/Time In Seconds() -> (seconds since 1Jan1904=w783:timestamp)
        n272 = call "Write element_1.vi"("seconds since 1Jan1904"=w783, "Variant"=w763, "node ID"=w777) -> ("request out"=w782:T19)  [unwired: 8 in]
        n273 = Build Array(w782) -> (w781:T19[])
        n274 = call-poly <vilib>:"Multiple Write.vi"("error in (no error)"=w774, "requests"=w781, "OPC UA client refnum in"=w778) -> ("error out"=w776:errorcluster)  [unwired: 5 in, 3 out]
        n275 = Wait (ms)(milliseconds to wait=u32 200) -> ()  [unwired: 1 out]
      }
      frame "Send Control" {
        w809 = 4  # fcode_full
        n276 = Unbundle By Name(w801) -> ("Regs_Descriptions"=w802:string[][])
        n277 = Scan From String(format string="%s%s SET %[^]", input string=w792) -> (error out=w793:errorcluster, output 1=w799:string, output 2=w798:string, output 3=w797:string)  [unwired: 5 in, 2 out]
        n278 = call "Is Value Changed.vim"("value"=w792) -> ("changed or first call?"=w795:bool)
        n279 = Not(x=w793) -> (.not. x?=w796:bool)
        n280 = And(x=w796, y=w795) -> (x .and. y?=w794:bool)
        n281 = case shown="False" w794 {
          tunnel: w799 -> [_ w825]
          tunnel: [w819 w822] -> _
          tunnel: w798 -> [_ w824]
          tunnel: w797 -> [_ w823]
          tunnel: w793 -> [w818 w821]
          tunnel: [_ w820] -> w791
          frame False {
            n282 = call <vilib>:"Clear Errors.vi"("error in (no error)"=w818) -> ("error out"=w819:errorcluster)  [unwired: 5 in, 1 out]
          }
          frame True {
            n283 = case shown="Default" w825 {
              tunnel: w824 -> [_ w830]
              tunnel: w823 -> [_ w829]
              tunnel: w821 -> [w826 w831]
              tunnel: [w826 w828] -> w822
              tunnel: [_ w827] -> w820
              frame Default {
              }
              frame "UPDATE" {
                n284 = case shown="Default" w830 {
                  tunnel: w829 -> [w832 w835 w837]
                  tunnel: [w833 w834 w836] -> w828
                  tunnel: w831 -> [w833 w834 w836]
                  tunnel: [w832 w835 w837] -> w827
                  frame Default {
                  }
                  frame "PAR" {
                  }
                  frame "TMP_PAR" {
                  }
                }
              }
            }
          }
        }
        n285 = Index Array(array=w802, index (col)=w809) -> (element=w808:string[])  [unwired: 1 in]
        n286 = call "JSON to array.vi"("error in (no error)"=w805, "JSON Data In"=w791) -> ("error out"=w806:errorcluster, "values"=w804:string[], "names"=w807:string[][])  [unwired: 7 in]
        n287 = for {
          tunnel: w808 -> [w851]
          tunnel: w804 -> [w846] mode=indexing
          shift-right: [w847] -> _
          shift-left: w806 -> [w843]
          shift-right: [w852] -> _
          shift-left: dbl[][] [] -> [w853]
          tunnel: w807 -> [w841] mode=indexing
          w850 = ParamColumns."value"  # ParamColumns
          n288 = Index Array(array=w841) -> (element #1=w840:string, element #2=w839:string)  [unwired: 2 in]
          n289 = Fract/Exp String To Number(use system decimal point (T)=FALSE, string=w846, default (0 dbl)=nan ("default (0 DBL)")) -> (number=w845:dbl)  [unwired: 1 in, 1 out]
          n290 = Search 1D Array(1D array=w851, element=w840) -> (index of element=w849:i32)  [unwired: 1 in]
          n291 = Scan From String(input string=w839, error in=w843, default 1=w850) -> (error out=w842:errorcluster, output 1=w848:T59)  [unwired: 2 in, 2 out]
          n292 = case shown="No Error" w842 {
            selector: w842 -> [w854 w867]
            tunnel: w853 -> [w859 w868]
            tunnel: [w858 w868] -> w852
            tunnel: w848 -> [w857 _]
            tunnel: w845 -> [w856 _]
            tunnel: w849 -> [w855 _]
            tunnel: [w854 w867] -> w847
            frame No Error {
              n293 = case shown="0, Default" w855 {
                selector: w855 -> [w860 _]
                tunnel: w859 -> [w864 w866]
                tunnel: [w863 w866] -> w858
                tunnel: w857 -> [w862 _]
                tunnel: w856 -> [w861 _]
                frame 0, Default {
                  n294 = in-place {
                    in-place-border: w861 -> [w865]
                    n295 = in-place-array #1(w864, w860, w862) -> ()  [unwired: 1 out]
                    n296 = in-place-array #1(w865) -> (w863:dbl[][])  [unwired: 2 out]
                  }
                }
                frame -1 {
                }
              }
            }
            frame Error {
            }
          }
        }
        n297 = Unbundle By Name(w812) -> ("OPC UA.Client refnum"=w814:T17)
        n298 = Get Date/Time In Seconds() -> (seconds since 1Jan1904=w817:timestamp)
        n299 = call "Write element_1.vi"("seconds since 1Jan1904"=w817, "Variant"=w792, "node ID"=T7 "ns=2;s=CONTROL.control") -> ("request out"=w816:T19)  [unwired: 8 in]
        n300 = Build Array(w816) -> (w815:T19[])
        n301 = call-poly <vilib>:"Multiple Write.vi"("error in (no error)"=w805, "requests"=w815, "OPC UA client refnum in"=w814) -> ("error out"=w813:errorcluster)  [unwired: 5 in, 3 out]
        n302 = Wait (ms)(milliseconds to wait=u32 200) -> ()  [unwired: 1 out]
      }
    }
    n303 = control-ref of="This VI"() -> (w601:refnum<vi>)
  }
  n304 = while "Message Generator - User Interface Event Handler" {
    tunnel: w9 -> [w872]
    tunnel: w15 -> [w871]
    tunnel: [w870] -> w13
    tunnel: [w869] -> w7
    stop <- w873 stop-if-true
    w874 = 100  # Event Structure Timeout (ms)
    n305 = event shown="[8] \"HT1 emergency stop\": Value Change" {
      selector: w871 -> [_ _ _ _ _ _ _ _ _]
      dyn-events: [_ _ _ _ _ _ _ _ _] -> w870
      timeout: w874 -> [_ _ _ _ _ _ _ _ _]
      tunnel: [w879 _ w888 w889 _ _ _ _ _] -> w873
      tunnel: w872 -> [w878 _ w886 w892 w896 w907 w909 w911 w913]
      tunnel: [_ _ _ w891 _ _ _ _ _] -> w869
      event Timeout {
        # "Exit UI event handler loop if message queue\nis destroyed in the message processor"
        n306 = event-data() -> ()  [unwired: 2 out]
        n307 = global read "Global stop.vi" "Stop"() -> (w875:bool)
        n308 = case shown="False" w875 {
          tunnel: w878 -> [w881 w884]
          tunnel: [_ w883] -> w876
          tunnel: [w881 w882] -> w877
          frame False {
          }
          frame True {
            n309 = call <vilib>:"Send Local Message.vi"("message queue in"=w884, "message name"="Exit") -> ("message queue out"=w882:T3, "error out"=w883:errorcluster)  [unwired: 11 in, 1 out]
          }
        }
        n310 = call <vilib>:"Check Message Queue Status.vi"("message queue in"=w877, "error in"=w876) -> ("error out"=w880:errorcluster)  [unwired: 9 in, 4 out]
        n311 = Unbundle By Name(w880) -> ("status"=w879:bool)
        n312 = local write "Останов\nпрограммы"(w879) -> ()
      }
      event User Event {
        n313 = event-data() -> ()  [unwired: 7 out]
      }
      event Panel Close? {
        w888 = TRUE ("Discard?")
        # "Intercepts the upper right close panel\noperation to allow a smooth shutdown\nas opposed to immediately killing the app."
        n314 = event-data() -> ()  [unwired: 2 out]
        n315 = call <vilib>:"Send Local Message.vi"("message queue in"=w886, "message name"="Exit") -> ()  [unwired: 11 in, 3 out]
        n316 = event-data("Discard?"=w888) -> ()  [unwired: 1 in, 1 out]
      }
      event "Останов\nпрограммы": Value Change {
        # "Exit the application\n>> Stop this message generator loop"
        n317 = event-data() -> ()  [unwired: 5 out]
        n318 = Two Button Dialog(message="Остановить программу?\nРасходы останутся") -> (T button?=w889:bool)  [unwired: 2 in]
        n319 = case shown="True" w889 {
          tunnel: w892 -> [_ w894]
          tunnel: [_ w893] -> w891
          frame False {
          }
          frame True {
            n320 = call <vilib>:"Send Local Message.vi"("message queue in"=w894, "message name"="Exit") -> ("error out"=w893:errorcluster)  [unwired: 11 in, 2 out]
          }
        }
      }
      event Menu Selection (User) {
        # "Add run-time menu items to the message\nqueue. The message handler case names must match the menu ItemTag names."
        n321 = event-data() -> ("ItemTag"=w897:string)  [unwired: 1 out]
        n322 = call <vilib>:"Send Local Message.vi"("message queue in"=w896, "message name"=w897) -> ()  [unwired: 11 in, 3 out]
      }
      event "process": Value Change {
        n323 = event-data() -> ()  [unwired: 2 out]
        n324 = Random Number (0-1)() -> (number: 0 to 1=w904:dbl)
        n325 = Number To Fractional String(number=w904) -> (F-format string=w905:string)  [unwired: 3 out]
        n326 = call <vilib>:"Send Local Message.vi"("message queue in"=w907, "message name"="Process Data", "message value"=w905) -> ("message queue out"=w903:T3, "error out"=w899:errorcluster)  [unwired: 10 in, 1 out]
        n327 = call <vilib>:"Send Network Message.vi"("message queue in"=w903, "receiver process"="Control", "receiver host"="192.168.0.70", "receiver port (0)"=u16 9000, "message name"="message name", "error in"=w899) -> ()  [unwired: 7 in, 3 out]
      }
      event "Start": Value Change {
        n328 = event-data() -> ()  [unwired: 7 out]
        n329 = call <vilib>:"Send Local Message.vi"("message queue in"=w909, "message name"="Send auto param") -> ()  [unwired: 11 in, 3 out]
      }
      event "Reset": Value Change {
        n330 = event-data() -> ()  [unwired: 7 out]
        n331 = call <vilib>:"Send Local Message.vi"("message queue in"=w911, "message name"="Send Reset") -> ()  [unwired: 11 in, 3 out]
      }
      event "HT1 emergency stop": Value Change {
        n332 = event-data() -> ()  [unwired: 7 out]
        n333 = call <vilib>:"Send Local Message.vi"("message queue in"=w913, "message name"="Send Reset") -> ()  [unwired: 11 in, 3 out]
      }
    }
  }
  n334 = disable-structure shown="Disabled" {
    disable-tunnel: w6 -> [w916 _]
    disable-tunnel: w5 -> [w915 _]
    disable-tunnel: w4 -> [w914 _]
    frame Disabled {
      n335 = while {
        shift-right: [w926] -> _
        shift-left: scada_prog_state."ReadAIParam" ("Enum") -> [w927]
        tunnel: w914 -> [w920]
        shift-right: [w922] -> _
        shift-left: w915 -> [w921]
        shift-right: [w925] -> _
        shift-left: w916 -> [w924]
        tunnel: [w918] -> _
        stop <- w923 stop-if-true
        n336 = case shown="\"Exit\"" w927 {
          tunnel: [scada_prog_state."ReadDIParam" ("Enum") scada_prog_state."AI" ("Enum") scada_prog_state."AIValues" ("Enum") scada_prog_state."Alarms" ("Enum") scada_prog_state."TB1" ("Enum") scada_prog_state."TB2" ("Enum") scada_prog_state."TB3" ("Enum") scada_prog_state."Exit" ("Enum") scada_prog_state."AI" ("Enum")] -> w926
          tunnel: [w929 w967 w1006 w1135 w1211 w1313 w1386 w1460 w1519] -> w925
          tunnel: w924 -> [w928 w968 w1005 w1134 w1208 w1318 w1392 w1466 w1519]
          tunnel: [_ _ _ _ _ _ _ _ w1518] -> w923
          tunnel: [w932 w965 w1004 w1137 w1210 w1296 w1389 w1463 w1517] -> w922
          tunnel: w921 -> [w931 w966 w1003 w1137 w1210 w1315 w1388 w1465 w1517]
          tunnel: w920 -> [w930 w969 w1002 w1136 w1207 w1319 w1393 w1467 w1515]
          tunnel: [_ _ _ _ _ _ _ _ "tick"] -> w919
          tunnel: [w930 w969 w1002 w1136 w1207 w1319 w1393 w1467 w1515] -> w918
          frame "ReadAIParam", Default {
            n337 = disable-structure shown="SERVER==OPC" {
              disable-tunnel: [w938 w948] -> w933
              disable-tunnel: w930 -> [w941 w956]
              disable-tunnel: w928 -> [w939 w951]
              disable-tunnel: [w935 w950] -> w929
              frame condition #0 {
                n338 = Unbundle By Name(w941) -> ("Enums.AI"=w937:string[], "AI_Names_SHVR"=w940:refnum<k21>)
                n339 = shared-variable-read(w940, w939) -> (w935:errorcluster, w936:string[])  [unwired: 2 out]
                n340 = case shown="No Error" w935 {
                  tunnel: w936 -> [_ w942]
                  tunnel: w937 -> [_ w944]
                  tunnel: [_ w943] -> w938
                  frame Error {
                  }
                  frame No Error {
                    n341 = for {
                      tunnel: w944 -> [w947] mode=indexing
                      tunnel: w942 -> [w946]
                      tunnel: [w945] -> w943 mode=indexing
                      n342 = Search 1D Array(1D array=w946, element=w947) -> (index of element=w945:i32)  [unwired: 1 in]
                    }
                  }
                }
              }
              frame condition #1 (active) {
                n343 = Unbundle By Name(w956) -> ("Enums.AI"=w949:string[], "OPC UA.Client refnum"=w953:T17)
                n344 = call-poly <vilib>:"Multiple Read.vi"("error in (no error)"=w951, "node IDs"=T6 ["ns=2;s=AI.AI_Names"] ("OPC UA.node IDs"), "OPC UA client refnum in"=w953) -> ("error out"=w950:errorcluster, "results"=w955:T40, "service status"=w954:T39)  [unwired: 5 in, 1 out]
                n345 = case shown="0..15" w954 {
                  tunnel: w955 -> [_ w960]
                  tunnel: w949 -> [_ w958]
                  tunnel: [_ w957] -> w948
                  frame 16.., Default {
                  }
                  frame 0..15 {
                    n346 = Index Array(array=w960) -> (element=w961:T41)  [unwired: 1 in]
                    n347 = Unbundle By Name(w961) -> ("values"=w959:string[])
                    n348 = for {
                      tunnel: w958 -> [w964] mode=indexing
                      tunnel: w959 -> [w963]
                      tunnel: [w962] -> w957 mode=indexing
                      n349 = Search 1D Array(1D array=w963, element=w964) -> (index of element=w962:i32)  [unwired: 1 in]
                    }
                  }
                }
              }
            }
            n350 = Bundle By Name(cluster=w931, "AI_reorder_table"=w933) -> (w932:T22)
          }
          frame "ReadDIParam" {
            n351 = disable-structure shown="SERVER==OPC" {
              disable-tunnel: [w975 w985] -> w970
              disable-tunnel: w969 -> [w978 w993]
              disable-tunnel: w968 -> [w976 w988]
              disable-tunnel: [w972 w987] -> w967
              frame condition #0 {
                n352 = Unbundle By Name(w978) -> ("Enums.DI"=w974:string[], "DI_Names_SHVR"=w977:refnum<k21>)
                n353 = shared-variable-read(w977, w976) -> (w972:errorcluster, w973:string[])  [unwired: 2 out]
                n354 = case shown="No Error" w972 {
                  tunnel: w973 -> [_ w979]
                  tunnel: w974 -> [_ w981]
                  tunnel: [_ w980] -> w975
                  frame Error {
                  }
                  frame No Error {
                    n355 = for {
                      tunnel: w981 -> [w984] mode=indexing
                      tunnel: w979 -> [w983]
                      tunnel: [w982] -> w980 mode=indexing
                      n356 = Search 1D Array(1D array=w983, element=w984) -> (index of element=w982:i32)  [unwired: 1 in]
                    }
                  }
                }
              }
              frame condition #1 (active) {
                n357 = Unbundle By Name(w993) -> ("Enums.DI"=w986:string[], "OPC UA.Client refnum"=w990:T17)
                n358 = call-poly <vilib>:"Multiple Read.vi"("error in (no error)"=w988, "node IDs"=T6 ["ns=2;s=DI.DI_Names"] ("OPC UA.node IDs"), "OPC UA client refnum in"=w990) -> ("error out"=w987:errorcluster, "results"=w992:T40, "service status"=w991:T39)  [unwired: 5 in, 1 out]
                n359 = case shown="0..15" w991 {
                  tunnel: w992 -> [_ w997]
                  tunnel: w986 -> [_ w995]
                  tunnel: [_ w994] -> w985
                  frame 16.., Default {
                  }
                  frame 0..15 {
                    n360 = Index Array(array=w997) -> (element=w998:T41)  [unwired: 1 in]
                    n361 = Unbundle By Name(w998) -> ("values"=w996:string[])
                    n362 = for {
                      tunnel: w995 -> [w1001] mode=indexing
                      tunnel: w996 -> [w1000]
                      tunnel: [w999] -> w994 mode=indexing
                      n363 = Search 1D Array(1D array=w1000, element=w1001) -> (index of element=w999:i32)  [unwired: 1 in]
                    }
                  }
                }
              }
            }
            n364 = Bundle By Name(cluster=w966, "DI_reorder_table"=w970) -> (w965:T22)
          }
          frame "AI" {
            # "ReadParam"
            n365 = in-place {
              in-place-border: w1002 -> [w1014]
              in-place-border: [w1013] -> w1006
              in-place-border: w1005 -> [w1012]
              in-place-border: w1003 -> [w1011]
              n366 = in-place-cluster #2(w1003) -> ()  [unwired: 3 out]
              n367 = disable-structure shown="SERVER==SHRV, Default" {
                disable-tunnel: w1011 -> [w1020 w1087]
                disable-tunnel: w1014 -> [w1031 w1086]
                disable-tunnel: [w1018 w1079] -> w1013
                disable-tunnel: w1012 -> [w1030 w1084]
                disable-tunnel: [w1017 w1078] -> w1010
                disable-tunnel: [w1016 w1077] -> w1009
                disable-tunnel: [w1015 w1076] -> w1008
                frame condition #0 (active) {
                  n368 = Unbundle By Name(w1031) -> ("OPC UA.Client refnum"=w1033:T17)
                  n369 = Unbundle By Name(w1020) -> ("AI_reorder_table"=w1019:i32[])
                  n370 = call-poly <vilib>:"Multiple Read.vi"("error in (no error)"=w1030, "node IDs"=T6 ["ns=2;s=AI.AI"] ("OPC UA.node IDs"), "OPC UA client refnum in"=w1033) -> ("error out"=w1028:errorcluster, "results"=w1034:T65, "OPC UA client refnum out"=w1029:T17, "service status"=w1026:T39)  [unwired: 5 in]
                  n371 = call-poly <vilib>:"Multiple Read.vi"("error in (no error)"=w1028, "node IDs"=T6 ["ns=2;s=AI.AI_State", "ns=2;s=AI.AI_ALRState"] ("OPC UA.node IDs"), "OPC UA client refnum in"=w1029) -> ("error out"=w1018:errorcluster, "results"=w1021:T66, "service status"=w1025:T39)  [unwired: 5 in, 1 out]
                  n372 = case shown="0..15" w1025 {
                    tunnel: [_ TRUE] -> w1024
                    frame 16.., Default {
                    }
                    frame 0..15 {
                    }
                  }
                  n373 = case shown="0..15" w1026 {
                    tunnel: [_ TRUE] -> w1023
                    frame 16.., Default {
                    }
                    frame 0..15 {
                    }
                  }
                  n374 = And(x=w1024, y=w1023) -> (x .and. y?=w1022:bool)
                  n375 = case shown="True" w1022 {
                    tunnel: w1034 -> [w1047 _]
                    tunnel: w1021 -> [w1046 _]
                    tunnel: w1019 -> [w1041 w1071]
                    tunnel: [w1039 w1070] -> w1017
                    tunnel: [w1038 w1069] -> w1016
                    tunnel: [w1037 w1068] -> w1015
                    frame True {
                      n376 = Index Array(array=w1047) -> (element=w1048:T67)  [unwired: 1 in]
                      n377 = Index Array(array=w1046) -> (element #1=w1045:T68, element #2=w1043:T68)  [unwired: 2 in]
                      n378 = Unbundle By Name(w1048) -> ("values"=w1044:dbl[])
                      n379 = Unbundle By Name(w1045) -> ("values"=w1042:i32[])
                      n380 = Unbundle By Name(w1043) -> ("values"=w1040:i32[])
                      n381 = for {
                        tunnel: w1044 -> [w1055]
                        tunnel: w1041 -> [w1051] mode=indexing
                        tunnel: [w1054] -> w1039 mode=indexing
                        tunnel: w1040 -> [w1053]
                        tunnel: [w1052] -> w1038 mode=indexing
                        tunnel: w1042 -> [w1050]
                        tunnel: [w1049] -> w1037 mode=indexing
                        n382 = case shown="0, Default" w1051 {
                          selector: w1051 -> [_ w1059]
                          tunnel: w1055 -> [_ w1067]
                          tunnel: [nan ("PV") w1066] -> w1054
                          tunnel: w1053 -> [_ w1065]
                          tunnel: [T5 {"code"=0, "visible"=FALSE, "color"=14803425, "source"="отсутствует запись или ошибка в базе данных "} ("STATE") w1061] -> w1052
                          tunnel: w1050 -> [_ w1064]
                          tunnel: [errorcluster {"status"=TRUE, "code"=10, "source"="отсутствует запись или ошибка в базе данных "} ("ALRSTATE") w1060] -> w1049
                          frame -1 {
                          }
                          frame 0, Default {
                            n383 = Index Array(array=w1067, index=w1059) -> (element=w1066:dbl)
                            n384 = Index Array(array=w1064, index=w1059) -> (element=w1063:i32)
                            n385 = Index Array(array=w1065, index=w1059) -> (element=w1062:i32)
                            n386 = call "Sensor handling scada.vi"("AI_ALRState"=w1062, "AI_State"=w1063) -> ("ALRSTATE"=w1060:errorcluster, "STATE"=w1061:T5)  [unwired: 8 in]
                          }
                        }
                      }
                    }
                    frame False {
                      n387 = Array Size(array=w1071) -> (size(s)=w1072:i32)
                      n388 = for {
                        N: w1072 -> [_]
                        tunnel: [nan ("PV")] -> w1070 mode=indexing
                        tunnel: [T5 {"code"=0, "visible"=FALSE, "color"=14803425, "source"="отсутствует запись или ошибка в базе данных "} ("STATE")] -> w1069 mode=indexing
                        tunnel: [errorcluster {"status"=TRUE, "code"=10, "source"="отсутствует запись или ошибка в базе данных "} ("ALRSTATE")] -> w1068 mode=indexing
                      }
                    }
                  }
                }
                frame condition #1 {
                  n389 = Unbundle By Name(w1086) -> ("AI_SHVR"=w1088:refnum<k21>)
                  n390 = Unbundle By Name(w1087) -> ("AI_reorder_table"=w1082:i32[])
                  n391 = Unbundle By Name(w1086) -> ("CPU_utilization"=w1085:refnum<k21>)
                  n392 = shared-variable-read(w1085) -> (→"CPU %":dbl)  [unwired: 1 in, 3 out]
                  n393 = shared-variable-read(w1088, w1084) -> (w1079:errorcluster, w1089:T4)  [unwired: 2 out]
                  n394 = Unbundle By Name(w1089) -> ("AI"=w1083:dbl[], "AIState"=w1081:T5[], "AIALRState"=w1080:errorcluster[])
                  n395 = case shown="No Error" w1079 {
                    tunnel: w1083 -> [w1097 _]
                    tunnel: w1082 -> [w1096 w1118]
                    tunnel: w1081 -> [w1095 _]
                    tunnel: w1080 -> [w1094 _]
                    tunnel: [w1093 w1117] -> w1078
                    tunnel: [w1092 w1116] -> w1077
                    tunnel: [w1091 w1115] -> w1076
                    frame No Error {
                      n396 = for {
                        tunnel: w1097 -> [w1104]
                        tunnel: w1096 -> [w1100] mode=indexing
                        tunnel: [w1103] -> w1093 mode=indexing
                        tunnel: w1094 -> [w1102]
                        tunnel: [w1101] -> w1092 mode=indexing
                        tunnel: w1095 -> [w1099]
                        tunnel: [w1098] -> w1091 mode=indexing
                        n397 = case shown="0, Default" w1100 {
                          selector: w1100 -> [_ w1108]
                          tunnel: w1104 -> [_ w1114]
                          tunnel: [nan ("PV") w1113] -> w1103
                          tunnel: w1102 -> [_ w1112]
                          tunnel: [T5 {"code"=0, "visible"=FALSE, "color"=14803425, "source"="отсутствует запись или ошибка в базе данных "} ("STATE") w1110] -> w1101
                          tunnel: w1099 -> [_ w1111]
                          tunnel: [errorcluster {"status"=TRUE, "code"=10, "source"="отсутствует запись или ошибка в базе данных "} ("ALRSTATE") w1109] -> w1098
                          frame -1 {
                          }
                          frame 0, Default {
                            n398 = Index Array(array=w1114, index=w1108) -> (element=w1113:dbl)
                            n399 = Index Array(array=w1111, index=w1108) -> (element=w1110:T5)
                            n400 = Index Array(array=w1112, index=w1108) -> (element=w1109:errorcluster)
                          }
                        }
                      }
                    }
                    frame Error {
                      n401 = Array Size(array=w1118) -> (size(s)=w1119:i32)
                      n402 = for {
                        N: w1119 -> [_]
                        tunnel: [nan ("PV")] -> w1117 mode=indexing
                        tunnel: [T5 {"code"=0, "visible"=FALSE, "color"=14803425, "source"="отсутствует запись или ошибка в базе данных "} ("STATE")] -> w1116 mode=indexing
                        tunnel: [errorcluster {"status"=TRUE, "code"=10, "source"="отсутствует запись или ошибка в базе данных "} ("ALRSTATE")] -> w1115 mode=indexing
                      }
                    }
                  }
                }
              }
              n403 = in-place-cluster #2("AI"=w1010, "AIState"=w1009, "AIALRState"=w1008) -> (w1004:T22)
            }
          }
          frame "AIValues" {
            n404 = Unbundle By Name(w1136) -> ("AI_refs"=w1133:refnum<vi>[])
            n405 = Unbundle By Name(w1137) -> ("AI"=w1126:dbl[], "AIState"=w1125:T5[])
            n406 = for {
              tunnel: w1133 -> [w1164] mode=indexing
              tunnel: w1125 -> [w1168] mode=indexing
              shift-right: [w1166] -> w1135
              shift-left: w1134 -> [w1167]
              tunnel: w1126 -> [w1165] mode=indexing
              n407 = Not A Number/Path/Refnum?(number/path/refnum=w1164) -> (NaN/Path/Refnum?=w1163:bool)
              n408 = case shown="False" w1163 {
                tunnel: w1168 -> [w1178 _]
                tunnel: w1167 -> [w1177 w1203]
                tunnel: [w1176 w1203] -> w1166
                tunnel: w1165 -> [w1175 _]
                tunnel: w1164 -> [w1173 _]
                frame False {
                  n409 = Unbundle By Name(w1178) -> ("code"=w1174:i32, "visible"=w1169:bool, "color"=w1171:u32)
                  n410 = case shown="1, Default" w1174 {
                    tunnel: [w1179 u32 16777216 ("Color Box") u32 16718848 ("Color Box") u32 16449346 ("Color Box") u32 16449346 ("Color Box") u32 16718848 ("Color Box") u32 0 ("Color Box") w1199 w1201] -> _
                    tunnel: [FALSE FALSE FALSE FALSE FALSE FALSE TRUE FALSE FALSE] -> w1170
                    tunnel: [w1179 u32 3997440 ("Color Box") u32 16449346 ("Color Box") u32 16718848 ("Color Box") u32 16718848 ("Color Box") u32 16449346 ("Color Box") u32 16772394 ("Color Box") w1199 w1201] -> _
                    frame 0 {
                      w1179 = u32 13816530 ("Color Box")
                    }
                    frame 1, Default {
                    }
                    frame 2 {
                    }
                    frame 3 {
                    }
                    frame 4 {
                    }
                    frame 5 {
                    }
                    frame 6 {
                    }
                    frame 7 {
                      w1199 = u32 13816530 ("Color Box")
                    }
                    frame 8 {
                      w1201 = u32 13816530 ("Color Box")
                    }
                  }
                  n411 = property on="Property Node" class="Slide (strict)"(reference=w1173, error in=w1177, "Value"=w1175, "NumText.TextColor"=u32 3997440 ("Color Box"), "NumText.BGColor"=w1171, "NumText.Visible"=w1169, "Blinking"=w1170) -> (error out=w1176:errorcluster)  [unwired: 1 out]
                }
                frame True {
                }
              }
            }
            n412 = Index Array(array=w1126, index="AI_enum") -> (element=w1131:dbl)
            "EB3BP1_XQ01" <- w1131
            n413 = Index Array(array=w1125, index="AI_enum") -> (element=w1129:T5)
            n414 = Unbundle By Name(w1129) -> ("code"=w1130:i32, "source"=w1127:string, "color"=w1123:u32)
            n415 = case shown="1, Default" w1130 {
              tunnel: [w1139 u32 16777216 ("Color Box") u32 16718848 ("Color Box") u32 16449346 ("Color Box") u32 16449346 ("Color Box") u32 16718848 ("Color Box") u32 0 ("Color Box") w1159 w1161] -> _
              tunnel: [FALSE FALSE FALSE FALSE FALSE FALSE TRUE FALSE FALSE] -> w1128
              tunnel: [w1139 u32 3997440 ("Color Box") u32 16449346 ("Color Box") u32 16718848 ("Color Box") u32 16718848 ("Color Box") u32 16449346 ("Color Box") u32 16772394 ("Color Box") w1159 w1161] -> _
              frame 0 {
                w1139 = u32 13816530 ("Color Box")
              }
              frame 1, Default {
              }
              frame 2 {
              }
              frame 3 {
              }
              frame 4 {
              }
              frame 5 {
              }
              frame 6 {
              }
              frame 7 {
                w1159 = u32 13816530 ("Color Box")
              }
              frame 8 {
                w1161 = u32 13816530 ("Color Box")
              }
            }
            n416 = property on="EB3BP1_XQ01" class="DigNum (strict)"("Value"=w1131, "NumText.TextColor"=u32 3997440 ("Color Box"), "Blinking"=w1128, "TipStrip"=w1127, "NumText.BGColor"=w1123) -> ()  [unwired: 2 in, 2 out]
          }
          frame "Alarms" {
            n417 = in-place {
              in-place-border: w1207 -> [w1219]
              n418 = in-place-cluster #3(w1210) -> ("ALR_State"=w1218:T9, "ALR_Names"=w1213:string[])
              n419 = in-place-match #4(w1208) -> (w1215:errorcluster)
              n420 = disable-structure shown="SERVER==OPC" {
                disable-tunnel: w1219 -> [w1224 w1287]
                disable-tunnel: [w1226 w1285] -> _
                disable-tunnel: w1215 -> [w1245 w1278]
                disable-tunnel: [w1227 w1286] -> w1214
                disable-tunnel: [w1228 w1280] -> w1216
                disable-tunnel: [w1236 w1283] -> w1217
                disable-tunnel: w1218 -> [w1223 w1279]
                disable-tunnel: w1213 -> [_ w1280]
                frame condition #0 (active) {
                  n421 = Unbundle By Name(w1224) -> ("OPC UA.Client refnum"=w1220:T17)
                  n422 = call-poly <vilib>:"Multiple Read.vi"("error in (no error)"=w1245, "node IDs"=T6 ["ns=2;s=ALR.ALR_blocked", "ns=2;s=ALR.ALR_ON"] ("OPC UA.node IDs"), "OPC UA client refnum in"=w1220) -> ("error out"=w1248:errorcluster, "results"=w1247:T69, "OPC UA client refnum out"=w1232:T17, "service status"=w1249:T39)  [unwired: 5 in]
                  n423 = case shown="0..15" w1249 {
                    tunnel: w1248 -> [w1270 w1273]
                    tunnel: [w1270 w1273] -> w1240
                    tunnel: w1247 -> [_ w1276]
                    tunnel: [_ TRUE] -> w1239
                    tunnel: [_ w1274] -> w1222
                    tunnel: [_ w1271] -> w1221
                    frame 16.., Default {
                    }
                    frame 0..15 {
                      n424 = Index Array(array=w1276) -> (element #1=w1277:T70, element #2=w1272:T70)  [unwired: 2 in]
                      n425 = Unbundle By Name(w1277) -> ("values"=w1274:bool[])
                      n426 = Unbundle By Name(w1272) -> ("values"=w1271:bool[])
                    }
                  }
                  n427 = call-poly <vilib>:"Multiple Read.vi"("error in (no error)"=w1240, "node IDs"=T6 ["ns=2;s=ALR.t_ms", "ns=2;s=ALR.ack_state", "ns=2;s=ALR.color"] ("OPC UA.node IDs"), "OPC UA client refnum in"=w1220) -> ("error out"=w1242:errorcluster, "results"=w1243:T71, "service status"=w1241:T39)  [unwired: 5 in, 1 out]
                  n428 = case shown="0..15" w1241 {
                    tunnel: w1242 -> [w1258 w1262]
                    tunnel: [w1258 w1262] -> w1230
                    tunnel: w1243 -> [_ w1268]
                    tunnel: [_ w1267] -> w1238
                    tunnel: w1239 -> [_ w1266]
                    tunnel: [_ w1264] -> w1229
                    tunnel: [_ w1261] -> w1237
                    tunnel: [_ w1259] -> w1225
                    frame 16.., Default {
                    }
                    frame 0..15 {
                      n429 = Index Array(array=w1268) -> (element #1=w1269:T72, element #2=w1263:T72, element #3=w1260:T72)  [unwired: 3 in]
                      n430 = Unbundle By Name(w1269) -> ("values"=w1267:u32[])
                      n431 = Unbundle By Name(w1263) -> ("values"=w1261:u32[])
                      n432 = Unbundle By Name(w1260) -> ("values"=w1259:u32[])
                      n433 = And(x=w1266, y=TRUE) -> (x .and. y?=w1264:bool)
                    }
                  }
                  n434 = call-poly <vilib>:"Multiple Read.vi"("error in (no error)"=w1230, "node IDs"=T6 ["ns=2;s=ALR.ALR_Names"] ("OPC UA.node IDs"), "OPC UA client refnum in"=w1232) -> ("error out"=w1234:errorcluster, "results"=w1235:T40, "service status"=w1233:T39)  [unwired: 5 in, 1 out]
                  n435 = case shown="0..15" w1233 {
                    tunnel: w1234 -> [w1250 w1251]
                    tunnel: [w1250 w1251] -> w1227
                    tunnel: w1235 -> [_ w1256]
                    tunnel: [_ w1255] -> w1228
                    tunnel: w1229 -> [_ w1254]
                    tunnel: [_ w1252] -> w1226
                    frame 16.., Default {
                    }
                    frame 0..15 {
                      n436 = Index Array(array=w1256) -> (element=w1257:T41)  [unwired: 1 in]
                      n437 = Unbundle By Name(w1257) -> ("values"=w1255:string[])
                      n438 = And(x=w1254, y=TRUE) -> (x .and. y?=w1252:bool)
                    }
                  }
                  n439 = Bundle By Name(cluster=w1223, "ALR blocked"=w1222, "ALR ON"=w1221, "t ms"=w1238, "ack state"=w1237, "color"=w1225) -> (w1236:T9)
                }
                frame condition #1 {
                  n440 = Unbundle By Name(w1287) -> ("ALR_state_SHRV"=w1282:refnum<k21>)
                  n441 = shared-variable-read(w1282, w1278) -> (w1284:errorcluster, w1281:T9)  [unwired: 2 out]
                  n442 = case shown="Error .." w1284 {
                    selector: w1284 -> [w1289 w1292]
                    tunnel: [w1290 w1291] -> w1283
                    tunnel: w1281 -> [w1290 _]
                    tunnel: [w1289 w1292] -> w1286
                    tunnel: [TRUE _] -> w1285
                    tunnel: w1279 -> [_ w1291]
                    frame No Error {
                    }
                    frame Error {
                    }
                  }
                }
              }
              n443 = in-place-cluster #3("ALR_State"=w1217, "ALR_Names"=w1216) -> (w1209:T22)
              n444 = in-place-match #4(w1214) -> (w1211:errorcluster)
            }
            n445 = Unbundle By Name(w1209) -> ("ALR_State"=w1206:T9, "ALR_Names"=w1205:string[])
            n446 = Unbundle By Name(w1207) -> ("ALR_Descriptions"=w1204:string[])
            n447 = call "view curr alr state_2.vi"("ALR_Descriptions"=w1204, "ALR_Names"=w1205, "ALR_State"=w1206) -> ()  [unwired: 9 in]
          }
          frame "TB1" {
            n448 = in-place {
              in-place-border: [w1325] -> w1297
              in-place-border: w1319 -> [w1322]
              n449 = in-place-cluster #5(w1315) -> ("TB1_ZY_State"=w1321)
              n450 = in-place-match #6(w1318) -> (w1323:errorcluster)
              n451 = disable-structure shown="SERVER==OPC" {
                disable-tunnel: [w1332 w1349] -> w1325
                disable-tunnel: [w1330 w1352] -> w1320
                disable-tunnel: w1323 -> [w1329 w1354]
                disable-tunnel: [w1328 w1350] -> w1324
                disable-tunnel: w1322 -> [w1327 w1348]
                disable-tunnel: w1321 -> [w1326 w1347]
                frame condition #0 (active) {
                  n452 = Unbundle By Name(w1327) -> ("OPC UA.Client refnum"=w1336:T17)
                  n453 = call-poly <vilib>:"Multiple Read.vi"("error in (no error)"=w1329, "node IDs"=T6 ["ns=2;s=EB2TB1.state"] ("OPC UA.node IDs"), "OPC UA client refnum in"=w1336) -> ("error out"=w1334:errorcluster, "results"=w1333:T58, "service status"=w1335:T39)  [unwired: 5 in, 1 out]
                  n454 = case shown="0..15" w1335 {
                    tunnel: w1334 -> [w1338 w1344]
                    tunnel: [w1338 w1343] -> w1328
                    tunnel: w1333 -> [_ w1342]
                    tunnel: [w1337 w1341] -> w1330
                    tunnel: [_ TRUE] -> w1332
                    tunnel: w1326 -> [w1337 _]
                    frame 16.., Default {
                    }
                    frame 0..15 {
                      n455 = Index Array(array=w1342) -> (element=w1346:T73)  [unwired: 1 in]
                      n456 = Unbundle By Name(w1346) -> ("value"=w1345:string)
                      n457 = call "From JSON Text.vim"("Data Type and Default Value"=T62 {"Z"={"Z_Source"=0, "Z_SetState"=0, "Z_State"=0, "Z_State_T"=0, "ZM_State"=0, "ZM_State_T"=0, "ALR  L1"=FALSE, "ALR  L2"=FALSE, "HH_run"=0}, "Y"={"Y_Source"=0, "Y_SetState"=0, "SP_Set"=0.0, "SP"=0.0, "PV"=0.0, "Y_Set"=0.0, "Y"=0.0, "Y_State"={"code"=0, "visible"=FALSE, "color"=0}, "YB"=FALSE}, "ALR_Status"=[]} ("ZY_State"), "error in (no error)"=w1344, "JSON"=w1345) -> ("error out"=w1343:errorcluster, "Data out"=w1341:T62)  [unwired: 7 in]
                    }
                  }
                }
                frame condition #1 {
                  n458 = Unbundle By Name(w1348) -> ("EB2TB1_state"=w1355)
                  n459 = shared-variable-read(w1355, w1354) -> (w1353:errorcluster, w1351:T74)  [unwired: 2 out]
                  n460 = case shown="No Error" w1353 {
                    selector: w1353 -> [w1357 w1360]
                    tunnel: [w1358 T63 {"Z"={"Z_Source"=enum."initialize", "Z_SetState"=enum."initialization", "Z_State"=enum."initialization", "Z_State_T"=0, "ZM_State"=enum."initialization", "ZM_State_T"=0, "ALR  L1"=FALSE, "ALR  L2"=FALSE, "HH_run"=0}, "Y"={"Y_Source"=enum."initialize", "Y_SetState"=enum."initialize", "SP_Set"=0.0, "SP"=0.0, "PV"=0.0, "Y_Set"=0.0, "Y"=0.0, "Y_State"={"code"=0, "visible"=FALSE, "color"=0}, "YB"=FALSE}, "ALR_Status"=[]} ("AI")] -> w1352
                    tunnel: w1351 -> [w1358 _]
                    tunnel: [w1357 w1360] -> w1350
                    tunnel: [TRUE _] -> w1349
                    tunnel: w1347 -> [_ _]
                    frame No Error {
                    }
                    frame Error {
                    }
                  }
                }
              }
              n461 = in-place-cluster #5("TB1_ZY_State"=w1320) -> (w1296:T22)
              n462 = in-place-match #6(w1324) -> (w1313:errorcluster)
            }
            n463 = disable-structure shown="Enabled" {
              disable-tunnel: [w1363 TRUE ("timer end")] -> w1304
              frame Disabled {
                n464 = property on="Property Node" class="Z_OnSwitch (strict)"() -> ("timer end"=w1363:bool)  [unwired: 2 in, 2 out]
              }
              frame Enabled {
              }
            }
            n465 = Unbundle By Name(w1296) -> ("ALR  L1"=w1317, "ALR  L2"=w1316)
            n466 = Unbundle By Name(w1296) -> ("Y_SetState"=w1295, "Y"=w1294)
            n467 = disable-structure shown="Enabled" {
              disable-tunnel: [w1361 TRUE ("timer end")] -> w1293
              frame Disabled {
                n468 = property on="Property Node" class="YQ2 (strict)"() -> ("timer end"=w1361:bool)  [unwired: 2 in, 2 out]
              }
              frame Enabled {
              }
            }
            n469 = Unbundle By Name(w1296) -> ("Z_Source"=w1306, "Z_State"=w1305)
            n470 = Bundle By Name(cluster=T61 {"connect"=FALSE, "Z_Source"=enum."initialize", "Z_State_heating"=enum."initialization"} ("source"), "connect"=w1297, "Z_Source"=w1306, "Z_State_heating"=w1305) -> (w1307:T61)
            n471 = Bundle By Name(cluster=cluster{"connect":bool, "Y_State":T46, "Y":dbl} {"connect"=FALSE, "Y_State"=enum."initialize", "Y"=0.0} ("source"), "connect"=w1297, "Y_State"=w1295, "Y"=w1294) -> (w1298:cluster{"connect":bool, "Y_State":T46, "Y":dbl})
            n472 = Not(x=w1304) -> (.not. x?=w1311:bool)
            n473 = Not(x=w1293) -> (.not. x?=w1302:bool)
            n474 = call "Is Value Changed.vim"("value"=w1307) -> ("changed or first call?"=w1310:bool)
            n475 = feedback #7() -> (w1312:bool)  [unwired: 1 in]
            n476 = feedback-in #7(w1311) -> ()
            n477 = property on="Property Node" class="Bool (strict)"("Visible"=w1317) -> ()  [unwired: 2 in, 2 out]
            n478 = property on="Property Node" class="Bool (strict)"("Visible"=w1316) -> ()  [unwired: 2 in, 2 out]
            n479 = call "Is Value Changed.vim"("value"=w1298) -> ("changed or first call?"=w1301:bool)
            n480 = feedback #8() -> (w1303:bool)  [unwired: 1 in]
            n481 = feedback-in #8(w1302) -> ()
            n482 = Compound Arithmetic op=OR(w1310, w1311, w1312) -> (w1308:bool)
            n483 = Compound Arithmetic op=OR(w1301, w1302, w1303) -> (w1299:bool)
            n484 = case shown="True" w1308 {
              tunnel: w1307 -> [_ w1365]
              frame False {
              }
              frame True {
                n485 = property on="Property Node" class="Z_OnSwitch (strict)"("State"=w1365) -> ()  [unwired: 2 in, 2 out]
              }
            }
            n486 = case shown="True" w1299 {
              tunnel: w1298 -> [_ w1366]
              frame False {
              }
              frame True {
                n487 = property on="Property Node" class="YQ2 (strict)"("State"=w1366) -> ()  [unwired: 2 in, 2 out]
              }
            }
          }
          frame "TB2" {
            n488 = in-place {
              in-place-border: [w1399] -> w1369
              in-place-border: w1393 -> [w1396]
              n489 = in-place-cluster #9(w1388) -> ("TB2_ZY_State"=w1395)
              n490 = in-place-match #10(w1392) -> (w1397:errorcluster)
              n491 = disable-structure shown="SERVER==OPC" {
                disable-tunnel: [w1406 w1423] -> w1399
                disable-tunnel: [w1404 w1426] -> w1394
                disable-tunnel: w1397 -> [w1403 w1428]
                disable-tunnel: [w1402 w1424] -> w1398
                disable-tunnel: w1396 -> [w1401 w1422]
                disable-tunnel: w1395 -> [w1400 w1421]
                frame condition #0 (active) {
                  n492 = Unbundle By Name(w1401) -> ("OPC UA.Client refnum"=w1410:T17)
                  n493 = call-poly <vilib>:"Multiple Read.vi"("error in (no error)"=w1403, "node IDs"=T6 ["ns=2;s=EB2TB2.state"] ("OPC UA.node IDs"), "OPC UA client refnum in"=w1410) -> ("error out"=w1408:errorcluster, "results"=w1407:T58, "service status"=w1409:T39)  [unwired: 5 in, 1 out]
                  n494 = case shown="0..15" w1409 {
                    tunnel: w1408 -> [w1412 w1418]
                    tunnel: [w1412 w1417] -> w1402
                    tunnel: w1407 -> [_ w1416]
                    tunnel: [w1411 w1415] -> w1404
                    tunnel: [_ TRUE] -> w1406
                    tunnel: w1400 -> [w1411 _]
                    frame 16.., Default {
                    }
                    frame 0..15 {
                      n495 = Index Array(array=w1416) -> (element=w1420:T73)  [unwired: 1 in]
                      n496 = Unbundle By Name(w1420) -> ("value"=w1419:string)
                      n497 = call "From JSON Text.vim"("Data Type and Default Value"=T62 {"Z"={"Z_Source"=0, "Z_SetState"=0, "Z_State"=0, "Z_State_T"=0, "ZM_State"=0, "ZM_State_T"=0, "ALR  L1"=FALSE, "ALR  L2"=FALSE, "HH_run"=0}, "Y"={"Y_Source"=0, "Y_SetState"=0, "SP_Set"=0.0, "SP"=0.0, "PV"=0.0, "Y_Set"=0.0, "Y"=0.0, "Y_State"={"code"=0, "visible"=FALSE, "color"=0}, "YB"=FALSE}, "ALR_Status"=[]} ("ZY_State"), "error in (no error)"=w1418, "JSON"=w1419) -> ("error out"=w1417:errorcluster, "Data out"=w1415:T62)  [unwired: 7 in]
                    }
                  }
                }
                frame condition #1 {
                  n498 = Unbundle By Name(w1422) -> ("EB2TB2_state"=w1429)
                  n499 = shared-variable-read(w1429, w1428) -> (w1427:errorcluster, w1425:T74)  [unwired: 2 out]
                  n500 = case shown="No Error" w1427 {
                    selector: w1427 -> [w1431 w1434]
                    tunnel: [w1432 T63 {"Z"={"Z_Source"=enum."initialize", "Z_SetState"=enum."initialization", "Z_State"=enum."initialization", "Z_State_T"=0, "ZM_State"=enum."initialization", "ZM_State_T"=0, "ALR  L1"=FALSE, "ALR  L2"=FALSE, "HH_run"=0}, "Y"={"Y_Source"=enum."initialize", "Y_SetState"=enum."initialize", "SP_Set"=0.0, "SP"=0.0, "PV"=0.0, "Y_Set"=0.0, "Y"=0.0, "Y_State"={"code"=0, "visible"=FALSE, "color"=0}, "YB"=FALSE}, "ALR_Status"=[]} ("AI")] -> w1426
                    tunnel: w1425 -> [w1432 _]
                    tunnel: [w1431 w1434] -> w1424
                    tunnel: [TRUE _] -> w1423
                    tunnel: w1421 -> [_ _]
                    frame No Error {
                    }
                    frame Error {
                    }
                  }
                }
              }
              n501 = in-place-cluster #9("TB2_ZY_State"=w1394) -> (w1389:T22)
              n502 = in-place-match #10(w1398) -> (w1386:errorcluster)
            }
            n503 = disable-structure shown="Enabled" {
              disable-tunnel: [w1435 TRUE ("timer end")] -> w1377
              frame Disabled {
                n504 = property on="Property Node" class="Z_OnSwitch (strict)"() -> ("timer end"=w1435:bool)  [unwired: 2 in, 2 out]
              }
              frame Enabled {
              }
            }
            n505 = Unbundle By Name(w1389) -> ("Y_SetState"=w1370, "Y"=w1368)
            n506 = disable-structure shown="Enabled" {
              disable-tunnel: [w1437 TRUE ("timer end")] -> w1367
              frame Disabled {
                n507 = property on="Property Node" class="YQ2 (strict)"() -> ("timer end"=w1437:bool)  [unwired: 2 in, 2 out]
              }
              frame Enabled {
              }
            }
            n508 = Unbundle By Name(w1389) -> ("ALR  L1"=w1391, "ALR  L2"=w1390)
            n509 = Unbundle By Name(w1389) -> ("Z_Source"=w1379, "Z_State"=w1378)
            n510 = Bundle By Name(cluster=cluster{"connect":bool, "Y_State":T46, "Y":dbl} {"connect"=FALSE, "Y_State"=enum."initialize", "Y"=0.0} ("source"), "connect"=w1369, "Y_State"=w1370, "Y"=w1368) -> (w1371:cluster{"connect":bool, "Y_State":T46, "Y":dbl})
            n511 = Bundle By Name(cluster=T61 {"connect"=FALSE, "Z_Source"=enum."initialize", "Z_State_heating"=enum."initialization"} ("source"), "connect"=w1369, "Z_Source"=w1379, "Z_State_heating"=w1378) -> (w1380:T61)
            n512 = Not(x=w1367) -> (.not. x?=w1375:bool)
            n513 = Not(x=w1377) -> (.not. x?=w1384:bool)
            n514 = property on="Property Node" class="Bool (strict)"("Visible"=w1391) -> ()  [unwired: 2 in, 2 out]
            n515 = property on="Property Node" class="Bool (strict)"("Visible"=w1390) -> ()  [unwired: 2 in, 2 out]
            n516 = call "Is Value Changed.vim"("value"=w1371) -> ("changed or first call?"=w1374:bool)
            n517 = feedback #11() -> (w1376:bool)  [unwired: 1 in]
            n518 = feedback-in #11(w1375) -> ()
            n519 = call "Is Value Changed.vim"("value"=w1380) -> ("changed or first call?"=w1383:bool)
            n520 = feedback #12() -> (w1385:bool)  [unwired: 1 in]
            n521 = feedback-in #12(w1384) -> ()
            n522 = Compound Arithmetic op=OR(w1374, w1375, w1376) -> (w1372:bool)
            n523 = Compound Arithmetic op=OR(w1383, w1384, w1385) -> (w1381:bool)
            n524 = case shown="True" w1381 {
              tunnel: w1380 -> [_ w1439]
              frame False {
              }
              frame True {
                n525 = property on="Property Node" class="Z_OnSwitch (strict)"("State"=w1439) -> ()  [unwired: 2 in, 2 out]
              }
            }
            n526 = case shown="True" w1372 {
              tunnel: w1371 -> [_ w1440]
              frame False {
              }
              frame True {
                n527 = property on="Property Node" class="YQ2 (strict)"("State"=w1440) -> ()  [unwired: 2 in, 2 out]
              }
            }
          }
          frame "TB3" {
            n528 = in-place {
              in-place-border: [w1473] -> w1442
              in-place-border: w1467 -> [w1470]
              n529 = in-place-cluster #13(w1465) -> ("TB3_ZY_State"=w1469)
              n530 = in-place-match #14(w1466) -> (w1471:errorcluster)
              n531 = disable-structure shown="SERVER==OPC" {
                disable-tunnel: [w1480 w1497] -> w1473
                disable-tunnel: [w1478 w1500] -> w1468
                disable-tunnel: w1471 -> [w1477 w1502]
                disable-tunnel: [w1476 w1498] -> w1472
                disable-tunnel: w1470 -> [w1475 w1496]
                disable-tunnel: w1469 -> [w1474 w1495]
                frame condition #0 (active) {
                  n532 = Unbundle By Name(w1475) -> ("OPC UA.Client refnum"=w1484:T17)
                  n533 = call-poly <vilib>:"Multiple Read.vi"("error in (no error)"=w1477, "node IDs"=T6 ["ns=2;s=EB2TB3.state"] ("OPC UA.node IDs"), "OPC UA client refnum in"=w1484) -> ("error out"=w1482:errorcluster, "results"=w1481:T58, "service status"=w1483:T39)  [unwired: 5 in, 1 out]
                  n534 = case shown="0..15" w1483 {
                    tunnel: w1482 -> [w1486 w1492]
                    tunnel: [w1486 w1491] -> w1476
                    tunnel: w1481 -> [_ w1490]
                    tunnel: [w1485 w1489] -> w1478
                    tunnel: [_ TRUE] -> w1480
                    tunnel: w1474 -> [w1485 _]
                    frame 16.., Default {
                    }
                    frame 0..15 {
                      n535 = Index Array(array=w1490) -> (element=w1494:T73)  [unwired: 1 in]
                      n536 = Unbundle By Name(w1494) -> ("value"=w1493:string)
                      n537 = call "From JSON Text.vim"("Data Type and Default Value"=T62 {"Z"={"Z_Source"=0, "Z_SetState"=0, "Z_State"=0, "Z_State_T"=0, "ZM_State"=0, "ZM_State_T"=0, "ALR  L1"=FALSE, "ALR  L2"=FALSE, "HH_run"=0}, "Y"={"Y_Source"=0, "Y_SetState"=0, "SP_Set"=0.0, "SP"=0.0, "PV"=0.0, "Y_Set"=0.0, "Y"=0.0, "Y_State"={"code"=0, "visible"=FALSE, "color"=0}, "YB"=FALSE}, "ALR_Status"=[]} ("ZY_State"), "error in (no error)"=w1492, "JSON"=w1493) -> ("error out"=w1491:errorcluster, "Data out"=w1489:T62)  [unwired: 7 in]
                    }
                  }
                }
                frame condition #1 {
                  n538 = Unbundle By Name(w1496) -> ("EB2TB3_state"=w1503)
                  n539 = shared-variable-read(w1503, w1502) -> (w1501:errorcluster, w1499:T74)  [unwired: 2 out]
                  n540 = case shown="Error .." w1501 {
                    selector: w1501 -> [w1505 w1508]
                    tunnel: [w1506 T63 {"Z"={"Z_Source"=enum."initialize", "Z_SetState"=enum."initialization", "Z_State"=enum."initialization", "Z_State_T"=0, "ZM_State"=enum."initialization", "ZM_State_T"=0, "ALR  L1"=FALSE, "ALR  L2"=FALSE, "HH_run"=0}, "Y"={"Y_Source"=enum."initialize", "Y_SetState"=enum."initialize", "SP_Set"=0.0, "SP"=0.0, "PV"=0.0, "Y_Set"=0.0, "Y"=0.0, "Y_State"={"code"=0, "visible"=FALSE, "color"=0}, "YB"=FALSE}, "ALR_Status"=[]} ("AI")] -> w1500
                    tunnel: w1499 -> [w1506 _]
                    tunnel: [w1505 w1508] -> w1498
                    tunnel: [TRUE _] -> w1497
                    tunnel: w1495 -> [_ _]
                    frame No Error {
                    }
                    frame Error {
                    }
                  }
                }
              }
              n541 = in-place-cluster #13("TB3_ZY_State"=w1468) -> (w1463:T22)
              n542 = in-place-match #14(w1472) -> (w1460:errorcluster)
            }
            n543 = disable-structure shown="Enabled" {
              disable-tunnel: [w1509 TRUE ("timer end")] -> w1451
              frame Disabled {
                n544 = property on="Property Node" class="Z_OnSwitch (strict)"() -> ("timer end"=w1509:bool)  [unwired: 2 in, 2 out]
              }
              frame Enabled {
              }
            }
            n545 = Unbundle By Name(w1463) -> ("Y_SetState"=w1444, "Y"=w1443)
            n546 = Unbundle By Name(w1463) -> ("ALR  L1"=w1462, "ALR  L2"=w1461)
            n547 = disable-structure shown="Enabled" {
              disable-tunnel: [w1511 TRUE ("timer end")] -> w1441
              frame Disabled {
                n548 = property on="Property Node" class="YQ2 (strict)"() -> ("timer end"=w1511:bool)  [unwired: 2 in, 2 out]
              }
              frame Enabled {
              }
            }
            n549 = Unbundle By Name(w1463) -> ("Z_Source"=w1453, "Z_State"=w1452)
            n550 = Bundle By Name(cluster=cluster{"connect":bool, "Y_State":T46, "Y":dbl} {"connect"=FALSE, "Y_State"=enum."initialize", "Y"=0.0} ("source"), "connect"=w1442, "Y_State"=w1444, "Y"=w1443) -> (w1445:cluster{"connect":bool, "Y_State":T46, "Y":dbl})
            n551 = Bundle By Name(cluster=T61 {"connect"=FALSE, "Z_Source"=enum."initialize", "Z_State_heating"=enum."initialization"} ("source"), "connect"=w1442, "Z_Source"=w1453, "Z_State_heating"=w1452) -> (w1454:T61)
            n552 = Not(x=w1441) -> (.not. x?=w1449:bool)
            n553 = Not(x=w1451) -> (.not. x?=w1458:bool)
            n554 = property on="Property Node" class="Bool (strict)"("Visible"=w1462) -> ()  [unwired: 2 in, 2 out]
            n555 = property on="Property Node" class="Bool (strict)"("Visible"=w1461) -> ()  [unwired: 2 in, 2 out]
            n556 = call "Is Value Changed.vim"("value"=w1445) -> ("changed or first call?"=w1448:bool)
            n557 = feedback #15() -> (w1450:bool)  [unwired: 1 in]
            n558 = feedback-in #15(w1449) -> ()
            n559 = call "Is Value Changed.vim"("value"=w1454) -> ("changed or first call?"=w1457:bool)
            n560 = feedback #16() -> (w1459:bool)  [unwired: 1 in]
            n561 = feedback-in #16(w1458) -> ()
            n562 = Compound Arithmetic op=OR(w1448, w1449, w1450) -> (w1446:bool)
            n563 = Compound Arithmetic op=OR(w1457, w1458, w1459) -> (w1455:bool)
            n564 = case shown="True" w1455 {
              tunnel: w1454 -> [_ w1513]
              frame False {
              }
              frame True {
                n565 = property on="Property Node" class="Z_OnSwitch (strict)"("State"=w1513) -> ()  [unwired: 2 in, 2 out]
              }
            }
            n566 = case shown="True" w1446 {
              tunnel: w1445 -> [_ w1514]
              frame False {
              }
              frame True {
                n567 = property on="Property Node" class="YQ2 (strict)"("State"=w1514) -> ()  [unwired: 2 in, 2 out]
              }
            }
          }
          frame "Exit" {
            n568 = local read "Останов\nпрограммы"() -> (w1518:bool)
          }
        }
        n569 = Wait Until Next ms Multiple(millisecond multiple=w919) -> ()  [unwired: 1 out]
      }
    }
    frame Enabled {
    }
  }
  n570 = Unregister For Events(event registration refnum=w13) -> ()  [unwired: 1 in, 1 out]
  n571 = disable-structure shown="Disabled" {
    disable-tunnel: w16 -> [w1521 _]
    frame Disabled {
      n572 = invoke class="VI" method="FP.Close"(reference=w1521) -> ()  [unwired: 2 in, 3 out]
    }
    frame Enabled {
    }
  }
  n573 = flat-sequence {
    tunnel: w8 -> [w1529]
    tunnel: w7 -> [w1527]
    tunnel: w7 -> [w1526]
    tunnel: w4 -> [w1523]
    frame #0 {
      n574 = disable-structure shown="SERVER==OPC" {
        disable-tunnel: w1523 -> [w1551 w1579]
        disable-tunnel: [w1565 w1571] -> w1522
        frame condition #0 {
          n575 = Unbundle By Name(w1551) -> ("EB2TB3_control"=w1550, "EB2TB3_state"=w1549, "EB3TB1_control"=w1548, "EB3TB1_state"=w1547, "EB3TB2_control"=w1546, "EB3TB2_state"=w1545, "EB3TB3_control"=w1544, "EB3TB3_state"=w1543)
          n576 = Close Variable Connection(11:w1550) -> (0:w1540:errorcluster)  [unwired: 1 in]
          n577 = Close Variable Connection(11:w1549) -> (0:w1539:errorcluster)  [unwired: 1 in]
          n578 = Close Variable Connection(11:w1548) -> (0:w1538:errorcluster)  [unwired: 1 in]
          n579 = Close Variable Connection(11:w1547) -> (0:w1537:errorcluster)  [unwired: 1 in]
          n580 = Close Variable Connection(11:w1546) -> (0:w1536:errorcluster)  [unwired: 1 in]
          n581 = Close Variable Connection(11:w1545) -> (0:w1535:errorcluster)  [unwired: 1 in]
          n582 = Close Variable Connection(11:w1544) -> (0:w1534:errorcluster)  [unwired: 1 in]
          n583 = Close Variable Connection(11:w1543) -> (0:w1533:errorcluster)  [unwired: 1 in]
          n584 = Merge Errors(w1540, w1539, w1538, w1537, w1536, w1535, w1534, w1533) -> (w1532:errorcluster)
          n585 = Unbundle By Name(w1551) -> ("AI_SHVR"=w1570:refnum<k21>, "AI_Names_SHVR"=w1569:refnum<k21>, "DI_SHVR"=w1568:refnum<k21>, "DI_Names_SHVR"=w1567:refnum<k21>, "ALR_state_SHRV"=w1561:refnum<k21>, "ALR_Descriptions_SHRV"=w1560:refnum<k21>, "EB2TB1_control"=w1555, "EB2TB1_state"=w1554, "EB2TB2_control"=w1553, "EB2TB2_state"=w1552)
          n586 = Close Variable Connection(11:w1570) -> (0:w1566:errorcluster)  [unwired: 1 in]
          n587 = Close Variable Connection(11:w1569) -> (0:w1564:errorcluster)  [unwired: 1 in]
          n588 = Close Variable Connection(11:w1568) -> (0:w1563:errorcluster)  [unwired: 1 in]
          n589 = Close Variable Connection(11:w1567) -> (0:w1562:errorcluster)  [unwired: 1 in]
          n590 = Close Variable Connection(11:w1561) -> (0:w1559:errorcluster)  [unwired: 1 in]
          n591 = Close Variable Connection(11:w1560) -> (0:w1558:errorcluster)  [unwired: 1 in]
          n592 = Close Variable Connection(11:w1555) -> (0:w1557:errorcluster)  [unwired: 1 in]
          n593 = Close Variable Connection(11:w1554) -> (0:w1556:errorcluster)  [unwired: 1 in]
          n594 = Close Variable Connection(11:w1553) -> (0:w1542:errorcluster)  [unwired: 1 in]
          n595 = Close Variable Connection(11:w1552) -> (0:w1541:errorcluster)  [unwired: 1 in]
          n596 = Merge Errors(w1566, w1564, w1563, w1562, w1559, w1558, w1557, w1556, w1542, w1541, w1532) -> (w1565:errorcluster)
        }
        frame condition #1 (active) {
          # "7."
          # "8."
          # "6."
          n597 = Unbundle By Name(w1579) -> ("OPC UA.subscription IDs"=w1576:T18[], "OPC UA.Client refnum"=w1578:T17, "OPC UA.node IDs"=w1577:T6, "OPC UA.data change event"=w1574:refnum<user-event>)
          n598 = Destroy User Event(user event=w1574) -> (error out=w1572:errorcluster)  [unwired: 1 in]
          n599 = Index Array(array=w1576) -> (element=w1575:T18)  [unwired: 1 in]
          n600 = call <vilib>:"Delete Monitored Nodes.vi"("node IDs"=w1577, "subscription ID in"=w1575, "OPC UA client refnum in"=w1578) -> ("error out"=w1581:errorcluster, "OPC UA client refnum out"=w1580:T17)  [unwired: 4 in, 3 out]
          n601 = call <vilib>:"Delete Subscriptions.vi"("error in (no error)"=w1581, "subscription IDs"=w1576, "OPC UA client refnum in"=w1580) -> ("error out"=w1583:errorcluster, "OPC UA client refnum out"=w1582:T17)  [unwired: 6 in, 1 out]
          n602 = call <vilib>:"Disconnect.vi"("error in (no error)"=w1583, "OPC UA client refnum in"=w1582) -> ("error out"=w1573:errorcluster)  [unwired: 9 in]
          n603 = Merge Errors(w1573, w1572) -> (w1571:errorcluster)
        }
      }
      n604 = Unbundle By Name(w1523) -> ("AI_refs"=w1524:refnum<vi>[])
      n605 = Merge Errors(w1522, w1526, w1527, w1529) -> (w1528:errorcluster)
      n606 = call <vilib>:"Simple Error Handler.vi"("error in (no error)"=w1528) -> ()  [unwired: 4 in, 5 out]
      n607 = disable-structure shown="Disabled" {
        frame Disabled {
          n608 = property class="App"() -> (error out=w1530:errorcluster, "App.Kind"=w1531:T76)  [unwired: 2 in, 1 out]
          n609 = case shown="\"Run Time System\"" w1531 {
            tunnel: w1530 -> [_ _]
            frame Default {
            }
            frame "Run Time System" {
              n610 = Quit LabVIEW() -> ()  [unwired: 1 in]
            }
          }
        }
        frame Enabled {
        }
      }
      n611 = for {
        tunnel: w1524 -> [w1585] mode=indexing
        n612 = Not A Number/Path/Refnum?(number/path/refnum=w1585) -> (NaN/Path/Refnum?=w1584:bool)
        n613 = case shown="False" w1584 {
          tunnel: w1585 -> [w1586 _]
          frame False {
            n614 = Close Reference(reference=w1586) -> ()  [unwired: 1 in, 1 out]
          }
          frame True {
          }
        }
      }
      n615 = local write "Останов\nпрограммы"(FALSE ("stop")) -> ()
    }
  }
